vi "FPGA Beam Scanning V2.vi"(1 "Detectors":T1, 2 "Image Acquisition Parameters":T2={"Scan Type"=enum."Sample Scanning", "Scan Mode"=enum."XY", "Fast Axis Frequency (Hz)"=100.0, "Image Format"=128, "Line Accumulations"=1, "Frames Per Capture"=1, "Frames Accumulations"=1, "Image Dimension (um)"=[], "Number of Z Steps"=1, "Z Steps Size (um)"=1.0, "Pixel Size (nm)"=[]} {"Z Steps Size (um)" min=0.0; "Number of Z Steps" min=1; "Frames Accumulations" min=1; "Frames Per Capture" min=1; "Line Accumulations" min=1; "Image Format" items=["64 x 64"=64, "128 x 128"=128, "256 x 256"=256, "512 x 512"=512, "1024 x 1024"=1024, "2048 x 2048"=2048]}) -> ()   [LabVIEW 2016]
uses:
  <vilib>/rvi/interface/nirviReadWriteControl/nirviReadWriteControl.xnode
  <vilib>/rvi/interface/nirviMethod/nirviMethod.xnode
  <vilib>/rvi/errors/niLvFpgaMergeErrorWithErrorCode.vi
  <vilib>/rvi/interface/nirviOpenFPGA/nirviOpenFPGA.xnode
  <vilib>/vision/NI_Vision_Development_Module.lvlib
  <vilib>/rvi/interface/nirviCloseFPGA/nirviCloseFPGA.xnode
  <vilib>/vision/Image Controls.llb/IMAQ Image.ctl
  FPGA Bitfiles/MainSTEDFPGAProj_FPGATarget2_BeamScanningCamb_PyGckhW3v70.lvbitx
  FPGA Target VIs/FPGA-7852R/Beam Scanning Cambridge V1.vi
  NiFpgaLv.dll
  <vilib>/Utility/error.llb/Error Cluster From Error Code.vi
  <vilib>/rvi/errors/niLvFpgaAdjustHostInterfaceError.vi
  <vilib>/FPGAPlugInAG/PCIe-7852R/niLvFpga_ReadFifo_PCIe-7852R.vi
  <vilib>/FPGAPlugInAG/PCIe-7852R/niLvFpga_Close_PCIe-7852R.vi
  <vilib>/FPGAPlugInAG/PCIe-7852R/niLvFpga_Open_PCIe-7852R.vi
  <vilib>/FPGAPlugInAG/PCIe-7852R/niLvFpga_ConfigureFifo_PCIe-7852R.vi
  <vilib>/FPGAPlugInAG/PCIe-7852R/niLvFpga_StartFifo_PCIe-7852R.vi
  <vilib>/FPGAPlugInAG/PCIe-7852R/niLvFpga_Run_PCIe-7852R.vi
  Type Defs/Image Acquisition Parameters.ctl
  Detectors.ctl
panel:
  in  "Adjust Trigger":u16=300
  # "Copyright (C) 2020 Edward S Allgeyer\n\nRedistribution and use in source and binary forms, with or without\nmodification, are permitted provided that the following conditions\nare met:\n\n1. Redistributions of source code must retain the above copyright\n   notice, this list of conditions and the following disclaimer.\n\n2. Redistributions in binary form must reproduce the above copyright\n   notice, this list of conditions and the following disclaimer in\n   the documentation and/or other materials provided with the\n   distribution.\n\n3. Neither the name of the copyright holder nor the names of its\n   contributors may be used to endorse or promote products derived\n   from this software without specific prior written permission.\n\nTHIS SOFTWARE IS PROVIDED BY THE COPYRIGHT HOLDERS AND CONTRIBUTORS\n\"AS IS\" AND ANY EXPRESS OR IMPLIED WARRANTIES, INCLUDING, BUT NOT\nLIMITED TO, THE IMPLIED WARRANTIES OF MERCHANTABILITY AND FITNESS\nFOR A PARTICULAR PURPOSE ARE DISCLAIMED. IN NO EVENT SHALL THE\nCOPYRIGHT HOLDER OR CONTRIBUTORS BE LIABLE FOR ANY DIRECT, INDIRECT,\nINCIDENTAL, SPECIAL, EXEMPLARY, OR CONSEQUENTIAL DAMAGES (INCLUDING,\nBUT NOT LIMITED TO, PROCUREMENT OF SUBSTITUTE GOODS OR SERVICES;\nLOSS OF USE, DATA, OR PROFITS; OR BUSINESS INTERRUPTION) HOWEVER\nCAUSED AND ON ANY THEORY OF LIABILITY, WHETHER IN CONTRACT, STRICT\nLIABILITY, OR TORT (INCLUDING NEGLIGENCE OR OTHERWISE) ARISING IN\nANY WAY OUT OF THE USE OF THIS SOFTWARE, EVEN IF ADVISED OF THE\nPOSSIBILITY OF SUCH DAMAGE."
  # "XY"
  # "Z"
  # "Length"
  # "Height"
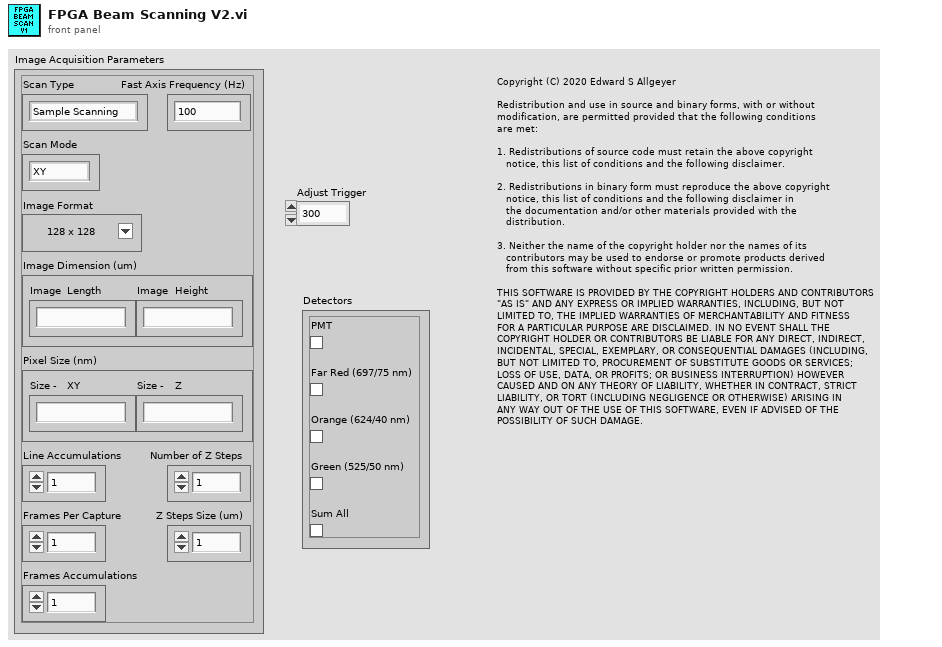
[diagram p1: front panel]
types:
  T1 = typedef "Detectors.ctl" = cluster{"PMT":bool, "Far Red (697/75 nm)":bool, "Orange (624/40 nm)":bool, "Green (525/50 nm)":bool, "Sum All":bool}
  T2 = typedef "Image Acquisition Parameters.ctl" = cluster{"Scan Type":enum16{"Sample Scanning", "Beam Scanning"}, "Scan Mode":enum16{"XY", "XZ", "YZ", "XYZ"}, "Fast Axis Frequency (Hz)":dbl, "Image Format":u16, "Line Accumulations":u16, "Frames Per Capture":u16, "Frames Accumulations":u16, "Image Dimension (um)":dbl[], "Number of Z Steps":u8, "Z Steps Size (um)":dbl, "Pixel Size (nm)":dbl[]}
  T3 = typedef "IMAQ Image.ctl" = refnum<image>
  T4 = enum16{"big-endian, network order", "native, host order", "little-endian"}
  T5 = cluster{"FPGA Sampling Period (ns)":dbl, "Counting Period (us)":dbl, "Samples Per Counting Period":i32, "Start Time (us)":dbl, "Stop Time (us)":dbl, "Normalized Scan End Position":dbl, "Normalized Scan Start Position":dbl}
  T6 = typedef "Scan Parameters.ctl" = cluster{"Fast_Ax_Amp_V":dbl, "Fast_Ax_Off_V":dbl, "Slow_Ax_Amp_V":dbl, "Slow_Ax_Off_V ":dbl, "Slow_Ax_Max_V_VperS":dbl, "Slow_Ax1_Del25ns":i32, "Slow_Ax2_Del25ns":i32, "Stage_X_Off_V":dbl, "Stage_Y_Off_V":dbl, "Stage_Z_Off_V":dbl, "Galvo1_Off_V":dbl, "Galvo2_Off_V":dbl, "Last_Scan_Mode":enum16{"XY", "XZ", "YZ", "XYZ"}, "Current_Scan_Mode":enum16{"XY", "XZ", "YZ", "XYZ"}, "Fly_Back_Lines":u16, "Linear_Ramp_End":u32, "Z_Step_I16":i16, "Z_Start_I16":i16, "Laser_States _U32":u32, "590_Voltage_I16":i16, "775_AOM_Volt_I16":i16, "Blanking OFF":bool, "Unused_Axis_I16":i16}
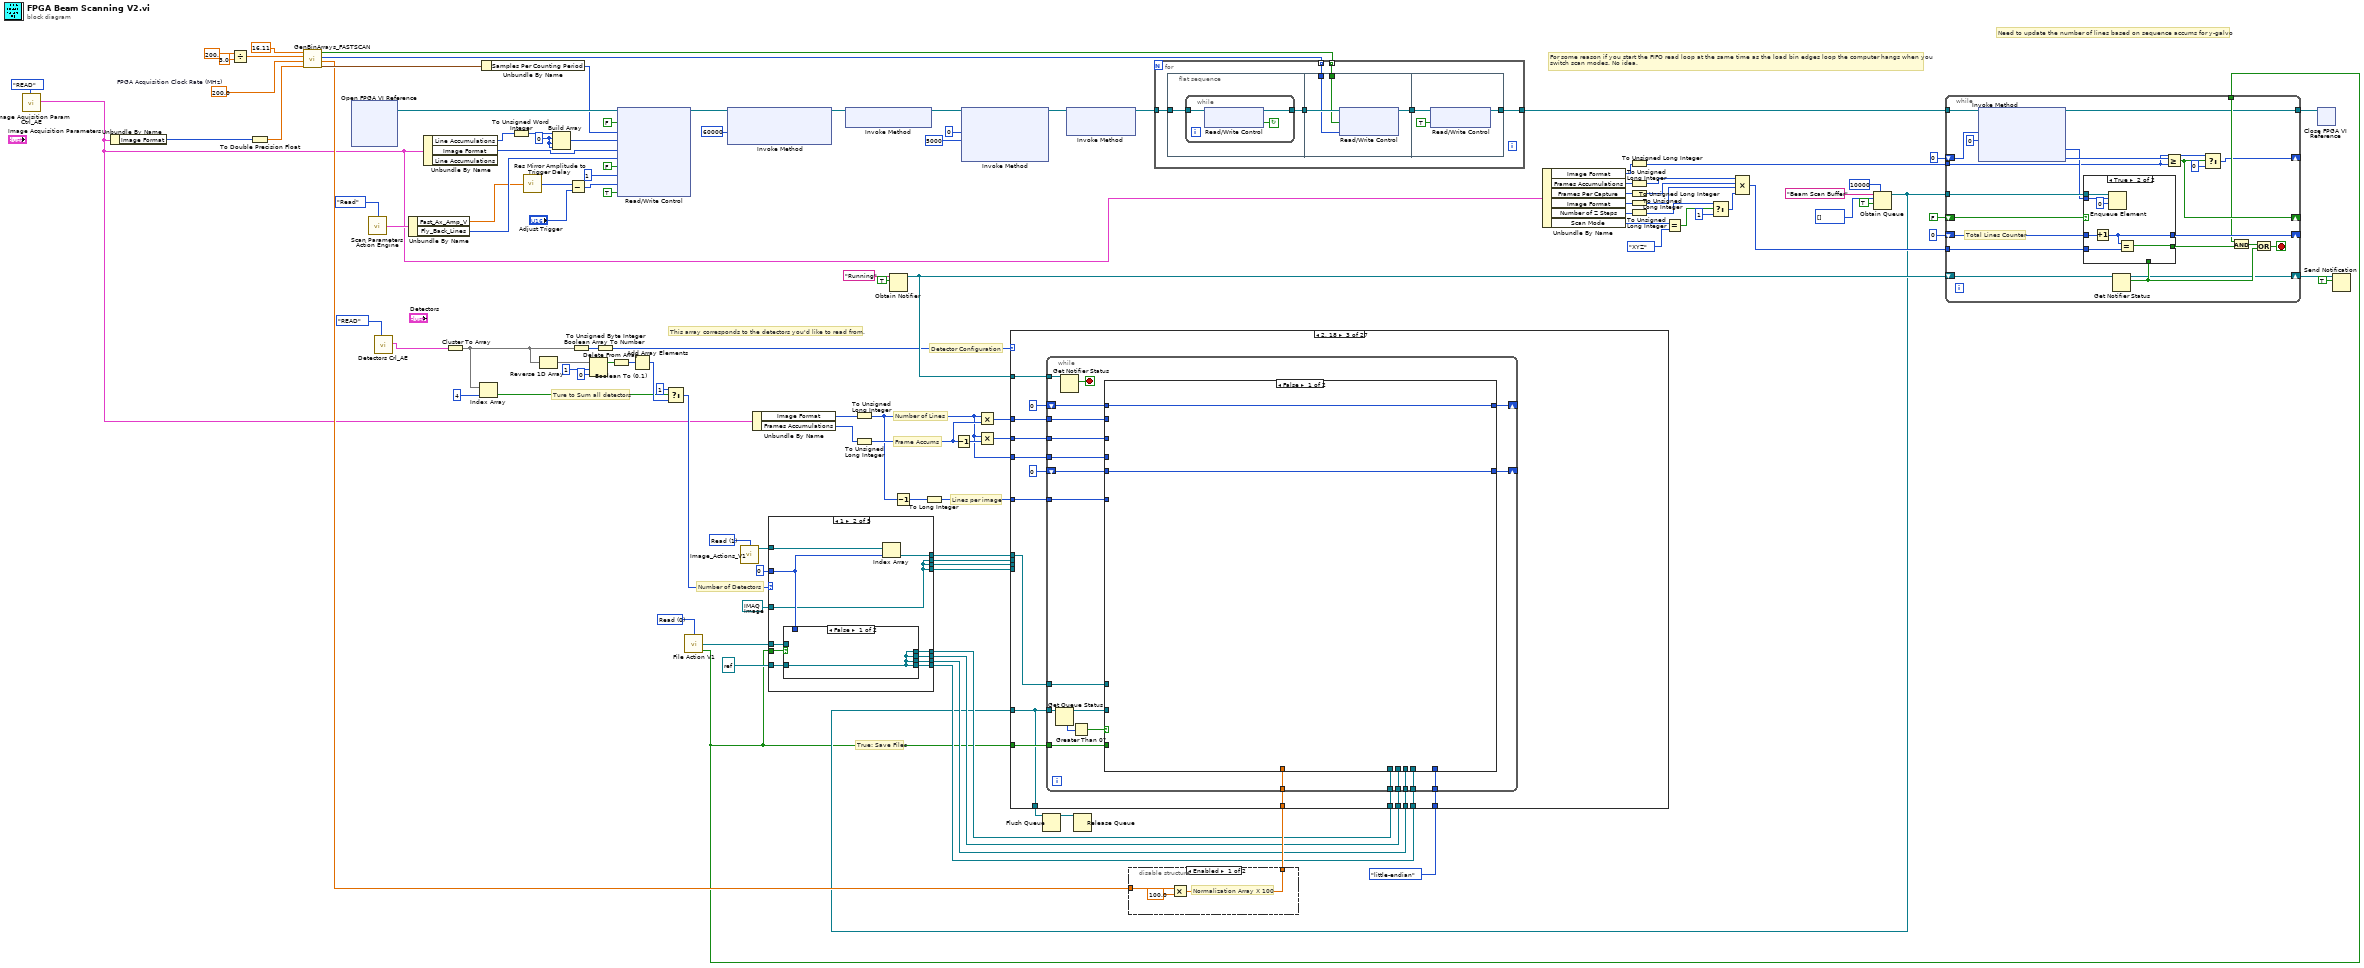
[diagram p0: block diagram]
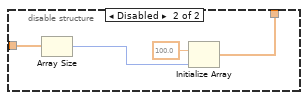
[diagram p2: hidden frame]
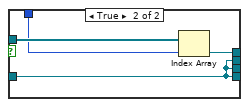
[diagram p4: hidden frame]
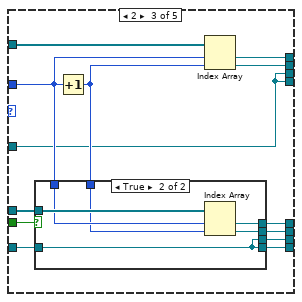
[diagram p5: hidden frame]
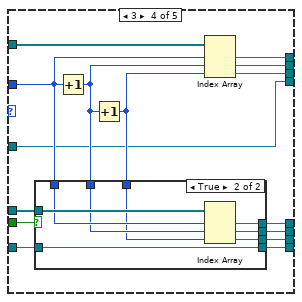
[diagram p7: hidden frame]
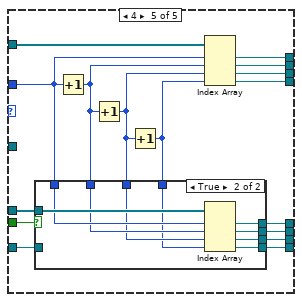
[diagram p9: hidden frame]
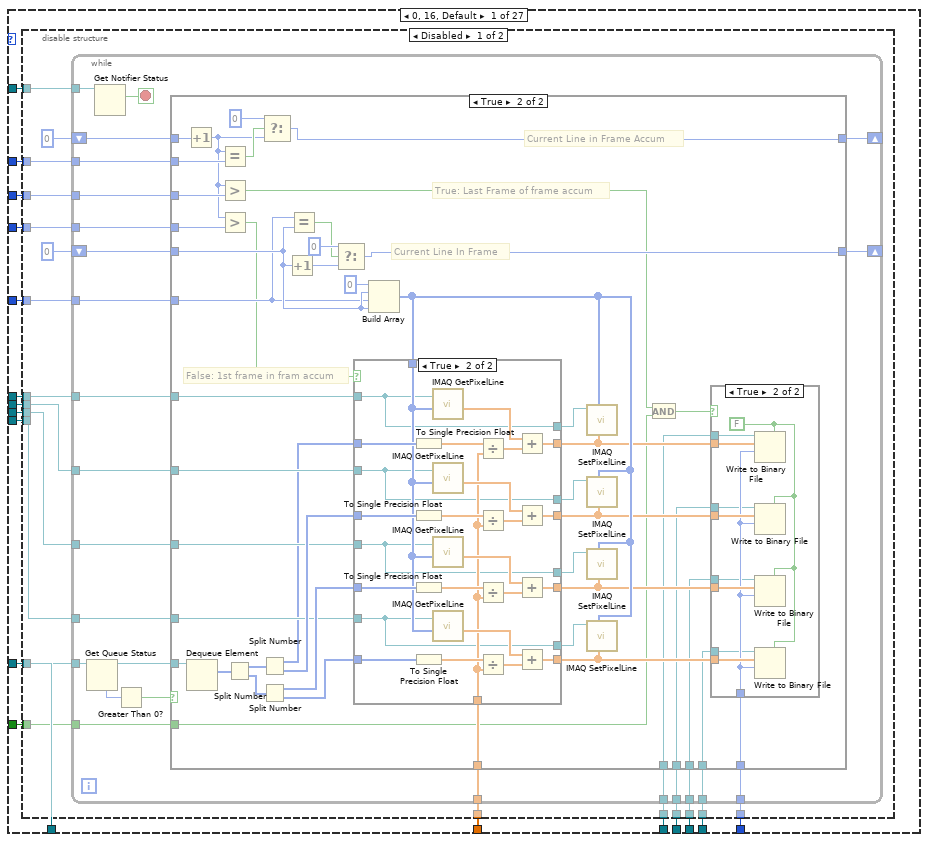
[diagram p11: hidden frame]
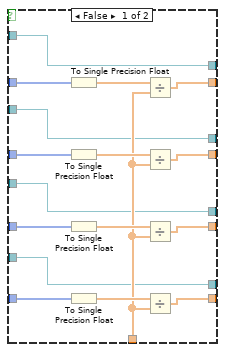
[diagram p14: hidden frame]
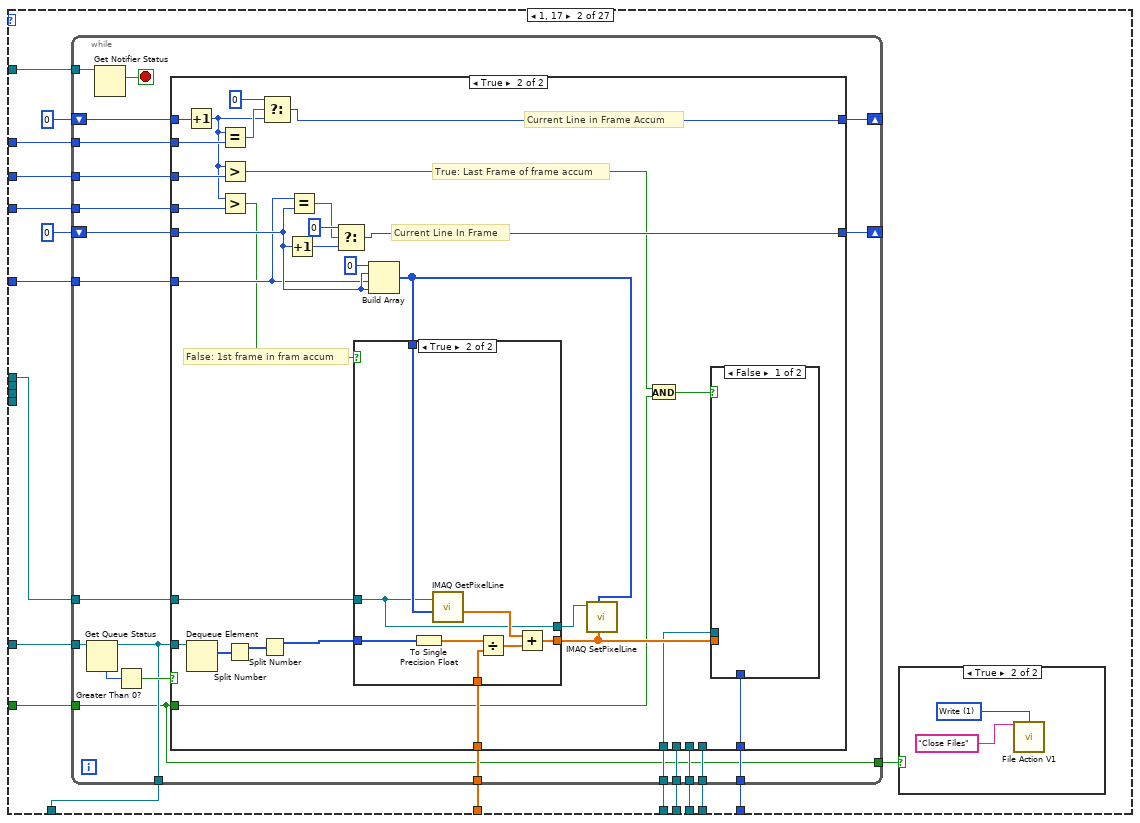
[diagram p16: hidden frame]
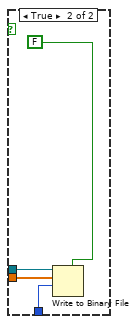
[diagram p19: hidden frame]
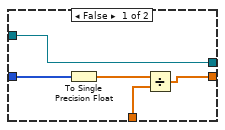
[diagram p20: hidden frame]
diagram:
  w18 = u16 0 items=["Read", "Write"] ("Mode")
  w19 = u16 0 ("element")
  w62 = u16 1 items=["Write", "Read"] ("Mode")
  w110 = 200.0  # FPGA Acquisition Clock Rate (MHz)
  # "This array corresponds to the detectors you'd like to read from."
  # "Ture to Sum all detectors"
  # "Number of Detectors"
  # "Detector Configuration"
  # "Frame Accums"
  # "Number of Lines"
  # "True: Save Files"
  # "Lines per image"
  # "For some reason if you start the FIFO read loop at the same time as the load bin edges loop the computer hangs when you\nswitch scan modes. No idea."
  # "Need to update the number of lines based on sequence accums for y-galvo"
  n1 = call "Image Aquisition Param Ctrl_AE.vi"("Action"=enum16{"READ", "WRITE"}."READ") -> ("Image Acquisition Parameters Out"=w3:T2)  [unwired: 10 in]
  n2 = Unbundle By Name(w3) -> ("Image Format"=w16:u16)
  n3 = Divide(x=200.0, y=3.0) -> (x/y=w107:dbl)
  n4 = To Double Precision Float(number=w16) -> (double precision float=w91:dbl)
  n5 = call "GenBinArrays_FASTSCAN.vi"("Pixels Per Line"=w91, "FPGA Acquisition Clock Rate (MHz)"=w110, "Collection Percent (%)"=w107, "Scan Rate (kHz)"=16.11) -> ("Reported Parameters"=w106:T5, "Normalization Array"=w40:sgl[], "Pre Binned Counts (x100)"=w13:u32[], "FPGA Bin Edges"=w14:bool[])
  n6 = xnode "Open FPGA VI Reference"() -> ("FPGA VI Reference Out"=w114:refnum<k20>)  [unwired: 2 in, 1 out]
  n7 = call "Scan Parameters Action Engine.vi"("Action"=enum16{"Read", "Write"}."Read") -> ("Scan Parameters OUT"=w24:T6)  [unwired: 14 in]
  n8 = call "Detectors Crl_AE.vi"("Action"=enum16{"READ", "WRITE"}."READ") -> ("Detectors Parameters Out"=w1:T1)  [unwired: 10 in]
  n9 = Unbundle By Name(w24) -> ("Fast_Ax_Amp_V"=w15:dbl, "Fly_Back_Lines"=w23:u16)
  n10 = Unbundle By Name(w3) -> ("Line Accumulations"=w29:u16, "Image Format"=w26:u16)  [unwired: 1 out]
  n11 = Cluster To Array(cluster=w1) -> (array=w7:bool[])
  n12 = Index Array(array=w7, index=4) -> (element=w5:bool)
  n13 = Unbundle By Name(w106) -> ("Samples Per Counting Period"=w73:i32)
  n14 = To Unsigned Word Integer(number=w29) -> (unsigned 16bit integer=w28:u16)
  n15 = call "Res Mirror Amplitude to Trigger Delay.vi"("Amplitude (V)"=w15) -> ("Trigger Delay (Ticks)"=w12:u16)
  n16 = Reverse 1D Array(array=w7) -> (reversed array=w45:bool[])
  n17 = Build Array(w28, w19, w19, w19) -> (w27:u16[])
  n18 = Subtract(x=w12, y="Adjust Trigger") -> (x-y=w11:u16)
  n19 = Boolean Array To Number(Boolean array=w7) -> (number=w9:u32)
  n20 = Delete From Array(array=w45, length=1, index=0) -> (array with subset deleted=w49:bool[])  [unwired: 1 out]
  n21 = To Unsigned Byte Integer(number=w9) -> (unsigned 8bit integer=w8:u8)
  n22 = Boolean To (0,1)(Boolean=w49) -> (0, 1=w48:i16[])
  n23 = xnode "Read/Write Control"("FPGA VI Reference In"=w114, "Ready For Write"=FALSE, "FPGA Samples"=w73, "Accums Per Line"=w27, "Lines Per Image"=w26, "Dead Lines"=w23, "Line Trigger"=FALSE, "Sequences"=u8 1, "Trigger Delay (Ticks)"=w11, "Stop Acquisition"=TRUE) -> ("FPGA VI Reference Out"=w113:refnum<k20>)  [unwired: 1 in, 1 out]
  n24 = Add Array Elements(numeric array=w48) -> (sum=w47:i16)
  n25 = Select(t=i16 1, s=w5, f=w47) -> (s? t:f=w42:i16)
  n26 = call "File Action V1.vi"("Mode"=w18) -> ("File REFs"=w59:refnum<file>[], "Files Open"=w17:bool)  [unwired: 12 in, 1 out]
  n27 = xnode "Invoke Method"("FPGA VI Reference In"=w113, "Requested Depth"=u32 60000) -> ("FPGA VI Reference Out"=w89:refnum<k20>)  [unwired: 1 in, 2 out]
  n28 = call "Image_Actions_V1.vi"("Mode"=w62) -> ("Image REFs OUT"=w61:T3[])  [unwired: 13 in, 1 out]
  n29 = Unbundle By Name(w3) -> ("Image Format"=w82:u16, "Frames Accumulations"=w81:u16)
  n30 = case shown="1" w42 {
    tunnel: [w116 w117 w133 w153 w192] -> w54
    tunnel: [w116 w117 w133 w167 w191] -> w55
    tunnel: [w116 w117 w145 w166 w190] -> w56
    tunnel: [w116 w127 w144 w165 w189] -> w57
    tunnel: 0 ("Offset") -> [_ w123 w140 w161 w185]
    tunnel: w61 -> [_ w126 w143 w164 w188]
    tunnel: T3 refnum ("New Image") -> [w116 w117 w133 w153 _]
    tunnel: w59 -> [_ w124 w141 w162 w186]
    tunnel: w17 -> [_ w125 w142 w163 w187]
    tunnel: [w115 w122 w138 w158 w181] -> w53
    tunnel: [w115 w121 w137 w157 w180] -> w52
    tunnel: [w115 w120 w136 w156 w179] -> w51
    tunnel: [w115 w119 w135 w155 w178] -> w50
    tunnel: refnum<file> refnum ("element") -> [w115 w118 w134 w154 w177]
    frame 0, Default {
    }
    frame 1 {
      n31 = case shown="False" w125 {
        tunnel: w124 -> [_ w132]
        tunnel: w123 -> [_ w131]
        tunnel: [w128 w130] -> w122
        tunnel: [w128 w129] -> w121
        tunnel: [w128 w129] -> w120
        tunnel: [w128 w129] -> w119
        tunnel: w118 -> [w128 w129]
        frame False {
        }
        frame True {
          n32 = Index Array(array=w132, index=w131) -> (element=w130:refnum<file>)
        }
      }
      n33 = Index Array(array=w126, index=w123) -> (element=w127:T3)
    }
    frame 2 {
      n34 = Increment(x=w140) -> (x+1=w139:i32)
      n35 = case shown="True" w142 {
        tunnel: w141 -> [_ w152]
        tunnel: w140 -> [_ w151]
        tunnel: w139 -> [_ w150]
        tunnel: [w146 w149] -> w138
        tunnel: [w146 w148] -> w137
        tunnel: [w146 w147] -> w136
        tunnel: [w146 w147] -> w135
        tunnel: w134 -> [w146 w147]
        frame False {
        }
        frame True {
          n36 = Index Array(array=w152, index #1=w151, index #2=w150) -> (element #1=w149:refnum<file>, element #2=w148:refnum<file>)
        }
      }
      n37 = Index Array(array=w143, index #1=w140, index #2=w139) -> (element #1=w144:T3, element #2=w145:T3)
    }
    frame 3 {
      n38 = Increment(x=w161) -> (x+1=w160:i32)
      n39 = Increment(x=w160) -> (x+1=w159:i32)
      n40 = case shown="True" w163 {
        tunnel: w162 -> [_ w176]
        tunnel: w161 -> [_ w175]
        tunnel: w160 -> [_ w174]
        tunnel: w159 -> [_ w173]
        tunnel: [w168 w172] -> w158
        tunnel: [w168 w171] -> w157
        tunnel: [w168 w170] -> w156
        tunnel: [w168 w169] -> w155
        tunnel: w154 -> [w168 w169]
        frame False {
        }
        frame True {
          n41 = Index Array(array=w176, index #1=w175, index #2=w174, index #3=w173) -> (element #1=w172:refnum<file>, element #2=w171:refnum<file>, element #3=w170:refnum<file>)
        }
      }
      n42 = Index Array(array=w164, index #1=w161, index #2=w160, index #3=w159) -> (element #1=w165:T3, element #2=w166:T3, element #3=w167:T3)
    }
    frame 4 {
      n43 = Increment(x=w185) -> (x+1=w184:i32)
      n44 = Increment(x=w184) -> (x+1=w183:i32)
      n45 = Increment(x=w183) -> (x+1=w182:i32)
      n46 = case shown="True" w187 {
        tunnel: w186 -> [_ w202]
        tunnel: w185 -> [_ w201]
        tunnel: w184 -> [_ w200]
        tunnel: w183 -> [_ w199]
        tunnel: w182 -> [_ w198]
        tunnel: [w193 w197] -> w181
        tunnel: [w193 w196] -> w180
        tunnel: [w193 w195] -> w179
        tunnel: [w193 w194] -> w178
        tunnel: w177 -> [w193 _]
        frame False {
        }
        frame True {
          n47 = Index Array(array=w202, index #1=w201, index #2=w200, index #3=w199, index #4=w198) -> (element #1=w197:refnum<file>, element #2=w196:refnum<file>, element #3=w195:refnum<file>, element #4=w194:refnum<file>)
        }
      }
      n48 = Index Array(array=w188, index #1=w185, index #2=w184, index #3=w183, index #4=w182) -> (element #1=w189:T3, element #2=w190:T3, element #3=w191:T3, element #4=w192:T3)
    }
  }
  n49 = xnode "Invoke Method"("FPGA VI Reference In"=w89) -> ("FPGA VI Reference Out"=w90:refnum<k20>)  [unwired: 1 in, 1 out]
  n50 = To Unsigned Long Integer(number=w82) -> (unsigned 32bit integer=w65:u32)
  n51 = To Unsigned Long Integer(number=w81) -> (unsigned 32bit integer=w66:u32)
  n52 = Obtain Notifier(name (unnamed)="Running", notification data type=TRUE) -> (notifier out=w39:refnum<notifier>)  [unwired: 2 in, 2 out]
  n53 = Decrement(x=w65) -> (x-1=w63:u32)
  n54 = To Long Integer(number=w63) -> (32bit integer=w71:i32)
  n55 = Decrement(x=w66) -> (x-1=w69:u32)
  n56 = xnode "Invoke Method"("FPGA VI Reference In"=w90, "Number of Elements"=u32 0, "Timeout (ms)"=5000) -> ("FPGA VI Reference Out"=w112:refnum<k20>)  [unwired: 1 in, 3 out]
  n57 = Multiply(x=w65, y=w66) -> (x*y=w67:u32)
  n58 = Multiply(x=w65, y=w69) -> (x*y=w68:u32)
  n59 = xnode "Invoke Method"("FPGA VI Reference In"=w112) -> ("FPGA VI Reference Out"=w105:refnum<k20>)  [unwired: 2 in, 1 out]
  n60 = disable-structure shown="Enabled" {
    disable-tunnel: [w205 w206] -> w80
    disable-tunnel: w40 -> [w203 w209]
    frame Enabled {
      # "Normalization Array X 100"
      n61 = Multiply(x=w203, y=sgl 100.0) -> (x*y=w205:sgl[])
    }
    frame Disabled {
      n62 = Array Size(array=w209) -> (size(s)=w208:i32)
      n63 = Initialize Array(sgl 100.0 ("element"), w208) -> (w206:sgl[])
    }
  }
  n64 = for {
    tunnel: [w213] -> w78
    tunnel: w105 -> [w212]
    tunnel: w14 -> [w211] mode=indexing
    tunnel: w13 -> [w210] mode=indexing
    n65 = flat-sequence {
      tunnel: [w217] -> w215
      tunnel: w212 -> [w216]
      tunnel: w215 -> [w224]
      tunnel: [w223] -> w214
      tunnel: w211 -> [w222]
      tunnel: w210 -> [w221]
      tunnel: w214 -> [w227]
      tunnel: [w226] -> w213
      frame #0 {
        n66 = while {
          tunnel: [w220] -> w217
          tunnel: w216 -> [w219]
          stop <- w218 continue-if-true
          n67 = xnode "Read/Write Control"("FPGA VI Reference In"=w219) -> ("FPGA VI Reference Out"=w220:refnum<k20>, "Ready For Write"=w218:bool)  [unwired: 1 in, 1 out]
        }
      }
      frame #1 {
        n68 = xnode "Read/Write Control"("FPGA VI Reference In"=w224, "BinEdge"=w222, "PreBinnedValue"=w221) -> ("FPGA VI Reference Out"=w223:refnum<k20>)  [unwired: 1 in, 1 out]
      }
      frame #2 {
        n69 = xnode "Read/Write Control"("FPGA VI Reference In"=w227, "Ready For Write"=TRUE) -> ("FPGA VI Reference Out"=w226:refnum<k20>)  [unwired: 1 in, 1 out]
      }
    }
  }
  n70 = Unbundle By Name(w3) -> ("Image Format"=w97:u16, "Frames Accumulations"=w37:u16, "Frames Per Capture"=w98:u16, "Image Format"=w38:u16, "Number of Z Steps"=w34:u8, "Scan Mode"=w35:enum16{"XY", "XZ", "YZ", "XYZ"})
  n71 = To Unsigned Long Integer(number=w97) -> (unsigned 32bit integer=w104:u32)
  n72 = To Unsigned Long Integer(number=w37) -> (unsigned 32bit integer=w33:u32)
  n73 = To Unsigned Long Integer(number=w98) -> (unsigned 32bit integer=w32:u32)
  n74 = To Unsigned Long Integer(number=w38) -> (unsigned 32bit integer=w31:u32)
  n75 = To Unsigned Long Integer(number=w34) -> (unsigned 32bit integer=w30:u32)
  n76 = Equal?(x=w35, y=enum16{"XY", "XZ", "YZ", "XYZ"}."XYZ") -> (x = y?=w85:bool)
  n77 = Select(t=w30, s=w85, f=u32 1) -> (s? t:f=w84:u32)
  n78 = Compound Arithmetic op=MULTIPLY(w33, w32, w31, w84) -> (w99:u32)
  n79 = Obtain Queue(max queue size (-1, unlimited)=10000, name (unnamed)="Beam Scan Buffer", element data type=u64[] [], create if not found? (T)=TRUE) -> (queue out=w21:refnum<queue>)  [unwired: 1 in, 2 out]
  n80 = case shown="2, 18" w8 {
    tunnel: w71 -> [w244 w406 w495 w584 w689 w777 w884 w992 w1116 w1204 w1311 w1419 w1544 w1651 w1777 w1904 w2046 w2135 w2225 w2315 w2407 w2497 w2587 w2679 w2768 w2860 w2952]
    tunnel: w17 -> [w241 w403 w492 w581 w686 w774 w881 w989 w1113 w1201 w1308 w1416 w1541 w1648 w1774 w1901 w2043 w2132 w2222 w2312 w2404 w2494 w2584 w2676 w2765 w2857 w2949]
    tunnel: T4."little-endian" ("byte order (0:big-endian, network order)") -> [w243 w405 w494 w583 w688 w776 w883 w991 w1115 w1203 w1310 w1418 w1543 w1650 w1776 w1903 w2045 w2134 w2224 w2314 w2406 w2496 w2586 w2678 w2767 w2859 w2951]
    tunnel: w80 -> [w242 w404 w493 w582 w687 w775 w882 w990 w1114 w1202 w1309 w1417 w1542 w1649 w1775 w1902 w2044 w2133 w2223 w2313 w2405 w2495 w2585 w2677 w2766 w2858 w2950]
    tunnel: w39 -> [w240 w402 w491 w580 w685 w773 w880 w988 w1112 w1200 w1307 w1415 w1540 w1647 w1773 w1900 w2042 w2131 w2221 w2311 w2403 w2493 w2583 w2675 w2764 w2856 w2948]
    tunnel: w68 -> [w239 w400 w489 w578 w683 w771 w878 w986 w1110 w1198 w1305 w1413 w1538 w1645 w1771 w1898 w2040 w2129 w2219 w2309 w2401 w2491 w2581 w2673 w2762 w2854 w2946]
    tunnel: w67 -> [w238 w399 w488 w577 w682 w770 w877 w985 w1109 w1197 w1304 w1412 w1537 w1644 w1770 w1897 w2039 w2128 w2218 w2308 w2400 w2490 w2580 w2672 w2761 w2853 w2945]
    tunnel: w65 -> [w237 w398 w487 w576 w681 w769 w876 w984 w1108 w1196 w1303 w1411 w1536 w1643 w1769 w1896 w2038 w2127 w2217 w2307 w2399 w2489 w2579 w2671 w2760 w2852 w2944]
    tunnel: w21 -> [w236 w397 w486 w569 w680 w768 w875 w983 w1107 w1195 w1302 w1410 w1535 w1642 w1768 w1895 w2037 w2126 w2216 w2306 w2398 w2488 w2578 w2670 w2759 w2851 w2943]
    tunnel: w57 -> [w231 w392 w481 w571 w675 w763 w870 w978 w1102 w1190 w1297 w1405 w1530 w1637 w1763 w1890 w2032 w2121 w2211 w2301 w2393 w2483 w2573 w2665 w2754 w2846 w2938]
    tunnel: w56 -> [w230 _ _ w570 _ w762 w869 w977 _ w1189 w1296 w1404 w1529 w1636 w1762 w1889 _ _ _ _ _ _ _ _ _ _ _]
    tunnel: w55 -> [w229 _ _ _ _ _ _ w976 _ _ _ w1403 _ w1635 w1761 w1888 _ _ _ _ _ _ _ _ _ _ _]
    tunnel: w54 -> [w228 _ _ _ _ _ _ _ _ _ _ _ _ _ _ w1887 _ _ _ _ _ _ _ _ _ _ _]
    tunnel: [w236 w391 w486 w568 w680 w768 w875 w983 w1107 w1195 w1302 w1410 w1535 w1642 w1768 w1895 w2037 w2126 w2216 w2306 w2398 w2488 w2578 w2670 w2759 w2851 w2943] -> w20
    tunnel: w53 -> [w235 w396 w485 w575 w679 w767 w874 w982 w1106 w1194 w1301 w1409 w1534 w1641 w1767 w1894 w2036 w2125 w2215 w2305 w2397 w2487 w2577 w2669 w2758 w2850 w2942]
    tunnel: w52 -> [w234 w395 w484 w574 w678 w766 w873 w981 w1105 w1193 w1300 w1408 w1533 w1640 w1766 w1893 w2035 w2124 w2214 w2304 w2396 w2486 w2576 w2668 w2757 w2849 w2941]
    tunnel: w51 -> [w233 w394 w483 w573 w677 w765 w872 w980 w1104 w1192 w1299 w1407 w1532 w1639 w1765 w1892 w2034 w2123 w2213 w2303 w2395 w2485 w2575 w2667 w2756 w2848 w2940]
    tunnel: w50 -> [w232 w393 w482 w572 w676 w764 w871 w979 w1103 w1191 w1298 w1406 w1531 w1638 w1764 w1891 w2033 w2122 w2212 w2302 w2394 w2484 w2574 w2666 w2755 w2847 w2939]
    frame 0, 16, Default {
      n81 = disable-structure shown="Disabled" {
        disable-tunnel: w244 -> [w262 _]
        disable-tunnel: w243 -> [w261 _]
        disable-tunnel: w242 -> [w260 _]
        disable-tunnel: w241 -> [w259 _]
        disable-tunnel: w240 -> [w258 _]
        disable-tunnel: w239 -> [w256 _]
        disable-tunnel: w238 -> [w255 _]
        disable-tunnel: w237 -> [w254 _]
        disable-tunnel: w236 -> [w253 _]
        disable-tunnel: w235 -> [w252 _]
        disable-tunnel: w234 -> [w251 _]
        disable-tunnel: w233 -> [w250 _]
        disable-tunnel: w232 -> [w249 _]
        disable-tunnel: w231 -> [w248 _]
        disable-tunnel: w230 -> [w247 _]
        disable-tunnel: w229 -> [w246 _]
        disable-tunnel: w228 -> [w245 _]
        frame Disabled {
          n82 = while {
            shift-right: [w286] -> _
            shift-left: 0 -> [w287]
            tunnel: w262 -> [w288]
            tunnel: w261 -> [w285]
            tunnel: w260 -> [w284]
            tunnel: w259 -> [w283]
            tunnel: w258 -> [w279]
            shift-right: [w276] -> _
            shift-left: u32 0 -> [w277]
            tunnel: w256 -> [w275]
            tunnel: w255 -> [w274]
            tunnel: w254 -> [w273]
            tunnel: w253 -> [w272]
            tunnel: w248 -> [w271]
            tunnel: w247 -> [w270]
            tunnel: w246 -> [w269]
            tunnel: w245 -> [w268]
            tunnel: w252 -> [w267]
            tunnel: w251 -> [w266]
            tunnel: w250 -> [w265]
            tunnel: w249 -> [w264]
            stop <- w278 stop-if-true
            n83 = Get Queue Status(queue=w272) -> (queue out=w280:refnum<queue>, # elements in queue=w282:i32)  [unwired: 2 in, 6 out]
            n84 = Get Notifier Status(notifier=w279) -> (current notification=w278:bool)  [unwired: 1 in, 4 out]
            n85 = Greater Than 0?(x=w282) -> (x > 0?=w281:bool)
            n86 = case shown="True" w281 {
              tunnel: w288 -> [_ w325]
              tunnel: w287 -> [w290 w326]
              tunnel: [w290 w324] -> w286
              tunnel: w285 -> [_ w318]
              tunnel: w284 -> [_ w317]
              tunnel: w283 -> [_ w307]
              tunnel: w280 -> [_ w316]
              tunnel: w277 -> [w289 w313]
              tunnel: [w289 w312] -> w276
              tunnel: w275 -> [_ w311]
              tunnel: w274 -> [_ w310]
              tunnel: w273 -> [_ w305]
              tunnel: w271 -> [_ w303]
              tunnel: w270 -> [_ w302]
              tunnel: w269 -> [_ w301]
              tunnel: w268 -> [_ w300]
              tunnel: w267 -> [_ w294]
              tunnel: w266 -> [_ w293]
              tunnel: w265 -> [_ w292]
              tunnel: w264 -> [_ w291]
              frame False {
              }
              frame True {
                # "False: 1st frame in fram accum"
                # "True: Last Frame of frame accum"
                # "Current Line in Frame Accum"
                # "Current Line In Frame"
                n87 = Increment(x=w313) -> (x+1=w306:u32)
                n88 = Dequeue Element(queue=w316) -> (element=w335:u64[])  [unwired: 2 in, 3 out]
                n89 = Equal?(x=w306, y=w310) -> (x = y?=w315:bool)
                n90 = Greater?(x=w306, y=w311) -> (0:w308:bool)
                n91 = Greater?(x=w306, y=w305) -> (0:w304:bool)
                n92 = Split Number(x=w335) -> (hi(x)=w336:u32[], lo(x)=w334:u32[])
                n93 = Split Number(x=w336) -> (hi(x)=w295:u16[], lo(x)=w333:u16[])
                n94 = Split Number(x=w334) -> (hi(x)=w332:u16[], lo(x)=w331:u16[])
                n95 = Select(t=u32 0, s=w315, f=w306) -> (s? t:f=w312:u32)
                n96 = Increment(x=w326) -> (x+1=w328:i32)
                n97 = Equal?(x=w325, y=w326) -> (x = y?=w327:bool)
                n98 = Select(t=0, s=w327, f=w328) -> (s? t:f=w324:i32)
                n99 = Build Array(0, w326, w325, w326) -> (w323:i32[])
                n100 = case shown="True" w304 {
                  tunnel: w295 -> [w362 w389]
                  tunnel: w333 -> [w357 w388]
                  tunnel: w332 -> [w356 w387]
                  tunnel: w331 -> [w355 w386]
                  tunnel: [w353 w378] -> w320
                  tunnel: [w354 w377] -> w321
                  tunnel: [w361 w376] -> w322
                  tunnel: [w352 w375] -> w319
                  tunnel: w323 -> [_ w370]
                  tunnel: w317 -> [w351 w368]
                  tunnel: w303 -> [w350 w365]
                  tunnel: w302 -> [w349 w366]
                  tunnel: w301 -> [w348 w367]
                  tunnel: w300 -> [w347 w364]
                  tunnel: [w348 w367] -> w297
                  tunnel: [w349 w366] -> w298
                  tunnel: [w350 w365] -> w299
                  tunnel: [w347 w364] -> w296
                  frame False {
                    n101 = To Single Precision Float(number=w362) -> (single precision float=w363:sgl[])
                    n102 = To Single Precision Float(number=w357) -> (single precision float=w360:sgl[])
                    n103 = To Single Precision Float(number=w356) -> (single precision float=w359:sgl[])
                    n104 = To Single Precision Float(number=w355) -> (single precision float=w358:sgl[])
                    n105 = Divide(x=w363, y=w351) -> (x/y=w361:sgl[])
                    n106 = Divide(x=w360, y=w351) -> (x/y=w354:sgl[])
                    n107 = Divide(x=w359, y=w351) -> (x/y=w353:sgl[])
                    n108 = Divide(x=w358, y=w351) -> (x/y=w352:sgl[])
                  }
                  frame True {
                    n109 = To Single Precision Float(number=w389) -> (single precision float=w369:sgl[])
                    n110 = To Single Precision Float(number=w388) -> (single precision float=w385:sgl[])
                    n111 = To Single Precision Float(number=w387) -> (single precision float=w384:sgl[])
                    n112 = To Single Precision Float(number=w386) -> (single precision float=w383:sgl[])
                    n113 = call "IMAQ GetPixelLine"("Line Coordinates"=w370, "Image"=w365) -> ("Pixels Line (Float)"=w374:sgl[])  [unwired: 2 in, 4 out]
                    n114 = call "IMAQ GetPixelLine"("Line Coordinates"=w370, "Image"=w366) -> ("Pixels Line (Float)"=w373:sgl[])  [unwired: 2 in, 4 out]
                    n115 = call "IMAQ GetPixelLine"("Line Coordinates"=w370, "Image"=w367) -> ("Pixels Line (Float)"=w372:sgl[])  [unwired: 2 in, 4 out]
                    n116 = call "IMAQ GetPixelLine"("Line Coordinates"=w370, "Image"=w364) -> ("Pixels Line (Float)"=w371:sgl[])  [unwired: 2 in, 4 out]
                    n117 = Divide(x=w369, y=w368) -> (x/y=w382:sgl[])
                    n118 = Divide(x=w385, y=w368) -> (x/y=w381:sgl[])
                    n119 = Divide(x=w384, y=w368) -> (x/y=w380:sgl[])
                    n120 = Divide(x=w383, y=w368) -> (x/y=w379:sgl[])
                    n121 = Add(x=w374, y=w382) -> (x+y=w376:sgl[])
                    n122 = Add(x=w373, y=w381) -> (x+y=w377:sgl[])
                    n123 = Add(x=w372, y=w380) -> (x+y=w378:sgl[])
                    n124 = Add(x=w371, y=w379) -> (x+y=w375:sgl[])
                  }
                }
                n125 = call "IMAQ SetPixelLine"("Pixels Line (Float)"=w322, "Line Coordinates"=w323, "Image"=w299) -> ()  [unwired: 7 in, 2 out]
                n126 = call "IMAQ SetPixelLine"("Pixels Line (Float)"=w321, "Line Coordinates"=w323, "Image"=w298) -> ()  [unwired: 7 in, 2 out]
                n127 = call "IMAQ SetPixelLine"("Pixels Line (Float)"=w320, "Line Coordinates"=w323, "Image"=w297) -> ()  [unwired: 7 in, 2 out]
                n128 = call "IMAQ SetPixelLine"("Pixels Line (Float)"=w319, "Line Coordinates"=w323, "Image"=w296) -> ()  [unwired: 7 in, 2 out]
                n129 = And(x=w308, y=w307) -> (x .and. y?=w309:bool)
                n130 = case shown="True" w309 {
                  tunnel: w322 -> [_ w346]
                  tunnel: w321 -> [_ w345]
                  tunnel: w320 -> [_ w344]
                  tunnel: w319 -> [_ w343]
                  tunnel: w318 -> [_ w341]
                  tunnel: w294 -> [_ w340]
                  tunnel: w293 -> [_ w339]
                  tunnel: w292 -> [_ w338]
                  tunnel: w291 -> [_ w337]
                  frame False {
                  }
                  frame True {
                    w342 = FALSE ("prepend array or string size? (T)")
                    n131 = Write to Binary File(file (use dialog)=w340, data=w346, 5:w342, 9:w341) -> ()  [unwired: 2 in, 3 out]
                    n132 = Write to Binary File(file (use dialog)=w339, data=w345, 5:w342, 9:w341) -> ()  [unwired: 2 in, 3 out]
                    n133 = Write to Binary File(file (use dialog)=w338, data=w344, 5:w342, 9:w341) -> ()  [unwired: 2 in, 3 out]
                    n134 = Write to Binary File(file (use dialog)=w337, data=w343, 5:w342, 9:w341) -> ()  [unwired: 2 in, 3 out]
                  }
                }
              }
            }
          }
        }
        frame Enabled {
        }
      }
    }
    frame 1, 17 {
      n135 = while {
        shift-right: [w429] -> _
        shift-left: 0 -> [w430]
        tunnel: w406 -> [w431]
        tunnel: w405 -> [w428]
        tunnel: w404 -> [w427]
        tunnel: w403 -> [w410]
        tunnel: w402 -> [w424]
        shift-right: [w421] -> _
        shift-left: u32 0 -> [w422]
        tunnel: w400 -> [w420]
        tunnel: w399 -> [w419]
        tunnel: w398 -> [w418]
        tunnel: w397 -> [w417]
        tunnel: w392 -> [w416]
        tunnel: w396 -> [w415]
        tunnel: w395 -> [w414]
        tunnel: w394 -> [w413]
        tunnel: w393 -> [w412]
        tunnel: [w411] -> w391
        tunnel: [w410] -> w390
        stop <- w423 stop-if-true
        n136 = Get Queue Status(queue=w417) -> (queue out=w411:refnum<queue>, # elements in queue=w426:i32)  [unwired: 2 in, 6 out]
        n137 = Get Notifier Status(notifier=w424) -> (current notification=w423:bool)  [unwired: 1 in, 4 out]
        n138 = Greater Than 0?(x=w426) -> (x > 0?=w425:bool)
        n139 = case shown="True" w425 {
          tunnel: w431 -> [_ w456]
          tunnel: w430 -> [w433 w457]
          tunnel: [w433 w455] -> w429
          tunnel: w428 -> [_ w452]
          tunnel: w427 -> [_ w451]
          tunnel: w410 -> [_ w434]
          tunnel: w411 -> [_ w450]
          tunnel: w422 -> [w432 w447]
          tunnel: [w432 w446] -> w421
          tunnel: w420 -> [_ w445]
          tunnel: w419 -> [_ w444]
          tunnel: w418 -> [_ w440]
          tunnel: w416 -> [_ w438]
          tunnel: w415 -> [_ w436]
          tunnel: w414 -> [_ _]
          tunnel: w413 -> [_ _]
          tunnel: w412 -> [_ _]
          frame False {
          }
          frame True {
            # "False: 1st frame in fram accum"
            # "True: Last Frame of frame accum"
            # "Current Line in Frame Accum"
            # "Current Line In Frame"
            n140 = Increment(x=w447) -> (x+1=w441:u32)
            n141 = Dequeue Element(queue=w450) -> (element=w462:u64[])  [unwired: 2 in, 3 out]
            n142 = Equal?(x=w441, y=w444) -> (x = y?=w449:bool)
            n143 = Greater?(x=w441, y=w445) -> (0:w442:bool)
            n144 = Greater?(x=w441, y=w440) -> (0:w439:bool)
            n145 = Split Number(x=w462) -> (hi(x)=w463:u32[])  [unwired: 1 out]
            n146 = Split Number(x=w463) -> (hi(x)=w435:u16[])  [unwired: 1 out]
            n147 = Select(t=u32 0, s=w449, f=w441) -> (s? t:f=w446:u32)
            n148 = Increment(x=w457) -> (x+1=w459:i32)
            n149 = Equal?(x=w456, y=w457) -> (x = y?=w458:bool)
            n150 = Select(t=0, s=w458, f=w459) -> (s? t:f=w455:i32)
            n151 = Build Array(0, w457, w456, w457) -> (w454:i32[])
            n152 = case shown="True" w439 {
              tunnel: w435 -> [w471 w480]
              tunnel: [w470 w477] -> w453
              tunnel: w454 -> [_ w475]
              tunnel: w451 -> [w469 w474]
              tunnel: w438 -> [w468 w473]
              tunnel: [w468 w473] -> w437
              frame False {
                n153 = To Single Precision Float(number=w471) -> (single precision float=w472:sgl[])
                n154 = Divide(x=w472, y=w469) -> (x/y=w470:sgl[])
              }
              frame True {
                n155 = To Single Precision Float(number=w480) -> (single precision float=w479:sgl[])
                n156 = call "IMAQ GetPixelLine"("Line Coordinates"=w475, "Image"=w473) -> ("Pixels Line (Float)"=w476:sgl[])  [unwired: 2 in, 4 out]
                n157 = Divide(x=w479, y=w474) -> (x/y=w478:sgl[])
                n158 = Add(x=w476, y=w478) -> (x+y=w477:sgl[])
              }
            }
            n159 = call "IMAQ SetPixelLine"("Pixels Line (Float)"=w453, "Line Coordinates"=w454, "Image"=w437) -> ()  [unwired: 7 in, 2 out]
            n160 = And(x=w442, y=w434) -> (x .and. y?=w443:bool)
            n161 = case shown="False" w443 {
              tunnel: w453 -> [_ w467]
              tunnel: w452 -> [_ w465]
              tunnel: w436 -> [_ w464]
              frame False {
              }
              frame True {
                n162 = Write to Binary File(file (use dialog)=w464, data=w467, 5:FALSE ("prepend array or string size? (T)"), 9:w465) -> ()  [unwired: 2 in, 3 out]
              }
            }
          }
        }
      }
      n163 = case shown="True" w390 {
        frame False {
        }
        frame True {
          w409 = u16 1 items=["Read", "Write"] ("Mode")
          n164 = call "File Action V1.vi"("Action"="Close Files", "Mode"=w409) -> ()  [unwired: 11 in, 3 out]
        }
      }
    }
    frame 2, 18 {
      n165 = while {
        shift-right: [w516] -> _
        shift-left: 0 -> [w517]
        tunnel: w495 -> [w518]
        tunnel: w494 -> [w515]
        tunnel: w493 -> [w514]
        tunnel: w492 -> [w513]
        tunnel: w491 -> [w509]
        shift-right: [w506] -> _
        shift-left: u32 0 -> [w507]
        tunnel: w489 -> [w505]
        tunnel: w488 -> [w504]
        tunnel: w487 -> [w503]
        tunnel: w486 -> [w502]
        tunnel: w481 -> [w501]
        tunnel: w485 -> [w500]
        tunnel: w484 -> [w499]
        tunnel: w483 -> [w498]
        tunnel: w482 -> [w497]
        stop <- w508 stop-if-true
        n166 = Get Queue Status(queue=w502) -> (queue out=w510:refnum<queue>, # elements in queue=w512:i32)  [unwired: 2 in, 6 out]
        n167 = Get Notifier Status(notifier=w509) -> (current notification=w508:bool)  [unwired: 1 in, 4 out]
        n168 = Greater Than 0?(x=w512) -> (x > 0?=w511:bool)
        n169 = case shown="False" w511 {
          tunnel: w518 -> [_ w543]
          tunnel: w517 -> [w520 w544]
          tunnel: [w520 w542] -> w516
          tunnel: w515 -> [_ w539]
          tunnel: w514 -> [_ w538]
          tunnel: w513 -> [_ w528]
          tunnel: w510 -> [_ w537]
          tunnel: w507 -> [w519 w534]
          tunnel: [w519 w533] -> w506
          tunnel: w505 -> [_ w532]
          tunnel: w504 -> [_ w531]
          tunnel: w503 -> [_ w526]
          tunnel: w501 -> [_ w524]
          tunnel: w500 -> [_ w522]
          tunnel: w499 -> [_ _]
          tunnel: w498 -> [_ _]
          tunnel: w497 -> [_ _]
          frame False {
          }
          frame True {
            # "False: 1st frame in fram accum"
            # "True: Last Frame of frame accum"
            # "Current Line in Frame Accum"
            # "Current Line In Frame"
            n170 = Increment(x=w534) -> (x+1=w527:u32)
            n171 = Dequeue Element(queue=w537) -> (element=w549:u64[])  [unwired: 2 in, 3 out]
            n172 = Equal?(x=w527, y=w531) -> (x = y?=w536:bool)
            n173 = Greater?(x=w527, y=w532) -> (0:w529:bool)
            n174 = Greater?(x=w527, y=w526) -> (0:w525:bool)
            n175 = Split Number(x=w549) -> (hi(x)=w550:u32[])  [unwired: 1 out]
            n176 = Split Number(x=w550) -> (lo(x)=w521:u16[])  [unwired: 1 out]
            n177 = Select(t=u32 0, s=w536, f=w527) -> (s? t:f=w533:u32)
            n178 = Increment(x=w544) -> (x+1=w546:i32)
            n179 = Equal?(x=w543, y=w544) -> (x = y?=w545:bool)
            n180 = Select(t=0, s=w545, f=w546) -> (s? t:f=w542:i32)
            n181 = Build Array(0, w544, w543, w544) -> (w541:i32[])
            n182 = case shown="True" w525 {
              tunnel: w521 -> [w558 w567]
              tunnel: [w557 w564] -> w540
              tunnel: w541 -> [_ w562]
              tunnel: w538 -> [w556 w561]
              tunnel: w524 -> [w555 w560]
              tunnel: [w555 w560] -> w523
              frame False {
                n183 = To Single Precision Float(number=w558) -> (single precision float=w559:sgl[])
                n184 = Divide(x=w559, y=w556) -> (x/y=w557:sgl[])
              }
              frame True {
                n185 = To Single Precision Float(number=w567) -> (single precision float=w566:sgl[])
                n186 = call "IMAQ GetPixelLine"("Line Coordinates"=w562, "Image"=w560) -> ("Pixels Line (Float)"=w563:sgl[])  [unwired: 2 in, 4 out]
                n187 = Divide(x=w566, y=w561) -> (x/y=w565:sgl[])
                n188 = Add(x=w563, y=w565) -> (x+y=w564:sgl[])
              }
            }
            n189 = call "IMAQ SetPixelLine"("Pixels Line (Float)"=w540, "Line Coordinates"=w541, "Image"=w523) -> ()  [unwired: 7 in, 2 out]
            n190 = And(x=w529, y=w528) -> (x .and. y?=w530:bool)
            n191 = case shown="True" w530 {
              tunnel: w540 -> [_ w554]
              tunnel: w539 -> [_ w552]
              tunnel: w522 -> [_ w551]
              frame False {
              }
              frame True {
                n192 = Write to Binary File(file (use dialog)=w551, data=w554, 5:FALSE ("prepend array or string size? (T)"), 9:w552) -> ()  [unwired: 2 in, 3 out]
              }
            }
          }
        }
      }
    }
    frame 3 {
      n193 = while {
        shift-right: [w606] -> _
        shift-left: 0 -> [w607]
        tunnel: w584 -> [w608]
        tunnel: w583 -> [w605]
        tunnel: w582 -> [w604]
        tunnel: w581 -> [w603]
        tunnel: w580 -> [w600]
        shift-right: [w597] -> _
        shift-left: u32 0 -> [w598]
        tunnel: w578 -> [w596]
        tunnel: w577 -> [w595]
        tunnel: w576 -> [w594]
        tunnel: w569 -> [w593]
        tunnel: w571 -> [w592]
        tunnel: w570 -> [w591]
        tunnel: w575 -> [w590]
        tunnel: w574 -> [w589]
        tunnel: w573 -> [w588]
        tunnel: w572 -> [w587]
        tunnel: [w586] -> w568
        stop <- w599 stop-if-true
        n194 = Get Queue Status(queue=w593) -> (queue out=w586:refnum<queue>, # elements in queue=w602:i32)  [unwired: 2 in, 6 out]
        n195 = Get Notifier Status(notifier=w600) -> (current notification=w599:bool)  [unwired: 1 in, 4 out]
        n196 = Greater Than 0?(x=w602) -> (x > 0?=w601:bool)
        n197 = case shown="True" w601 {
          tunnel: w608 -> [_ w638]
          tunnel: w607 -> [w610 w639]
          tunnel: [w610 w637] -> w606
          tunnel: w605 -> [_ w633]
          tunnel: w604 -> [_ w632]
          tunnel: w603 -> [_ w622]
          tunnel: w586 -> [_ w631]
          tunnel: w598 -> [w609 w628]
          tunnel: [w609 w627] -> w597
          tunnel: w596 -> [_ w626]
          tunnel: w595 -> [_ w625]
          tunnel: w594 -> [_ w620]
          tunnel: w592 -> [_ w618]
          tunnel: w591 -> [_ w617]
          tunnel: w590 -> [_ w614]
          tunnel: w589 -> [_ w613]
          tunnel: w588 -> [_ _]
          tunnel: w587 -> [_ _]
          frame False {
          }
          frame True {
            # "False: 1st frame in fram accum"
            # "True: Last Frame of frame accum"
            # "Current Line in Frame Accum"
            # "Current Line In Frame"
            n198 = Increment(x=w628) -> (x+1=w621:u32)
            n199 = Dequeue Element(queue=w631) -> (element=w644:u64[])  [unwired: 2 in, 3 out]
            n200 = Equal?(x=w621, y=w625) -> (x = y?=w630:bool)
            n201 = Greater?(x=w621, y=w626) -> (0:w623:bool)
            n202 = Greater?(x=w621, y=w620) -> (0:w619:bool)
            n203 = Split Number(x=w644) -> (hi(x)=w645:u32[])  [unwired: 1 out]
            n204 = Split Number(x=w645) -> (hi(x)=w612:u16[], lo(x)=w611:u16[])
            n205 = Select(t=u32 0, s=w630, f=w621) -> (s? t:f=w627:u32)
            n206 = Increment(x=w639) -> (x+1=w641:i32)
            n207 = Equal?(x=w638, y=w639) -> (x = y?=w640:bool)
            n208 = Select(t=0, s=w640, f=w641) -> (s? t:f=w637:i32)
            n209 = Build Array(0, w639, w638, w639) -> (w636:i32[])
            n210 = case shown="True" w619 {
              tunnel: w612 -> [w658 w674]
              tunnel: w611 -> [w657 w673]
              tunnel: [w655 w668] -> w634
              tunnel: [w656 w667] -> w635
              tunnel: w636 -> [_ w664]
              tunnel: w632 -> [w654 w663]
              tunnel: w618 -> [w653 w661]
              tunnel: w617 -> [w652 w662]
              tunnel: [w652 w662] -> w615
              tunnel: [w653 w661] -> w616
              frame False {
                n211 = To Single Precision Float(number=w658) -> (single precision float=w660:sgl[])
                n212 = To Single Precision Float(number=w657) -> (single precision float=w659:sgl[])
                n213 = Divide(x=w660, y=w654) -> (x/y=w656:sgl[])
                n214 = Divide(x=w659, y=w654) -> (x/y=w655:sgl[])
              }
              frame True {
                n215 = To Single Precision Float(number=w674) -> (single precision float=w672:sgl[])
                n216 = To Single Precision Float(number=w673) -> (single precision float=w671:sgl[])
                n217 = call "IMAQ GetPixelLine"("Line Coordinates"=w664, "Image"=w661) -> ("Pixels Line (Float)"=w666:sgl[])  [unwired: 2 in, 4 out]
                n218 = call "IMAQ GetPixelLine"("Line Coordinates"=w664, "Image"=w662) -> ("Pixels Line (Float)"=w665:sgl[])  [unwired: 2 in, 4 out]
                n219 = Divide(x=w672, y=w663) -> (x/y=w670:sgl[])
                n220 = Divide(x=w671, y=w663) -> (x/y=w669:sgl[])
                n221 = Add(x=w666, y=w670) -> (x+y=w667:sgl[])
                n222 = Add(x=w665, y=w669) -> (x+y=w668:sgl[])
              }
            }
            n223 = call "IMAQ SetPixelLine"("Pixels Line (Float)"=w635, "Line Coordinates"=w636, "Image"=w616) -> ()  [unwired: 7 in, 2 out]
            n224 = call "IMAQ SetPixelLine"("Pixels Line (Float)"=w634, "Line Coordinates"=w636, "Image"=w615) -> ()  [unwired: 7 in, 2 out]
            n225 = And(x=w623, y=w622) -> (x .and. y?=w624:bool)
            n226 = case shown="False" w624 {
              tunnel: w635 -> [_ w651]
              tunnel: w634 -> [_ w650]
              tunnel: w633 -> [_ w648]
              tunnel: w614 -> [_ w647]
              tunnel: w613 -> [_ w646]
              frame False {
              }
              frame True {
                w649 = FALSE ("prepend array or string size? (T)")
                n227 = Write to Binary File(file (use dialog)=w647, data=w651, 5:w649, 9:w648) -> ()  [unwired: 2 in, 3 out]
                n228 = Write to Binary File(file (use dialog)=w646, data=w650, 5:w649, 9:w648) -> ()  [unwired: 2 in, 3 out]
              }
            }
          }
        }
      }
    }
    frame 4, 20 {
      n229 = while {
        shift-right: [w710] -> _
        shift-left: 0 -> [w711]
        tunnel: w689 -> [w712]
        tunnel: w688 -> [w709]
        tunnel: w687 -> [w708]
        tunnel: w686 -> [w707]
        tunnel: w685 -> [w703]
        shift-right: [w700] -> _
        shift-left: u32 0 -> [w701]
        tunnel: w683 -> [w699]
        tunnel: w682 -> [w698]
        tunnel: w681 -> [w697]
        tunnel: w680 -> [w696]
        tunnel: w675 -> [w695]
        tunnel: w679 -> [w694]
        tunnel: w678 -> [w693]
        tunnel: w677 -> [w692]
        tunnel: w676 -> [w691]
        stop <- w702 stop-if-true
        n230 = Get Queue Status(queue=w696) -> (queue out=w704:refnum<queue>, # elements in queue=w706:i32)  [unwired: 2 in, 6 out]
        n231 = Get Notifier Status(notifier=w703) -> (current notification=w702:bool)  [unwired: 1 in, 4 out]
        n232 = Greater Than 0?(x=w706) -> (x > 0?=w705:bool)
        n233 = case shown="True" w705 {
          tunnel: w712 -> [_ w737]
          tunnel: w711 -> [w714 w738]
          tunnel: [w714 w736] -> w710
          tunnel: w709 -> [_ w733]
          tunnel: w708 -> [_ w732]
          tunnel: w707 -> [_ w722]
          tunnel: w704 -> [_ w731]
          tunnel: w701 -> [w713 w728]
          tunnel: [w713 w727] -> w700
          tunnel: w699 -> [_ w726]
          tunnel: w698 -> [_ w725]
          tunnel: w697 -> [_ w720]
          tunnel: w695 -> [_ w718]
          tunnel: w694 -> [_ w716]
          tunnel: w693 -> [_ _]
          tunnel: w692 -> [_ _]
          tunnel: w691 -> [_ _]
          frame False {
          }
          frame True {
            # "False: 1st frame in fram accum"
            # "True: Last Frame of frame accum"
            # "Current Line in Frame Accum"
            # "Current Line In Frame"
            n234 = Increment(x=w728) -> (x+1=w721:u32)
            n235 = Dequeue Element(queue=w731) -> (element=w744:u64[])  [unwired: 2 in, 3 out]
            n236 = Equal?(x=w721, y=w725) -> (x = y?=w730:bool)
            n237 = Greater?(x=w721, y=w726) -> (0:w723:bool)
            n238 = Greater?(x=w721, y=w720) -> (0:w719:bool)
            n239 = Split Number(x=w744) -> (lo(x)=w743:u32[])  [unwired: 1 out]
            n240 = Split Number(x=w743) -> (hi(x)=w715:u16[])  [unwired: 1 out]
            n241 = Select(t=u32 0, s=w730, f=w721) -> (s? t:f=w727:u32)
            n242 = Increment(x=w738) -> (x+1=w740:i32)
            n243 = Equal?(x=w737, y=w738) -> (x = y?=w739:bool)
            n244 = Select(t=0, s=w739, f=w740) -> (s? t:f=w736:i32)
            n245 = Build Array(0, w738, w737, w738) -> (w735:i32[])
            n246 = case shown="True" w719 {
              tunnel: w715 -> [w752 w761]
              tunnel: [w751 w758] -> w734
              tunnel: w735 -> [_ w756]
              tunnel: w732 -> [w750 w755]
              tunnel: w718 -> [w749 w754]
              tunnel: [w749 w754] -> w717
              frame False {
                n247 = To Single Precision Float(number=w752) -> (single precision float=w753:sgl[])
                n248 = Divide(x=w753, y=w750) -> (x/y=w751:sgl[])
              }
              frame True {
                n249 = To Single Precision Float(number=w761) -> (single precision float=w760:sgl[])
                n250 = call "IMAQ GetPixelLine"("Line Coordinates"=w756, "Image"=w754) -> ("Pixels Line (Float)"=w757:sgl[])  [unwired: 2 in, 4 out]
                n251 = Divide(x=w760, y=w755) -> (x/y=w759:sgl[])
                n252 = Add(x=w757, y=w759) -> (x+y=w758:sgl[])
              }
            }
            n253 = call "IMAQ SetPixelLine"("Pixels Line (Float)"=w734, "Line Coordinates"=w735, "Image"=w717) -> ()  [unwired: 7 in, 2 out]
            n254 = And(x=w723, y=w722) -> (x .and. y?=w724:bool)
            n255 = case shown="True" w724 {
              tunnel: w734 -> [_ w748]
              tunnel: w733 -> [_ w746]
              tunnel: w716 -> [_ w745]
              frame False {
              }
              frame True {
                n256 = Write to Binary File(file (use dialog)=w745, data=w748, 5:FALSE ("prepend array or string size? (T)"), 9:w746) -> ()  [unwired: 2 in, 3 out]
              }
            }
          }
        }
      }
    }
    frame 5 {
      n257 = while {
        shift-right: [w799] -> _
        shift-left: 0 -> [w800]
        tunnel: w777 -> [w801]
        tunnel: w776 -> [w798]
        tunnel: w775 -> [w797]
        tunnel: w774 -> [w796]
        tunnel: w773 -> [w792]
        shift-right: [w789] -> _
        shift-left: u32 0 -> [w790]
        tunnel: w771 -> [w788]
        tunnel: w770 -> [w787]
        tunnel: w769 -> [w786]
        tunnel: w768 -> [w785]
        tunnel: w763 -> [w784]
        tunnel: w762 -> [w783]
        tunnel: w767 -> [w782]
        tunnel: w766 -> [w781]
        tunnel: w765 -> [w780]
        tunnel: w764 -> [w779]
        stop <- w791 stop-if-true
        n258 = Get Queue Status(queue=w785) -> (queue out=w793:refnum<queue>, # elements in queue=w795:i32)  [unwired: 2 in, 6 out]
        n259 = Get Notifier Status(notifier=w792) -> (current notification=w791:bool)  [unwired: 1 in, 4 out]
        n260 = Greater Than 0?(x=w795) -> (x > 0?=w794:bool)
        n261 = case shown="True" w794 {
          tunnel: w801 -> [_ w830]
          tunnel: w800 -> [w803 w831]
          tunnel: [w803 w829] -> w799
          tunnel: w798 -> [_ w825]
          tunnel: w797 -> [_ w824]
          tunnel: w796 -> [_ w814]
          tunnel: w793 -> [_ w823]
          tunnel: w790 -> [w802 w820]
          tunnel: [w802 w819] -> w789
          tunnel: w788 -> [_ w818]
          tunnel: w787 -> [_ w817]
          tunnel: w786 -> [_ w812]
          tunnel: w784 -> [_ w810]
          tunnel: w783 -> [_ w809]
          tunnel: w782 -> [_ w805]
          tunnel: w781 -> [_ w804]
          tunnel: w780 -> [_ _]
          tunnel: w779 -> [_ _]
          frame False {
          }
          frame True {
            # "False: 1st frame in fram accum"
            # "True: Last Frame of frame accum"
            # "Current Line in Frame Accum"
            # "Current Line In Frame"
            n262 = Increment(x=w820) -> (x+1=w813:u32)
            n263 = Dequeue Element(queue=w823) -> (element=w838:u64[])  [unwired: 2 in, 3 out]
            n264 = Equal?(x=w813, y=w817) -> (x = y?=w822:bool)
            n265 = Greater?(x=w813, y=w818) -> (0:w815:bool)
            n266 = Greater?(x=w813, y=w812) -> (0:w811:bool)
            n267 = Split Number(x=w838) -> (hi(x)=w839:u32[], lo(x)=w837:u32[])
            n268 = Split Number(x=w839) -> (hi(x)=w806:u16[])  [unwired: 1 out]
            n269 = Split Number(x=w837) -> (hi(x)=w836:u16[])  [unwired: 1 out]
            n270 = Select(t=u32 0, s=w822, f=w813) -> (s? t:f=w819:u32)
            n271 = Increment(x=w831) -> (x+1=w833:i32)
            n272 = Equal?(x=w830, y=w831) -> (x = y?=w832:bool)
            n273 = Select(t=0, s=w832, f=w833) -> (s? t:f=w829:i32)
            n274 = Build Array(0, w831, w830, w831) -> (w828:i32[])
            n275 = case shown="False" w811 {
              tunnel: w806 -> [w853 w868]
              tunnel: w836 -> [w850 w867]
              tunnel: [w849 w863] -> w826
              tunnel: [w852 w862] -> w827
              tunnel: w828 -> [_ w859]
              tunnel: w824 -> [w848 w857]
              tunnel: w810 -> [w847 w855]
              tunnel: w809 -> [w846 w856]
              tunnel: [w846 w856] -> w807
              tunnel: [w847 w855] -> w808
              frame False {
                n276 = To Single Precision Float(number=w853) -> (single precision float=w854:sgl[])
                n277 = To Single Precision Float(number=w850) -> (single precision float=w851:sgl[])
                n278 = Divide(x=w854, y=w848) -> (x/y=w852:sgl[])
                n279 = Divide(x=w851, y=w848) -> (x/y=w849:sgl[])
              }
              frame True {
                n280 = To Single Precision Float(number=w868) -> (single precision float=w858:sgl[])
                n281 = To Single Precision Float(number=w867) -> (single precision float=w866:sgl[])
                n282 = call "IMAQ GetPixelLine"("Line Coordinates"=w859, "Image"=w855) -> ("Pixels Line (Float)"=w861:sgl[])  [unwired: 2 in, 4 out]
                n283 = call "IMAQ GetPixelLine"("Line Coordinates"=w859, "Image"=w856) -> ("Pixels Line (Float)"=w860:sgl[])  [unwired: 2 in, 4 out]
                n284 = Divide(x=w858, y=w857) -> (x/y=w865:sgl[])
                n285 = Divide(x=w866, y=w857) -> (x/y=w864:sgl[])
                n286 = Add(x=w861, y=w865) -> (x+y=w862:sgl[])
                n287 = Add(x=w860, y=w864) -> (x+y=w863:sgl[])
              }
            }
            n288 = call "IMAQ SetPixelLine"("Pixels Line (Float)"=w827, "Line Coordinates"=w828, "Image"=w808) -> ()  [unwired: 7 in, 2 out]
            n289 = call "IMAQ SetPixelLine"("Pixels Line (Float)"=w826, "Line Coordinates"=w828, "Image"=w807) -> ()  [unwired: 7 in, 2 out]
            n290 = And(x=w815, y=w814) -> (x .and. y?=w816:bool)
            n291 = case shown="True" w816 {
              tunnel: w827 -> [_ w845]
              tunnel: w826 -> [_ w844]
              tunnel: w825 -> [_ w842]
              tunnel: w805 -> [_ w841]
              tunnel: w804 -> [_ w840]
              frame False {
              }
              frame True {
                w843 = FALSE ("prepend array or string size? (T)")
                n292 = Write to Binary File(file (use dialog)=w841, data=w845, 5:w843, 9:w842) -> ()  [unwired: 2 in, 3 out]
                n293 = Write to Binary File(file (use dialog)=w840, data=w844, 5:w843, 9:w842) -> ()  [unwired: 2 in, 3 out]
              }
            }
          }
        }
      }
    }
    frame 6 {
      n294 = while {
        shift-right: [w906] -> _
        shift-left: 0 -> [w907]
        tunnel: w884 -> [w908]
        tunnel: w883 -> [w905]
        tunnel: w882 -> [w904]
        tunnel: w881 -> [w903]
        tunnel: w880 -> [w899]
        shift-right: [w896] -> _
        shift-left: u32 0 -> [w897]
        tunnel: w878 -> [w895]
        tunnel: w877 -> [w894]
        tunnel: w876 -> [w893]
        tunnel: w875 -> [w892]
        tunnel: w870 -> [w891]
        tunnel: w869 -> [w890]
        tunnel: w874 -> [w889]
        tunnel: w873 -> [w888]
        tunnel: w872 -> [w887]
        tunnel: w871 -> [w886]
        stop <- w898 stop-if-true
        n295 = Get Queue Status(queue=w892) -> (queue out=w900:refnum<queue>, # elements in queue=w902:i32)  [unwired: 2 in, 6 out]
        n296 = Get Notifier Status(notifier=w899) -> (current notification=w898:bool)  [unwired: 1 in, 4 out]
        n297 = Greater Than 0?(x=w902) -> (x > 0?=w901:bool)
        n298 = case shown="True" w901 {
          tunnel: w908 -> [_ w936]
          tunnel: w907 -> [w910 w937]
          tunnel: [w910 w935] -> w906
          tunnel: w905 -> [_ w931]
          tunnel: w904 -> [_ w930]
          tunnel: w903 -> [_ w920]
          tunnel: w900 -> [_ w929]
          tunnel: w897 -> [w909 w926]
          tunnel: [w909 w925] -> w896
          tunnel: w895 -> [_ w924]
          tunnel: w894 -> [_ w923]
          tunnel: w893 -> [_ w918]
          tunnel: w891 -> [_ w916]
          tunnel: w890 -> [_ w915]
          tunnel: w889 -> [_ w912]
          tunnel: w888 -> [_ w911]
          tunnel: w887 -> [_ _]
          tunnel: w886 -> [_ _]
          frame False {
          }
          frame True {
            # "False: 1st frame in fram accum"
            # "True: Last Frame of frame accum"
            # "Current Line in Frame Accum"
            # "Current Line In Frame"
            n299 = Increment(x=w926) -> (x+1=w919:u32)
            n300 = Dequeue Element(queue=w929) -> (element=w945:u64[])  [unwired: 2 in, 3 out]
            n301 = Equal?(x=w919, y=w923) -> (x = y?=w928:bool)
            n302 = Greater?(x=w919, y=w924) -> (0:w921:bool)
            n303 = Greater?(x=w919, y=w918) -> (0:w917:bool)
            n304 = Split Number(x=w945) -> (hi(x)=w946:u32[], lo(x)=w944:u32[])
            n305 = Split Number(x=w946) -> (lo(x)=w943:u16[])  [unwired: 1 out]
            n306 = Split Number(x=w944) -> (hi(x)=w942:u16[])  [unwired: 1 out]
            n307 = Select(t=u32 0, s=w928, f=w919) -> (s? t:f=w925:u32)
            n308 = Increment(x=w937) -> (x+1=w939:i32)
            n309 = Equal?(x=w936, y=w937) -> (x = y?=w938:bool)
            n310 = Select(t=0, s=w938, f=w939) -> (s? t:f=w935:i32)
            n311 = Build Array(0, w937, w936, w937) -> (w934:i32[])
            n312 = case shown="False" w917 {
              tunnel: w943 -> [w959 w975]
              tunnel: w942 -> [w958 w974]
              tunnel: [w956 w969] -> w932
              tunnel: [w957 w968] -> w933
              tunnel: w934 -> [_ w965]
              tunnel: w930 -> [w955 w964]
              tunnel: w916 -> [w954 w962]
              tunnel: w915 -> [w953 w963]
              tunnel: [w953 w963] -> w913
              tunnel: [w954 w962] -> w914
              frame False {
                n313 = To Single Precision Float(number=w959) -> (single precision float=w961:sgl[])
                n314 = To Single Precision Float(number=w958) -> (single precision float=w960:sgl[])
                n315 = Divide(x=w961, y=w955) -> (x/y=w957:sgl[])
                n316 = Divide(x=w960, y=w955) -> (x/y=w956:sgl[])
              }
              frame True {
                n317 = To Single Precision Float(number=w975) -> (single precision float=w973:sgl[])
                n318 = To Single Precision Float(number=w974) -> (single precision float=w972:sgl[])
                n319 = call "IMAQ GetPixelLine"("Line Coordinates"=w965, "Image"=w962) -> ("Pixels Line (Float)"=w967:sgl[])  [unwired: 2 in, 4 out]
                n320 = call "IMAQ GetPixelLine"("Line Coordinates"=w965, "Image"=w963) -> ("Pixels Line (Float)"=w966:sgl[])  [unwired: 2 in, 4 out]
                n321 = Divide(x=w973, y=w964) -> (x/y=w971:sgl[])
                n322 = Divide(x=w972, y=w964) -> (x/y=w970:sgl[])
                n323 = Add(x=w967, y=w971) -> (x+y=w968:sgl[])
                n324 = Add(x=w966, y=w970) -> (x+y=w969:sgl[])
              }
            }
            n325 = call "IMAQ SetPixelLine"("Pixels Line (Float)"=w933, "Line Coordinates"=w934, "Image"=w914) -> ()  [unwired: 7 in, 2 out]
            n326 = call "IMAQ SetPixelLine"("Pixels Line (Float)"=w932, "Line Coordinates"=w934, "Image"=w913) -> ()  [unwired: 7 in, 2 out]
            n327 = And(x=w921, y=w920) -> (x .and. y?=w922:bool)
            n328 = case shown="True" w922 {
              tunnel: w933 -> [_ w952]
              tunnel: w932 -> [_ w951]
              tunnel: w931 -> [_ w949]
              tunnel: w912 -> [_ w948]
              tunnel: w911 -> [_ w947]
              frame False {
              }
              frame True {
                w950 = FALSE ("prepend array or string size? (T)")
                n329 = Write to Binary File(file (use dialog)=w948, data=w952, 5:w950, 9:w949) -> ()  [unwired: 2 in, 3 out]
                n330 = Write to Binary File(file (use dialog)=w947, data=w951, 5:w950, 9:w949) -> ()  [unwired: 2 in, 3 out]
              }
            }
          }
        }
      }
    }
    frame 7 {
      n331 = while {
        shift-right: [w1015] -> _
        shift-left: 0 -> [w1016]
        tunnel: w992 -> [w1017]
        tunnel: w991 -> [w1014]
        tunnel: w990 -> [w1013]
        tunnel: w989 -> [w1012]
        tunnel: w988 -> [w1008]
        shift-right: [w1005] -> _
        shift-left: u32 0 -> [w1006]
        tunnel: w986 -> [w1004]
        tunnel: w985 -> [w1003]
        tunnel: w984 -> [w1002]
        tunnel: w983 -> [w1001]
        tunnel: w978 -> [w1000]
        tunnel: w977 -> [w999]
        tunnel: w976 -> [w998]
        tunnel: w982 -> [w997]
        tunnel: w981 -> [w996]
        tunnel: w980 -> [w995]
        tunnel: w979 -> [w994]
        stop <- w1007 stop-if-true
        n332 = Get Queue Status(queue=w1001) -> (queue out=w1009:refnum<queue>, # elements in queue=w1011:i32)  [unwired: 2 in, 6 out]
        n333 = Get Notifier Status(notifier=w1008) -> (current notification=w1007:bool)  [unwired: 1 in, 4 out]
        n334 = Greater Than 0?(x=w1011) -> (x > 0?=w1010:bool)
        n335 = case shown="True" w1010 {
          tunnel: w1017 -> [_ w1050]
          tunnel: w1016 -> [w1019 w1051]
          tunnel: [w1019 w1049] -> w1015
          tunnel: w1014 -> [_ w1044]
          tunnel: w1013 -> [_ w1043]
          tunnel: w1012 -> [_ w1033]
          tunnel: w1009 -> [_ w1042]
          tunnel: w1006 -> [w1018 w1039]
          tunnel: [w1018 w1038] -> w1005
          tunnel: w1004 -> [_ w1037]
          tunnel: w1003 -> [_ w1036]
          tunnel: w1002 -> [_ w1031]
          tunnel: w1000 -> [_ w1029]
          tunnel: w999 -> [_ w1028]
          tunnel: w998 -> [_ w1027]
          tunnel: w997 -> [_ w1022]
          tunnel: w996 -> [_ w1021]
          tunnel: w995 -> [_ w1020]
          tunnel: w994 -> [_ _]
          frame False {
          }
          frame True {
            # "False: 1st frame in fram accum"
            # "True: Last Frame of frame accum"
            # "Current Line in Frame Accum"
            # "Current Line In Frame"
            n336 = Increment(x=w1039) -> (x+1=w1032:u32)
            n337 = Dequeue Element(queue=w1042) -> (element=w1059:u64[])  [unwired: 2 in, 3 out]
            n338 = Equal?(x=w1032, y=w1036) -> (x = y?=w1041:bool)
            n339 = Greater?(x=w1032, y=w1037) -> (0:w1034:bool)
            n340 = Greater?(x=w1032, y=w1031) -> (0:w1030:bool)
            n341 = Split Number(x=w1059) -> (hi(x)=w1060:u32[], lo(x)=w1058:u32[])
            n342 = Split Number(x=w1060) -> (hi(x)=w1023:u16[], lo(x)=w1057:u16[])
            n343 = Split Number(x=w1058) -> (hi(x)=w1056:u16[])  [unwired: 1 out]
            n344 = Select(t=u32 0, s=w1041, f=w1032) -> (s? t:f=w1038:u32)
            n345 = Increment(x=w1051) -> (x+1=w1053:i32)
            n346 = Equal?(x=w1050, y=w1051) -> (x = y?=w1052:bool)
            n347 = Select(t=0, s=w1052, f=w1053) -> (s? t:f=w1049:i32)
            n348 = Build Array(0, w1051, w1050, w1051) -> (w1048:i32[])
            n349 = case shown="False" w1030 {
              tunnel: w1023 -> [w1080 w1101]
              tunnel: w1057 -> [w1076 w1100]
              tunnel: w1056 -> [w1075 w1099]
              tunnel: [w1073 w1093] -> w1045
              tunnel: [w1074 w1092] -> w1046
              tunnel: [w1079 w1091] -> w1047
              tunnel: w1048 -> [_ w1087]
              tunnel: w1043 -> [w1072 w1085]
              tunnel: w1029 -> [w1071 w1082]
              tunnel: w1028 -> [w1070 w1083]
              tunnel: w1027 -> [w1069 w1084]
              tunnel: [w1069 w1084] -> w1024
              tunnel: [w1070 w1083] -> w1025
              tunnel: [w1071 w1082] -> w1026
              frame False {
                n350 = To Single Precision Float(number=w1080) -> (single precision float=w1081:sgl[])
                n351 = To Single Precision Float(number=w1076) -> (single precision float=w1078:sgl[])
                n352 = To Single Precision Float(number=w1075) -> (single precision float=w1077:sgl[])
                n353 = Divide(x=w1081, y=w1072) -> (x/y=w1079:sgl[])
                n354 = Divide(x=w1078, y=w1072) -> (x/y=w1074:sgl[])
                n355 = Divide(x=w1077, y=w1072) -> (x/y=w1073:sgl[])
              }
              frame True {
                n356 = To Single Precision Float(number=w1101) -> (single precision float=w1086:sgl[])
                n357 = To Single Precision Float(number=w1100) -> (single precision float=w1098:sgl[])
                n358 = To Single Precision Float(number=w1099) -> (single precision float=w1097:sgl[])
                n359 = call "IMAQ GetPixelLine"("Line Coordinates"=w1087, "Image"=w1082) -> ("Pixels Line (Float)"=w1090:sgl[])  [unwired: 2 in, 4 out]
                n360 = call "IMAQ GetPixelLine"("Line Coordinates"=w1087, "Image"=w1083) -> ("Pixels Line (Float)"=w1089:sgl[])  [unwired: 2 in, 4 out]
                n361 = call "IMAQ GetPixelLine"("Line Coordinates"=w1087, "Image"=w1084) -> ("Pixels Line (Float)"=w1088:sgl[])  [unwired: 2 in, 4 out]
                n362 = Divide(x=w1086, y=w1085) -> (x/y=w1096:sgl[])
                n363 = Divide(x=w1098, y=w1085) -> (x/y=w1095:sgl[])
                n364 = Divide(x=w1097, y=w1085) -> (x/y=w1094:sgl[])
                n365 = Add(x=w1090, y=w1096) -> (x+y=w1091:sgl[])
                n366 = Add(x=w1089, y=w1095) -> (x+y=w1092:sgl[])
                n367 = Add(x=w1088, y=w1094) -> (x+y=w1093:sgl[])
              }
            }
            n368 = call "IMAQ SetPixelLine"("Pixels Line (Float)"=w1047, "Line Coordinates"=w1048, "Image"=w1026) -> ()  [unwired: 7 in, 2 out]
            n369 = call "IMAQ SetPixelLine"("Pixels Line (Float)"=w1046, "Line Coordinates"=w1048, "Image"=w1025) -> ()  [unwired: 7 in, 2 out]
            n370 = call "IMAQ SetPixelLine"("Pixels Line (Float)"=w1045, "Line Coordinates"=w1048, "Image"=w1024) -> ()  [unwired: 7 in, 2 out]
            n371 = And(x=w1034, y=w1033) -> (x .and. y?=w1035:bool)
            n372 = case shown="True" w1035 {
              tunnel: w1047 -> [_ w1068]
              tunnel: w1046 -> [_ w1067]
              tunnel: w1045 -> [_ w1066]
              tunnel: w1044 -> [_ w1064]
              tunnel: w1022 -> [_ w1063]
              tunnel: w1021 -> [_ w1062]
              tunnel: w1020 -> [_ w1061]
              frame False {
              }
              frame True {
                w1065 = FALSE ("prepend array or string size? (T)")
                n373 = Write to Binary File(file (use dialog)=w1063, data=w1068, 5:w1065, 9:w1064) -> ()  [unwired: 2 in, 3 out]
                n374 = Write to Binary File(file (use dialog)=w1062, data=w1067, 5:w1065, 9:w1064) -> ()  [unwired: 2 in, 3 out]
                n375 = Write to Binary File(file (use dialog)=w1061, data=w1066, 5:w1065, 9:w1064) -> ()  [unwired: 2 in, 3 out]
              }
            }
          }
        }
      }
    }
    frame 8, 24 {
      n376 = while {
        shift-right: [w1137] -> _
        shift-left: 0 -> [w1138]
        tunnel: w1116 -> [w1139]
        tunnel: w1115 -> [w1136]
        tunnel: w1114 -> [w1135]
        tunnel: w1113 -> [w1134]
        tunnel: w1112 -> [w1130]
        shift-right: [w1127] -> _
        shift-left: u32 0 -> [w1128]
        tunnel: w1110 -> [w1126]
        tunnel: w1109 -> [w1125]
        tunnel: w1108 -> [w1124]
        tunnel: w1107 -> [w1123]
        tunnel: w1102 -> [w1122]
        tunnel: w1106 -> [w1121]
        tunnel: w1105 -> [w1120]
        tunnel: w1104 -> [w1119]
        tunnel: w1103 -> [w1118]
        stop <- w1129 stop-if-true
        n377 = Get Queue Status(queue=w1123) -> (queue out=w1131:refnum<queue>, # elements in queue=w1133:i32)  [unwired: 2 in, 6 out]
        n378 = Get Notifier Status(notifier=w1130) -> (current notification=w1129:bool)  [unwired: 1 in, 4 out]
        n379 = Greater Than 0?(x=w1133) -> (x > 0?=w1132:bool)
        n380 = case shown="True" w1132 {
          tunnel: w1139 -> [_ w1163]
          tunnel: w1138 -> [w1141 w1164]
          tunnel: [w1141 w1162] -> w1137
          tunnel: w1136 -> [_ w1159]
          tunnel: w1135 -> [_ w1158]
          tunnel: w1134 -> [_ w1148]
          tunnel: w1131 -> [_ w1157]
          tunnel: w1128 -> [w1140 w1154]
          tunnel: [w1140 w1153] -> w1127
          tunnel: w1126 -> [_ w1152]
          tunnel: w1125 -> [_ w1151]
          tunnel: w1124 -> [_ w1146]
          tunnel: w1122 -> [_ w1144]
          tunnel: w1121 -> [_ w1142]
          tunnel: w1120 -> [_ _]
          tunnel: w1119 -> [_ _]
          tunnel: w1118 -> [_ _]
          frame False {
          }
          frame True {
            # "False: 1st frame in fram accum"
            # "True: Last Frame of frame accum"
            # "Current Line in Frame Accum"
            # "Current Line In Frame"
            n381 = Increment(x=w1154) -> (x+1=w1147:u32)
            n382 = Dequeue Element(queue=w1157) -> (element=w1171:u64[])  [unwired: 2 in, 3 out]
            n383 = Equal?(x=w1147, y=w1151) -> (x = y?=w1156:bool)
            n384 = Greater?(x=w1147, y=w1152) -> (0:w1149:bool)
            n385 = Greater?(x=w1147, y=w1146) -> (0:w1145:bool)
            n386 = Split Number(x=w1171) -> (lo(x)=w1170:u32[])  [unwired: 1 out]
            n387 = Split Number(x=w1170) -> (lo(x)=w1169:u16[])  [unwired: 1 out]
            n388 = Select(t=u32 0, s=w1156, f=w1147) -> (s? t:f=w1153:u32)
            n389 = Increment(x=w1164) -> (x+1=w1166:i32)
            n390 = Equal?(x=w1163, y=w1164) -> (x = y?=w1165:bool)
            n391 = Select(t=0, s=w1165, f=w1166) -> (s? t:f=w1162:i32)
            n392 = Build Array(0, w1164, w1163, w1164) -> (w1161:i32[])
            n393 = case shown="True" w1145 {
              tunnel: w1169 -> [w1179 w1188]
              tunnel: [w1178 w1185] -> w1160
              tunnel: w1161 -> [_ w1183]
              tunnel: w1158 -> [w1177 w1182]
              tunnel: w1144 -> [w1176 w1181]
              tunnel: [w1176 w1181] -> w1143
              frame False {
                n394 = To Single Precision Float(number=w1179) -> (single precision float=w1180:sgl[])
                n395 = Divide(x=w1180, y=w1177) -> (x/y=w1178:sgl[])
              }
              frame True {
                n396 = To Single Precision Float(number=w1188) -> (single precision float=w1187:sgl[])
                n397 = call "IMAQ GetPixelLine"("Line Coordinates"=w1183, "Image"=w1181) -> ("Pixels Line (Float)"=w1184:sgl[])  [unwired: 2 in, 4 out]
                n398 = Divide(x=w1187, y=w1182) -> (x/y=w1186:sgl[])
                n399 = Add(x=w1184, y=w1186) -> (x+y=w1185:sgl[])
              }
            }
            n400 = call "IMAQ SetPixelLine"("Pixels Line (Float)"=w1160, "Line Coordinates"=w1161, "Image"=w1143) -> ()  [unwired: 7 in, 2 out]
            n401 = And(x=w1149, y=w1148) -> (x .and. y?=w1150:bool)
            n402 = case shown="True" w1150 {
              tunnel: w1160 -> [_ w1175]
              tunnel: w1159 -> [_ w1173]
              tunnel: w1142 -> [_ w1172]
              frame False {
              }
              frame True {
                n403 = Write to Binary File(file (use dialog)=w1172, data=w1175, 5:FALSE ("prepend array or string size? (T)"), 9:w1173) -> ()  [unwired: 2 in, 3 out]
              }
            }
          }
        }
      }
    }
    frame 9 {
      n404 = while {
        shift-right: [w1226] -> _
        shift-left: 0 -> [w1227]
        tunnel: w1204 -> [w1228]
        tunnel: w1203 -> [w1225]
        tunnel: w1202 -> [w1224]
        tunnel: w1201 -> [w1223]
        tunnel: w1200 -> [w1219]
        shift-right: [w1216] -> _
        shift-left: u32 0 -> [w1217]
        tunnel: w1198 -> [w1215]
        tunnel: w1197 -> [w1214]
        tunnel: w1196 -> [w1213]
        tunnel: w1195 -> [w1212]
        tunnel: w1190 -> [w1211]
        tunnel: w1189 -> [w1210]
        tunnel: w1194 -> [w1209]
        tunnel: w1193 -> [w1208]
        tunnel: w1192 -> [w1207]
        tunnel: w1191 -> [w1206]
        stop <- w1218 stop-if-true
        n405 = Get Queue Status(queue=w1212) -> (queue out=w1220:refnum<queue>, # elements in queue=w1222:i32)  [unwired: 2 in, 6 out]
        n406 = Get Notifier Status(notifier=w1219) -> (current notification=w1218:bool)  [unwired: 1 in, 4 out]
        n407 = Greater Than 0?(x=w1222) -> (x > 0?=w1221:bool)
        n408 = case shown="True" w1221 {
          tunnel: w1228 -> [_ w1257]
          tunnel: w1227 -> [w1230 w1258]
          tunnel: [w1230 w1256] -> w1226
          tunnel: w1225 -> [_ w1252]
          tunnel: w1224 -> [_ w1251]
          tunnel: w1223 -> [_ w1241]
          tunnel: w1220 -> [_ w1250]
          tunnel: w1217 -> [w1229 w1247]
          tunnel: [w1229 w1246] -> w1216
          tunnel: w1215 -> [_ w1245]
          tunnel: w1214 -> [_ w1244]
          tunnel: w1213 -> [_ w1239]
          tunnel: w1211 -> [_ w1237]
          tunnel: w1210 -> [_ w1236]
          tunnel: w1209 -> [_ w1232]
          tunnel: w1208 -> [_ w1231]
          tunnel: w1207 -> [_ _]
          tunnel: w1206 -> [_ _]
          frame False {
          }
          frame True {
            # "False: 1st frame in fram accum"
            # "True: Last Frame of frame accum"
            # "Current Line in Frame Accum"
            # "Current Line In Frame"
            n409 = Increment(x=w1247) -> (x+1=w1240:u32)
            n410 = Dequeue Element(queue=w1250) -> (element=w1265:u64[])  [unwired: 2 in, 3 out]
            n411 = Equal?(x=w1240, y=w1244) -> (x = y?=w1249:bool)
            n412 = Greater?(x=w1240, y=w1245) -> (0:w1242:bool)
            n413 = Greater?(x=w1240, y=w1239) -> (0:w1238:bool)
            n414 = Split Number(x=w1265) -> (hi(x)=w1266:u32[], lo(x)=w1264:u32[])
            n415 = Split Number(x=w1266) -> (hi(x)=w1233:u16[])  [unwired: 1 out]
            n416 = Split Number(x=w1264) -> (lo(x)=w1263:u16[])  [unwired: 1 out]
            n417 = Select(t=u32 0, s=w1249, f=w1240) -> (s? t:f=w1246:u32)
            n418 = Increment(x=w1258) -> (x+1=w1260:i32)
            n419 = Equal?(x=w1257, y=w1258) -> (x = y?=w1259:bool)
            n420 = Select(t=0, s=w1259, f=w1260) -> (s? t:f=w1256:i32)
            n421 = Build Array(0, w1258, w1257, w1258) -> (w1255:i32[])
            n422 = case shown="True" w1238 {
              tunnel: w1233 -> [w1280 w1295]
              tunnel: w1263 -> [w1277 w1294]
              tunnel: [w1279 w1290] -> w1254
              tunnel: [w1276 w1289] -> w1253
              tunnel: w1255 -> [_ w1286]
              tunnel: w1251 -> [w1275 w1284]
              tunnel: w1237 -> [w1274 w1283]
              tunnel: w1236 -> [w1273 w1282]
              tunnel: [w1274 w1283] -> w1235
              tunnel: [w1273 w1282] -> w1234
              frame False {
                n423 = To Single Precision Float(number=w1280) -> (single precision float=w1281:sgl[])
                n424 = To Single Precision Float(number=w1277) -> (single precision float=w1278:sgl[])
                n425 = Divide(x=w1281, y=w1275) -> (x/y=w1279:sgl[])
                n426 = Divide(x=w1278, y=w1275) -> (x/y=w1276:sgl[])
              }
              frame True {
                n427 = To Single Precision Float(number=w1295) -> (single precision float=w1285:sgl[])
                n428 = To Single Precision Float(number=w1294) -> (single precision float=w1293:sgl[])
                n429 = call "IMAQ GetPixelLine"("Line Coordinates"=w1286, "Image"=w1283) -> ("Pixels Line (Float)"=w1288:sgl[])  [unwired: 2 in, 4 out]
                n430 = call "IMAQ GetPixelLine"("Line Coordinates"=w1286, "Image"=w1282) -> ("Pixels Line (Float)"=w1287:sgl[])  [unwired: 2 in, 4 out]
                n431 = Divide(x=w1285, y=w1284) -> (x/y=w1292:sgl[])
                n432 = Divide(x=w1293, y=w1284) -> (x/y=w1291:sgl[])
                n433 = Add(x=w1288, y=w1292) -> (x+y=w1290:sgl[])
                n434 = Add(x=w1287, y=w1291) -> (x+y=w1289:sgl[])
              }
            }
            n435 = call "IMAQ SetPixelLine"("Pixels Line (Float)"=w1254, "Line Coordinates"=w1255, "Image"=w1235) -> ()  [unwired: 7 in, 2 out]
            n436 = call "IMAQ SetPixelLine"("Pixels Line (Float)"=w1253, "Line Coordinates"=w1255, "Image"=w1234) -> ()  [unwired: 7 in, 2 out]
            n437 = And(x=w1242, y=w1241) -> (x .and. y?=w1243:bool)
            n438 = case shown="True" w1243 {
              tunnel: w1254 -> [_ w1272]
              tunnel: w1253 -> [_ w1271]
              tunnel: w1252 -> [_ w1269]
              tunnel: w1232 -> [_ w1268]
              tunnel: w1231 -> [_ w1267]
              frame False {
              }
              frame True {
                w1270 = FALSE ("prepend array or string size? (T)")
                n439 = Write to Binary File(file (use dialog)=w1268, data=w1272, 5:w1270, 9:w1269) -> ()  [unwired: 2 in, 3 out]
                n440 = Write to Binary File(file (use dialog)=w1267, data=w1271, 5:w1270, 9:w1269) -> ()  [unwired: 2 in, 3 out]
              }
            }
          }
        }
      }
    }
    frame 10 {
      n441 = while {
        shift-right: [w1333] -> _
        shift-left: 0 -> [w1334]
        tunnel: w1311 -> [w1335]
        tunnel: w1310 -> [w1332]
        tunnel: w1309 -> [w1331]
        tunnel: w1308 -> [w1330]
        tunnel: w1307 -> [w1326]
        shift-right: [w1323] -> _
        shift-left: u32 0 -> [w1324]
        tunnel: w1305 -> [w1322]
        tunnel: w1304 -> [w1321]
        tunnel: w1303 -> [w1320]
        tunnel: w1302 -> [w1319]
        tunnel: w1297 -> [w1318]
        tunnel: w1296 -> [w1317]
        tunnel: w1301 -> [w1316]
        tunnel: w1300 -> [w1315]
        tunnel: w1299 -> [w1314]
        tunnel: w1298 -> [w1313]
        stop <- w1325 stop-if-true
        n442 = Get Queue Status(queue=w1319) -> (queue out=w1327:refnum<queue>, # elements in queue=w1329:i32)  [unwired: 2 in, 6 out]
        n443 = Get Notifier Status(notifier=w1326) -> (current notification=w1325:bool)  [unwired: 1 in, 4 out]
        n444 = Greater Than 0?(x=w1329) -> (x > 0?=w1328:bool)
        n445 = case shown="True" w1328 {
          tunnel: w1335 -> [_ w1363]
          tunnel: w1334 -> [w1337 w1364]
          tunnel: [w1337 w1362] -> w1333
          tunnel: w1332 -> [_ w1358]
          tunnel: w1331 -> [_ w1357]
          tunnel: w1330 -> [_ w1347]
          tunnel: w1327 -> [_ w1356]
          tunnel: w1324 -> [w1336 w1353]
          tunnel: [w1336 w1352] -> w1323
          tunnel: w1322 -> [_ w1351]
          tunnel: w1321 -> [_ w1350]
          tunnel: w1320 -> [_ w1345]
          tunnel: w1318 -> [_ w1343]
          tunnel: w1317 -> [_ w1342]
          tunnel: w1316 -> [_ w1339]
          tunnel: w1315 -> [_ w1338]
          tunnel: w1314 -> [_ _]
          tunnel: w1313 -> [_ _]
          frame False {
          }
          frame True {
            # "False: 1st frame in fram accum"
            # "True: Last Frame of frame accum"
            # "Current Line in Frame Accum"
            # "Current Line In Frame"
            n446 = Increment(x=w1353) -> (x+1=w1346:u32)
            n447 = Dequeue Element(queue=w1356) -> (element=w1372:u64[])  [unwired: 2 in, 3 out]
            n448 = Equal?(x=w1346, y=w1350) -> (x = y?=w1355:bool)
            n449 = Greater?(x=w1346, y=w1351) -> (0:w1348:bool)
            n450 = Greater?(x=w1346, y=w1345) -> (0:w1344:bool)
            n451 = Split Number(x=w1372) -> (hi(x)=w1373:u32[], lo(x)=w1371:u32[])
            n452 = Split Number(x=w1373) -> (lo(x)=w1370:u16[])  [unwired: 1 out]
            n453 = Split Number(x=w1371) -> (lo(x)=w1369:u16[])  [unwired: 1 out]
            n454 = Select(t=u32 0, s=w1355, f=w1346) -> (s? t:f=w1352:u32)
            n455 = Increment(x=w1364) -> (x+1=w1366:i32)
            n456 = Equal?(x=w1363, y=w1364) -> (x = y?=w1365:bool)
            n457 = Select(t=0, s=w1365, f=w1366) -> (s? t:f=w1362:i32)
            n458 = Build Array(0, w1364, w1363, w1364) -> (w1361:i32[])
            n459 = case shown="True" w1344 {
              tunnel: w1370 -> [w1386 w1402]
              tunnel: w1369 -> [w1385 w1401]
              tunnel: [w1384 w1396] -> w1360
              tunnel: [w1383 w1395] -> w1359
              tunnel: w1361 -> [_ w1392]
              tunnel: w1357 -> [w1382 w1391]
              tunnel: w1343 -> [w1381 w1390]
              tunnel: w1342 -> [w1380 w1389]
              tunnel: [w1381 w1390] -> w1341
              tunnel: [w1380 w1389] -> w1340
              frame False {
                n460 = To Single Precision Float(number=w1386) -> (single precision float=w1388:sgl[])
                n461 = To Single Precision Float(number=w1385) -> (single precision float=w1387:sgl[])
                n462 = Divide(x=w1388, y=w1382) -> (x/y=w1384:sgl[])
                n463 = Divide(x=w1387, y=w1382) -> (x/y=w1383:sgl[])
              }
              frame True {
                n464 = To Single Precision Float(number=w1402) -> (single precision float=w1400:sgl[])
                n465 = To Single Precision Float(number=w1401) -> (single precision float=w1399:sgl[])
                n466 = call "IMAQ GetPixelLine"("Line Coordinates"=w1392, "Image"=w1390) -> ("Pixels Line (Float)"=w1394:sgl[])  [unwired: 2 in, 4 out]
                n467 = call "IMAQ GetPixelLine"("Line Coordinates"=w1392, "Image"=w1389) -> ("Pixels Line (Float)"=w1393:sgl[])  [unwired: 2 in, 4 out]
                n468 = Divide(x=w1400, y=w1391) -> (x/y=w1398:sgl[])
                n469 = Divide(x=w1399, y=w1391) -> (x/y=w1397:sgl[])
                n470 = Add(x=w1394, y=w1398) -> (x+y=w1396:sgl[])
                n471 = Add(x=w1393, y=w1397) -> (x+y=w1395:sgl[])
              }
            }
            n472 = call "IMAQ SetPixelLine"("Pixels Line (Float)"=w1360, "Line Coordinates"=w1361, "Image"=w1341) -> ()  [unwired: 7 in, 2 out]
            n473 = call "IMAQ SetPixelLine"("Pixels Line (Float)"=w1359, "Line Coordinates"=w1361, "Image"=w1340) -> ()  [unwired: 7 in, 2 out]
            n474 = And(x=w1348, y=w1347) -> (x .and. y?=w1349:bool)
            n475 = case shown="True" w1349 {
              tunnel: w1360 -> [_ w1379]
              tunnel: w1359 -> [_ w1378]
              tunnel: w1358 -> [_ w1376]
              tunnel: w1339 -> [_ w1375]
              tunnel: w1338 -> [_ w1374]
              frame False {
              }
              frame True {
                w1377 = FALSE ("prepend array or string size? (T)")
                n476 = Write to Binary File(file (use dialog)=w1375, data=w1379, 5:w1377, 9:w1376) -> ()  [unwired: 2 in, 3 out]
                n477 = Write to Binary File(file (use dialog)=w1374, data=w1378, 5:w1377, 9:w1376) -> ()  [unwired: 2 in, 3 out]
              }
            }
          }
        }
      }
    }
    frame 11 {
      n478 = while {
        shift-right: [w1442] -> _
        shift-left: 0 -> [w1443]
        tunnel: w1419 -> [w1444]
        tunnel: w1418 -> [w1441]
        tunnel: w1417 -> [w1440]
        tunnel: w1416 -> [w1439]
        tunnel: w1415 -> [w1435]
        shift-right: [w1432] -> _
        shift-left: u32 0 -> [w1433]
        tunnel: w1413 -> [w1431]
        tunnel: w1412 -> [w1430]
        tunnel: w1411 -> [w1429]
        tunnel: w1410 -> [w1428]
        tunnel: w1405 -> [w1427]
        tunnel: w1404 -> [w1426]
        tunnel: w1403 -> [w1425]
        tunnel: w1409 -> [w1424]
        tunnel: w1408 -> [w1423]
        tunnel: w1407 -> [w1422]
        tunnel: w1406 -> [w1421]
        stop <- w1434 stop-if-true
        n479 = Get Queue Status(queue=w1428) -> (queue out=w1436:refnum<queue>, # elements in queue=w1438:i32)  [unwired: 2 in, 6 out]
        n480 = Get Notifier Status(notifier=w1435) -> (current notification=w1434:bool)  [unwired: 1 in, 4 out]
        n481 = Greater Than 0?(x=w1438) -> (x > 0?=w1437:bool)
        n482 = case shown="True" w1437 {
          tunnel: w1444 -> [_ w1477]
          tunnel: w1443 -> [w1446 w1478]
          tunnel: [w1446 w1476] -> w1442
          tunnel: w1441 -> [_ w1471]
          tunnel: w1440 -> [_ w1470]
          tunnel: w1439 -> [_ w1460]
          tunnel: w1436 -> [_ w1469]
          tunnel: w1433 -> [w1445 w1466]
          tunnel: [w1445 w1465] -> w1432
          tunnel: w1431 -> [_ w1464]
          tunnel: w1430 -> [_ w1463]
          tunnel: w1429 -> [_ w1458]
          tunnel: w1427 -> [_ w1456]
          tunnel: w1426 -> [_ w1455]
          tunnel: w1425 -> [_ w1454]
          tunnel: w1424 -> [_ w1449]
          tunnel: w1423 -> [_ w1448]
          tunnel: w1422 -> [_ w1447]
          tunnel: w1421 -> [_ _]
          frame False {
          }
          frame True {
            # "False: 1st frame in fram accum"
            # "True: Last Frame of frame accum"
            # "Current Line in Frame Accum"
            # "Current Line In Frame"
            n483 = Increment(x=w1466) -> (x+1=w1459:u32)
            n484 = Dequeue Element(queue=w1469) -> (element=w1486:u64[])  [unwired: 2 in, 3 out]
            n485 = Equal?(x=w1459, y=w1463) -> (x = y?=w1468:bool)
            n486 = Greater?(x=w1459, y=w1464) -> (0:w1461:bool)
            n487 = Greater?(x=w1459, y=w1458) -> (0:w1457:bool)
            n488 = Split Number(x=w1486) -> (hi(x)=w1487:u32[], lo(x)=w1485:u32[])
            n489 = Split Number(x=w1487) -> (hi(x)=w1450:u16[], lo(x)=w1484:u16[])
            n490 = Split Number(x=w1485) -> (lo(x)=w1483:u16[])  [unwired: 1 out]
            n491 = Select(t=u32 0, s=w1468, f=w1459) -> (s? t:f=w1465:u32)
            n492 = Increment(x=w1478) -> (x+1=w1480:i32)
            n493 = Equal?(x=w1477, y=w1478) -> (x = y?=w1479:bool)
            n494 = Select(t=0, s=w1479, f=w1480) -> (s? t:f=w1476:i32)
            n495 = Build Array(0, w1478, w1477, w1478) -> (w1475:i32[])
            n496 = case shown="False" w1457 {
              tunnel: w1450 -> [w1507 w1528]
              tunnel: w1484 -> [w1503 w1527]
              tunnel: w1483 -> [w1502 w1526]
              tunnel: [w1501 w1520] -> w1473
              tunnel: [w1506 w1519] -> w1474
              tunnel: [w1500 w1518] -> w1472
              tunnel: w1475 -> [_ w1514]
              tunnel: w1470 -> [w1499 w1512]
              tunnel: w1456 -> [w1498 w1510]
              tunnel: w1455 -> [w1497 w1511]
              tunnel: w1454 -> [w1496 w1509]
              tunnel: [w1497 w1511] -> w1452
              tunnel: [w1498 w1510] -> w1453
              tunnel: [w1496 w1509] -> w1451
              frame False {
                n497 = To Single Precision Float(number=w1507) -> (single precision float=w1508:sgl[])
                n498 = To Single Precision Float(number=w1503) -> (single precision float=w1505:sgl[])
                n499 = To Single Precision Float(number=w1502) -> (single precision float=w1504:sgl[])
                n500 = Divide(x=w1508, y=w1499) -> (x/y=w1506:sgl[])
                n501 = Divide(x=w1505, y=w1499) -> (x/y=w1501:sgl[])
                n502 = Divide(x=w1504, y=w1499) -> (x/y=w1500:sgl[])
              }
              frame True {
                n503 = To Single Precision Float(number=w1528) -> (single precision float=w1513:sgl[])
                n504 = To Single Precision Float(number=w1527) -> (single precision float=w1525:sgl[])
                n505 = To Single Precision Float(number=w1526) -> (single precision float=w1524:sgl[])
                n506 = call "IMAQ GetPixelLine"("Line Coordinates"=w1514, "Image"=w1510) -> ("Pixels Line (Float)"=w1517:sgl[])  [unwired: 2 in, 4 out]
                n507 = call "IMAQ GetPixelLine"("Line Coordinates"=w1514, "Image"=w1511) -> ("Pixels Line (Float)"=w1516:sgl[])  [unwired: 2 in, 4 out]
                n508 = call "IMAQ GetPixelLine"("Line Coordinates"=w1514, "Image"=w1509) -> ("Pixels Line (Float)"=w1515:sgl[])  [unwired: 2 in, 4 out]
                n509 = Divide(x=w1513, y=w1512) -> (x/y=w1523:sgl[])
                n510 = Divide(x=w1525, y=w1512) -> (x/y=w1522:sgl[])
                n511 = Divide(x=w1524, y=w1512) -> (x/y=w1521:sgl[])
                n512 = Add(x=w1517, y=w1523) -> (x+y=w1519:sgl[])
                n513 = Add(x=w1516, y=w1522) -> (x+y=w1520:sgl[])
                n514 = Add(x=w1515, y=w1521) -> (x+y=w1518:sgl[])
              }
            }
            n515 = call "IMAQ SetPixelLine"("Pixels Line (Float)"=w1474, "Line Coordinates"=w1475, "Image"=w1453) -> ()  [unwired: 7 in, 2 out]
            n516 = call "IMAQ SetPixelLine"("Pixels Line (Float)"=w1473, "Line Coordinates"=w1475, "Image"=w1452) -> ()  [unwired: 7 in, 2 out]
            n517 = call "IMAQ SetPixelLine"("Pixels Line (Float)"=w1472, "Line Coordinates"=w1475, "Image"=w1451) -> ()  [unwired: 7 in, 2 out]
            n518 = And(x=w1461, y=w1460) -> (x .and. y?=w1462:bool)
            n519 = case shown="True" w1462 {
              tunnel: w1474 -> [_ w1495]
              tunnel: w1473 -> [_ w1494]
              tunnel: w1472 -> [_ w1493]
              tunnel: w1471 -> [_ w1491]
              tunnel: w1449 -> [_ w1490]
              tunnel: w1448 -> [_ w1489]
              tunnel: w1447 -> [_ w1488]
              frame False {
              }
              frame True {
                w1492 = FALSE ("prepend array or string size? (T)")
                n520 = Write to Binary File(file (use dialog)=w1490, data=w1495, 5:w1492, 9:w1491) -> ()  [unwired: 2 in, 3 out]
                n521 = Write to Binary File(file (use dialog)=w1489, data=w1494, 5:w1492, 9:w1491) -> ()  [unwired: 2 in, 3 out]
                n522 = Write to Binary File(file (use dialog)=w1488, data=w1493, 5:w1492, 9:w1491) -> ()  [unwired: 2 in, 3 out]
              }
            }
          }
        }
      }
    }
    frame 12 {
      n523 = while {
        shift-right: [w1566] -> _
        shift-left: 0 -> [w1567]
        tunnel: w1544 -> [w1568]
        tunnel: w1543 -> [w1565]
        tunnel: w1542 -> [w1564]
        tunnel: w1541 -> [w1563]
        tunnel: w1540 -> [w1559]
        shift-right: [w1556] -> _
        shift-left: u32 0 -> [w1557]
        tunnel: w1538 -> [w1555]
        tunnel: w1537 -> [w1554]
        tunnel: w1536 -> [w1553]
        tunnel: w1535 -> [w1552]
        tunnel: w1530 -> [w1551]
        tunnel: w1529 -> [w1550]
        tunnel: w1534 -> [w1549]
        tunnel: w1533 -> [w1548]
        tunnel: w1532 -> [w1547]
        tunnel: w1531 -> [w1546]
        stop <- w1558 stop-if-true
        n524 = Get Queue Status(queue=w1552) -> (queue out=w1560:refnum<queue>, # elements in queue=w1562:i32)  [unwired: 2 in, 6 out]
        n525 = Get Notifier Status(notifier=w1559) -> (current notification=w1558:bool)  [unwired: 1 in, 4 out]
        n526 = Greater Than 0?(x=w1562) -> (x > 0?=w1561:bool)
        n527 = case shown="True" w1561 {
          tunnel: w1568 -> [_ w1597]
          tunnel: w1567 -> [w1570 w1598]
          tunnel: [w1570 w1596] -> w1566
          tunnel: w1565 -> [_ w1592]
          tunnel: w1564 -> [_ w1591]
          tunnel: w1563 -> [_ w1581]
          tunnel: w1560 -> [_ w1590]
          tunnel: w1557 -> [w1569 w1587]
          tunnel: [w1569 w1586] -> w1556
          tunnel: w1555 -> [_ w1585]
          tunnel: w1554 -> [_ w1584]
          tunnel: w1553 -> [_ w1579]
          tunnel: w1551 -> [_ w1577]
          tunnel: w1550 -> [_ w1576]
          tunnel: w1549 -> [_ w1573]
          tunnel: w1548 -> [_ w1572]
          tunnel: w1547 -> [_ _]
          tunnel: w1546 -> [_ _]
          frame False {
          }
          frame True {
            # "False: 1st frame in fram accum"
            # "True: Last Frame of frame accum"
            # "Current Line in Frame Accum"
            # "Current Line In Frame"
            n528 = Increment(x=w1587) -> (x+1=w1580:u32)
            n529 = Dequeue Element(queue=w1590) -> (element=w1605:u64[])  [unwired: 2 in, 3 out]
            n530 = Equal?(x=w1580, y=w1584) -> (x = y?=w1589:bool)
            n531 = Greater?(x=w1580, y=w1585) -> (0:w1582:bool)
            n532 = Greater?(x=w1580, y=w1579) -> (0:w1578:bool)
            n533 = Split Number(x=w1605) -> (lo(x)=w1604:u32[])  [unwired: 1 out]
            n534 = Split Number(x=w1604) -> (hi(x)=w1571:u16[], lo(x)=w1603:u16[])
            n535 = Select(t=u32 0, s=w1589, f=w1580) -> (s? t:f=w1586:u32)
            n536 = Increment(x=w1598) -> (x+1=w1600:i32)
            n537 = Equal?(x=w1597, y=w1598) -> (x = y?=w1599:bool)
            n538 = Select(t=0, s=w1599, f=w1600) -> (s? t:f=w1596:i32)
            n539 = Build Array(0, w1598, w1597, w1598) -> (w1595:i32[])
            n540 = case shown="True" w1578 {
              tunnel: w1571 -> [w1619 w1634]
              tunnel: w1603 -> [w1616 w1633]
              tunnel: [w1618 w1629] -> w1594
              tunnel: [w1615 w1628] -> w1593
              tunnel: w1595 -> [_ w1625]
              tunnel: w1591 -> [w1614 w1623]
              tunnel: w1577 -> [w1613 w1622]
              tunnel: w1576 -> [w1612 w1621]
              tunnel: [w1613 w1622] -> w1575
              tunnel: [w1612 w1621] -> w1574
              frame False {
                n541 = To Single Precision Float(number=w1619) -> (single precision float=w1620:sgl[])
                n542 = To Single Precision Float(number=w1616) -> (single precision float=w1617:sgl[])
                n543 = Divide(x=w1620, y=w1614) -> (x/y=w1618:sgl[])
                n544 = Divide(x=w1617, y=w1614) -> (x/y=w1615:sgl[])
              }
              frame True {
                n545 = To Single Precision Float(number=w1634) -> (single precision float=w1624:sgl[])
                n546 = To Single Precision Float(number=w1633) -> (single precision float=w1632:sgl[])
                n547 = call "IMAQ GetPixelLine"("Line Coordinates"=w1625, "Image"=w1622) -> ("Pixels Line (Float)"=w1627:sgl[])  [unwired: 2 in, 4 out]
                n548 = call "IMAQ GetPixelLine"("Line Coordinates"=w1625, "Image"=w1621) -> ("Pixels Line (Float)"=w1626:sgl[])  [unwired: 2 in, 4 out]
                n549 = Divide(x=w1624, y=w1623) -> (x/y=w1631:sgl[])
                n550 = Divide(x=w1632, y=w1623) -> (x/y=w1630:sgl[])
                n551 = Add(x=w1627, y=w1631) -> (x+y=w1629:sgl[])
                n552 = Add(x=w1626, y=w1630) -> (x+y=w1628:sgl[])
              }
            }
            n553 = call "IMAQ SetPixelLine"("Pixels Line (Float)"=w1594, "Line Coordinates"=w1595, "Image"=w1575) -> ()  [unwired: 7 in, 2 out]
            n554 = call "IMAQ SetPixelLine"("Pixels Line (Float)"=w1593, "Line Coordinates"=w1595, "Image"=w1574) -> ()  [unwired: 7 in, 2 out]
            n555 = And(x=w1582, y=w1581) -> (x .and. y?=w1583:bool)
            n556 = case shown="True" w1583 {
              tunnel: w1594 -> [_ w1611]
              tunnel: w1593 -> [_ w1610]
              tunnel: w1592 -> [_ w1608]
              tunnel: w1573 -> [_ w1607]
              tunnel: w1572 -> [_ w1606]
              frame False {
              }
              frame True {
                w1609 = FALSE ("prepend array or string size? (T)")
                n557 = Write to Binary File(file (use dialog)=w1607, data=w1611, 5:w1609, 9:w1608) -> ()  [unwired: 2 in, 3 out]
                n558 = Write to Binary File(file (use dialog)=w1606, data=w1610, 5:w1609, 9:w1608) -> ()  [unwired: 2 in, 3 out]
              }
            }
          }
        }
      }
    }
    frame 13 {
      n559 = while {
        shift-right: [w1674] -> _
        shift-left: 0 -> [w1675]
        tunnel: w1651 -> [w1676]
        tunnel: w1650 -> [w1673]
        tunnel: w1649 -> [w1672]
        tunnel: w1648 -> [w1671]
        tunnel: w1647 -> [w1667]
        shift-right: [w1664] -> _
        shift-left: u32 0 -> [w1665]
        tunnel: w1645 -> [w1663]
        tunnel: w1644 -> [w1662]
        tunnel: w1643 -> [w1661]
        tunnel: w1642 -> [w1660]
        tunnel: w1637 -> [w1659]
        tunnel: w1636 -> [w1658]
        tunnel: w1635 -> [w1657]
        tunnel: w1641 -> [w1656]
        tunnel: w1640 -> [w1655]
        tunnel: w1639 -> [w1654]
        tunnel: w1638 -> [w1653]
        stop <- w1666 stop-if-true
        n560 = Get Queue Status(queue=w1660) -> (queue out=w1668:refnum<queue>, # elements in queue=w1670:i32)  [unwired: 2 in, 6 out]
        n561 = Get Notifier Status(notifier=w1667) -> (current notification=w1666:bool)  [unwired: 1 in, 4 out]
        n562 = Greater Than 0?(x=w1670) -> (x > 0?=w1669:bool)
        n563 = case shown="True" w1669 {
          tunnel: w1676 -> [_ w1709]
          tunnel: w1675 -> [w1678 w1710]
          tunnel: [w1678 w1708] -> w1674
          tunnel: w1673 -> [_ w1703]
          tunnel: w1672 -> [_ w1702]
          tunnel: w1671 -> [_ w1692]
          tunnel: w1668 -> [_ w1701]
          tunnel: w1665 -> [w1677 w1698]
          tunnel: [w1677 w1697] -> w1664
          tunnel: w1663 -> [_ w1696]
          tunnel: w1662 -> [_ w1695]
          tunnel: w1661 -> [_ w1690]
          tunnel: w1659 -> [_ w1688]
          tunnel: w1658 -> [_ w1687]
          tunnel: w1657 -> [_ w1686]
          tunnel: w1656 -> [_ w1681]
          tunnel: w1655 -> [_ w1680]
          tunnel: w1654 -> [_ w1679]
          tunnel: w1653 -> [_ _]
          frame False {
          }
          frame True {
            # "False: 1st frame in fram accum"
            # "True: Last Frame of frame accum"
            # "Current Line in Frame Accum"
            # "Current Line In Frame"
            n564 = Increment(x=w1698) -> (x+1=w1691:u32)
            n565 = Dequeue Element(queue=w1701) -> (element=w1718:u64[])  [unwired: 2 in, 3 out]
            n566 = Equal?(x=w1691, y=w1695) -> (x = y?=w1700:bool)
            n567 = Greater?(x=w1691, y=w1696) -> (0:w1693:bool)
            n568 = Greater?(x=w1691, y=w1690) -> (0:w1689:bool)
            n569 = Split Number(x=w1718) -> (hi(x)=w1719:u32[], lo(x)=w1717:u32[])
            n570 = Split Number(x=w1719) -> (hi(x)=w1682:u16[])  [unwired: 1 out]
            n571 = Split Number(x=w1717) -> (hi(x)=w1716:u16[], lo(x)=w1715:u16[])
            n572 = Select(t=u32 0, s=w1700, f=w1691) -> (s? t:f=w1697:u32)
            n573 = Increment(x=w1710) -> (x+1=w1712:i32)
            n574 = Equal?(x=w1709, y=w1710) -> (x = y?=w1711:bool)
            n575 = Select(t=0, s=w1711, f=w1712) -> (s? t:f=w1708:i32)
            n576 = Build Array(0, w1710, w1709, w1710) -> (w1707:i32[])
            n577 = case shown="True" w1689 {
              tunnel: w1682 -> [w1739 w1760]
              tunnel: w1716 -> [w1735 w1759]
              tunnel: w1715 -> [w1734 w1758]
              tunnel: [w1733 w1752] -> w1705
              tunnel: [w1738 w1751] -> w1706
              tunnel: [w1732 w1750] -> w1704
              tunnel: w1707 -> [_ w1746]
              tunnel: w1702 -> [w1731 w1744]
              tunnel: w1688 -> [w1730 w1742]
              tunnel: w1687 -> [w1729 w1743]
              tunnel: w1686 -> [w1728 w1741]
              tunnel: [w1729 w1743] -> w1684
              tunnel: [w1730 w1742] -> w1685
              tunnel: [w1728 w1741] -> w1683
              frame False {
                n578 = To Single Precision Float(number=w1739) -> (single precision float=w1740:sgl[])
                n579 = To Single Precision Float(number=w1735) -> (single precision float=w1737:sgl[])
                n580 = To Single Precision Float(number=w1734) -> (single precision float=w1736:sgl[])
                n581 = Divide(x=w1740, y=w1731) -> (x/y=w1738:sgl[])
                n582 = Divide(x=w1737, y=w1731) -> (x/y=w1733:sgl[])
                n583 = Divide(x=w1736, y=w1731) -> (x/y=w1732:sgl[])
              }
              frame True {
                n584 = To Single Precision Float(number=w1760) -> (single precision float=w1745:sgl[])
                n585 = To Single Precision Float(number=w1759) -> (single precision float=w1757:sgl[])
                n586 = To Single Precision Float(number=w1758) -> (single precision float=w1756:sgl[])
                n587 = call "IMAQ GetPixelLine"("Line Coordinates"=w1746, "Image"=w1742) -> ("Pixels Line (Float)"=w1749:sgl[])  [unwired: 2 in, 4 out]
                n588 = call "IMAQ GetPixelLine"("Line Coordinates"=w1746, "Image"=w1743) -> ("Pixels Line (Float)"=w1748:sgl[])  [unwired: 2 in, 4 out]
                n589 = call "IMAQ GetPixelLine"("Line Coordinates"=w1746, "Image"=w1741) -> ("Pixels Line (Float)"=w1747:sgl[])  [unwired: 2 in, 4 out]
                n590 = Divide(x=w1745, y=w1744) -> (x/y=w1755:sgl[])
                n591 = Divide(x=w1757, y=w1744) -> (x/y=w1754:sgl[])
                n592 = Divide(x=w1756, y=w1744) -> (x/y=w1753:sgl[])
                n593 = Add(x=w1749, y=w1755) -> (x+y=w1751:sgl[])
                n594 = Add(x=w1748, y=w1754) -> (x+y=w1752:sgl[])
                n595 = Add(x=w1747, y=w1753) -> (x+y=w1750:sgl[])
              }
            }
            n596 = call "IMAQ SetPixelLine"("Pixels Line (Float)"=w1706, "Line Coordinates"=w1707, "Image"=w1685) -> ()  [unwired: 7 in, 2 out]
            n597 = call "IMAQ SetPixelLine"("Pixels Line (Float)"=w1705, "Line Coordinates"=w1707, "Image"=w1684) -> ()  [unwired: 7 in, 2 out]
            n598 = call "IMAQ SetPixelLine"("Pixels Line (Float)"=w1704, "Line Coordinates"=w1707, "Image"=w1683) -> ()  [unwired: 7 in, 2 out]
            n599 = And(x=w1693, y=w1692) -> (x .and. y?=w1694:bool)
            n600 = case shown="True" w1694 {
              tunnel: w1706 -> [_ w1727]
              tunnel: w1705 -> [_ w1726]
              tunnel: w1704 -> [_ w1725]
              tunnel: w1703 -> [_ w1723]
              tunnel: w1681 -> [_ w1722]
              tunnel: w1680 -> [_ w1721]
              tunnel: w1679 -> [_ w1720]
              frame False {
              }
              frame True {
                w1724 = FALSE ("prepend array or string size? (T)")
                n601 = Write to Binary File(file (use dialog)=w1722, data=w1727, 5:w1724, 9:w1723) -> ()  [unwired: 2 in, 3 out]
                n602 = Write to Binary File(file (use dialog)=w1721, data=w1726, 5:w1724, 9:w1723) -> ()  [unwired: 2 in, 3 out]
                n603 = Write to Binary File(file (use dialog)=w1720, data=w1725, 5:w1724, 9:w1723) -> ()  [unwired: 2 in, 3 out]
              }
            }
          }
        }
      }
    }
    frame 14 {
      n604 = while {
        shift-right: [w1800] -> _
        shift-left: 0 -> [w1801]
        tunnel: w1777 -> [w1802]
        tunnel: w1776 -> [w1799]
        tunnel: w1775 -> [w1798]
        tunnel: w1774 -> [w1797]
        tunnel: w1773 -> [w1793]
        shift-right: [w1790] -> _
        shift-left: u32 0 -> [w1791]
        tunnel: w1771 -> [w1789]
        tunnel: w1770 -> [w1788]
        tunnel: w1769 -> [w1787]
        tunnel: w1768 -> [w1786]
        tunnel: w1763 -> [w1781]
        tunnel: w1762 -> [w1780]
        tunnel: w1761 -> [w1779]
        tunnel: w1767 -> [w1785]
        tunnel: w1766 -> [w1784]
        tunnel: w1765 -> [w1783]
        tunnel: w1764 -> [w1782]
        stop <- w1792 stop-if-true
        n605 = Get Queue Status(queue=w1786) -> (queue out=w1794:refnum<queue>, # elements in queue=w1796:i32)  [unwired: 2 in, 6 out]
        n606 = Get Notifier Status(notifier=w1793) -> (current notification=w1792:bool)  [unwired: 1 in, 4 out]
        n607 = Greater Than 0?(x=w1796) -> (x > 0?=w1795:bool)
        n608 = case shown="True" w1795 {
          tunnel: w1802 -> [_ w1834]
          tunnel: w1801 -> [w1804 w1835]
          tunnel: [w1804 w1833] -> w1800
          tunnel: w1799 -> [_ w1828]
          tunnel: w1798 -> [_ w1827]
          tunnel: w1797 -> [_ w1817]
          tunnel: w1794 -> [_ w1826]
          tunnel: w1791 -> [w1803 w1823]
          tunnel: [w1803 w1822] -> w1790
          tunnel: w1789 -> [_ w1821]
          tunnel: w1788 -> [_ w1820]
          tunnel: w1787 -> [_ w1815]
          tunnel: w1781 -> [_ w1813]
          tunnel: w1780 -> [_ w1812]
          tunnel: w1779 -> [_ w1811]
          tunnel: w1785 -> [_ w1807]
          tunnel: w1784 -> [_ w1806]
          tunnel: w1783 -> [_ w1805]
          tunnel: w1782 -> [_ _]
          frame False {
          }
          frame True {
            # "False: 1st frame in fram accum"
            # "True: Last Frame of frame accum"
            # "Current Line in Frame Accum"
            # "Current Line In Frame"
            n609 = Increment(x=w1823) -> (x+1=w1816:u32)
            n610 = Dequeue Element(queue=w1826) -> (element=w1844:u64[])  [unwired: 2 in, 3 out]
            n611 = Equal?(x=w1816, y=w1820) -> (x = y?=w1825:bool)
            n612 = Greater?(x=w1816, y=w1821) -> (0:w1818:bool)
            n613 = Greater?(x=w1816, y=w1815) -> (0:w1814:bool)
            n614 = Split Number(x=w1844) -> (hi(x)=w1845:u32[], lo(x)=w1843:u32[])
            n615 = Split Number(x=w1845) -> (lo(x)=w1842:u16[])  [unwired: 1 out]
            n616 = Split Number(x=w1843) -> (hi(x)=w1841:u16[], lo(x)=w1840:u16[])
            n617 = Select(t=u32 0, s=w1825, f=w1816) -> (s? t:f=w1822:u32)
            n618 = Increment(x=w1835) -> (x+1=w1837:i32)
            n619 = Equal?(x=w1834, y=w1835) -> (x = y?=w1836:bool)
            n620 = Select(t=0, s=w1836, f=w1837) -> (s? t:f=w1833:i32)
            n621 = Build Array(0, w1835, w1834, w1835) -> (w1832:i32[])
            n622 = case shown="True" w1814 {
              tunnel: w1842 -> [w1863 w1886]
              tunnel: w1841 -> [w1862 w1885]
              tunnel: w1840 -> [w1861 w1884]
              tunnel: [w1859 w1877] -> w1830
              tunnel: [w1860 w1876] -> w1831
              tunnel: [w1858 w1875] -> w1829
              tunnel: w1832 -> [_ w1871]
              tunnel: w1827 -> [w1857 w1870]
              tunnel: w1813 -> [w1856 w1868]
              tunnel: w1812 -> [w1855 w1869]
              tunnel: w1811 -> [w1854 w1867]
              tunnel: [w1855 w1869] -> w1809
              tunnel: [w1856 w1868] -> w1810
              tunnel: [w1854 w1867] -> w1808
              frame False {
                n623 = To Single Precision Float(number=w1863) -> (single precision float=w1866:sgl[])
                n624 = To Single Precision Float(number=w1862) -> (single precision float=w1865:sgl[])
                n625 = To Single Precision Float(number=w1861) -> (single precision float=w1864:sgl[])
                n626 = Divide(x=w1866, y=w1857) -> (x/y=w1860:sgl[])
                n627 = Divide(x=w1865, y=w1857) -> (x/y=w1859:sgl[])
                n628 = Divide(x=w1864, y=w1857) -> (x/y=w1858:sgl[])
              }
              frame True {
                n629 = To Single Precision Float(number=w1886) -> (single precision float=w1883:sgl[])
                n630 = To Single Precision Float(number=w1885) -> (single precision float=w1882:sgl[])
                n631 = To Single Precision Float(number=w1884) -> (single precision float=w1881:sgl[])
                n632 = call "IMAQ GetPixelLine"("Line Coordinates"=w1871, "Image"=w1868) -> ("Pixels Line (Float)"=w1874:sgl[])  [unwired: 2 in, 4 out]
                n633 = call "IMAQ GetPixelLine"("Line Coordinates"=w1871, "Image"=w1869) -> ("Pixels Line (Float)"=w1873:sgl[])  [unwired: 2 in, 4 out]
                n634 = call "IMAQ GetPixelLine"("Line Coordinates"=w1871, "Image"=w1867) -> ("Pixels Line (Float)"=w1872:sgl[])  [unwired: 2 in, 4 out]
                n635 = Divide(x=w1883, y=w1870) -> (x/y=w1880:sgl[])
                n636 = Divide(x=w1882, y=w1870) -> (x/y=w1879:sgl[])
                n637 = Divide(x=w1881, y=w1870) -> (x/y=w1878:sgl[])
                n638 = Add(x=w1874, y=w1880) -> (x+y=w1876:sgl[])
                n639 = Add(x=w1873, y=w1879) -> (x+y=w1877:sgl[])
                n640 = Add(x=w1872, y=w1878) -> (x+y=w1875:sgl[])
              }
            }
            n641 = call "IMAQ SetPixelLine"("Pixels Line (Float)"=w1831, "Line Coordinates"=w1832, "Image"=w1810) -> ()  [unwired: 7 in, 2 out]
            n642 = call "IMAQ SetPixelLine"("Pixels Line (Float)"=w1830, "Line Coordinates"=w1832, "Image"=w1809) -> ()  [unwired: 7 in, 2 out]
            n643 = call "IMAQ SetPixelLine"("Pixels Line (Float)"=w1829, "Line Coordinates"=w1832, "Image"=w1808) -> ()  [unwired: 7 in, 2 out]
            n644 = And(x=w1818, y=w1817) -> (x .and. y?=w1819:bool)
            n645 = case shown="True" w1819 {
              tunnel: w1831 -> [_ w1853]
              tunnel: w1830 -> [_ w1852]
              tunnel: w1829 -> [_ w1851]
              tunnel: w1828 -> [_ w1849]
              tunnel: w1807 -> [_ w1848]
              tunnel: w1806 -> [_ w1847]
              tunnel: w1805 -> [_ w1846]
              frame False {
              }
              frame True {
                w1850 = FALSE ("prepend array or string size? (T)")
                n646 = Write to Binary File(file (use dialog)=w1848, data=w1853, 5:w1850, 9:w1849) -> ()  [unwired: 2 in, 3 out]
                n647 = Write to Binary File(file (use dialog)=w1847, data=w1852, 5:w1850, 9:w1849) -> ()  [unwired: 2 in, 3 out]
                n648 = Write to Binary File(file (use dialog)=w1846, data=w1851, 5:w1850, 9:w1849) -> ()  [unwired: 2 in, 3 out]
              }
            }
          }
        }
      }
    }
    frame 15 {
      n649 = while {
        shift-right: [w1928] -> _
        shift-left: 0 -> [w1929]
        tunnel: w1904 -> [w1930]
        tunnel: w1903 -> [w1927]
        tunnel: w1902 -> [w1926]
        tunnel: w1901 -> [w1925]
        tunnel: w1900 -> [w1921]
        shift-right: [w1918] -> _
        shift-left: u32 0 -> [w1919]
        tunnel: w1898 -> [w1917]
        tunnel: w1897 -> [w1916]
        tunnel: w1896 -> [w1915]
        tunnel: w1895 -> [w1914]
        tunnel: w1890 -> [w1913]
        tunnel: w1889 -> [w1912]
        tunnel: w1888 -> [w1911]
        tunnel: w1887 -> [w1910]
        tunnel: w1894 -> [w1909]
        tunnel: w1893 -> [w1908]
        tunnel: w1892 -> [w1907]
        tunnel: w1891 -> [w1906]
        stop <- w1920 stop-if-true
        n650 = Get Queue Status(queue=w1914) -> (queue out=w1922:refnum<queue>, # elements in queue=w1924:i32)  [unwired: 2 in, 6 out]
        n651 = Get Notifier Status(notifier=w1921) -> (current notification=w1920:bool)  [unwired: 1 in, 4 out]
        n652 = Greater Than 0?(x=w1924) -> (x > 0?=w1923:bool)
        n653 = case shown="True" w1923 {
          tunnel: w1930 -> [_ w1967]
          tunnel: w1929 -> [w1932 w1968]
          tunnel: [w1932 w1966] -> w1928
          tunnel: w1927 -> [_ w1960]
          tunnel: w1926 -> [_ w1959]
          tunnel: w1925 -> [_ w1949]
          tunnel: w1922 -> [_ w1958]
          tunnel: w1919 -> [w1931 w1955]
          tunnel: [w1931 w1954] -> w1918
          tunnel: w1917 -> [_ w1953]
          tunnel: w1916 -> [_ w1952]
          tunnel: w1915 -> [_ w1947]
          tunnel: w1913 -> [_ w1945]
          tunnel: w1912 -> [_ w1944]
          tunnel: w1911 -> [_ w1943]
          tunnel: w1910 -> [_ w1942]
          tunnel: w1909 -> [_ w1936]
          tunnel: w1908 -> [_ w1935]
          tunnel: w1907 -> [_ w1934]
          tunnel: w1906 -> [_ w1933]
          frame False {
          }
          frame True {
            # "False: 1st frame in fram accum"
            # "True: Last Frame of frame accum"
            # "Current Line in Frame Accum"
            # "Current Line In Frame"
            n654 = Increment(x=w1955) -> (x+1=w1948:u32)
            n655 = Dequeue Element(queue=w1958) -> (element=w1977:u64[])  [unwired: 2 in, 3 out]
            n656 = Equal?(x=w1948, y=w1952) -> (x = y?=w1957:bool)
            n657 = Greater?(x=w1948, y=w1953) -> (0:w1950:bool)
            n658 = Greater?(x=w1948, y=w1947) -> (0:w1946:bool)
            n659 = Split Number(x=w1977) -> (hi(x)=w1978:u32[], lo(x)=w1976:u32[])
            n660 = Split Number(x=w1978) -> (hi(x)=w1937:u16[], lo(x)=w1975:u16[])
            n661 = Split Number(x=w1976) -> (hi(x)=w1974:u16[], lo(x)=w1973:u16[])
            n662 = Select(t=u32 0, s=w1957, f=w1948) -> (s? t:f=w1954:u32)
            n663 = Increment(x=w1968) -> (x+1=w1970:i32)
            n664 = Equal?(x=w1967, y=w1968) -> (x = y?=w1969:bool)
            n665 = Select(t=0, s=w1969, f=w1970) -> (s? t:f=w1966:i32)
            n666 = Build Array(0, w1968, w1967, w1968) -> (w1965:i32[])
            n667 = case shown="True" w1946 {
              tunnel: w1937 -> [w2004 w2031]
              tunnel: w1975 -> [w1999 w2030]
              tunnel: w1974 -> [w1998 w2029]
              tunnel: w1973 -> [w1997 w2028]
              tunnel: [w1995 w2020] -> w1962
              tunnel: [w1996 w2019] -> w1963
              tunnel: [w2003 w2018] -> w1964
              tunnel: [w1994 w2017] -> w1961
              tunnel: w1965 -> [_ w2012]
              tunnel: w1959 -> [w1993 w2010]
              tunnel: w1945 -> [w1992 w2007]
              tunnel: w1944 -> [w1991 w2008]
              tunnel: w1943 -> [w1990 w2009]
              tunnel: w1942 -> [w1989 w2006]
              tunnel: [w1990 w2009] -> w1939
              tunnel: [w1991 w2008] -> w1940
              tunnel: [w1992 w2007] -> w1941
              tunnel: [w1989 w2006] -> w1938
              frame False {
                n668 = To Single Precision Float(number=w2004) -> (single precision float=w2005:sgl[])
                n669 = To Single Precision Float(number=w1999) -> (single precision float=w2002:sgl[])
                n670 = To Single Precision Float(number=w1998) -> (single precision float=w2001:sgl[])
                n671 = To Single Precision Float(number=w1997) -> (single precision float=w2000:sgl[])
                n672 = Divide(x=w2005, y=w1993) -> (x/y=w2003:sgl[])
                n673 = Divide(x=w2002, y=w1993) -> (x/y=w1996:sgl[])
                n674 = Divide(x=w2001, y=w1993) -> (x/y=w1995:sgl[])
                n675 = Divide(x=w2000, y=w1993) -> (x/y=w1994:sgl[])
              }
              frame True {
                n676 = To Single Precision Float(number=w2031) -> (single precision float=w2011:sgl[])
                n677 = To Single Precision Float(number=w2030) -> (single precision float=w2027:sgl[])
                n678 = To Single Precision Float(number=w2029) -> (single precision float=w2026:sgl[])
                n679 = To Single Precision Float(number=w2028) -> (single precision float=w2025:sgl[])
                n680 = call "IMAQ GetPixelLine"("Line Coordinates"=w2012, "Image"=w2007) -> ("Pixels Line (Float)"=w2016:sgl[])  [unwired: 2 in, 4 out]
                n681 = call "IMAQ GetPixelLine"("Line Coordinates"=w2012, "Image"=w2008) -> ("Pixels Line (Float)"=w2015:sgl[])  [unwired: 2 in, 4 out]
                n682 = call "IMAQ GetPixelLine"("Line Coordinates"=w2012, "Image"=w2009) -> ("Pixels Line (Float)"=w2014:sgl[])  [unwired: 2 in, 4 out]
                n683 = call "IMAQ GetPixelLine"("Line Coordinates"=w2012, "Image"=w2006) -> ("Pixels Line (Float)"=w2013:sgl[])  [unwired: 2 in, 4 out]
                n684 = Divide(x=w2011, y=w2010) -> (x/y=w2024:sgl[])
                n685 = Divide(x=w2027, y=w2010) -> (x/y=w2023:sgl[])
                n686 = Divide(x=w2026, y=w2010) -> (x/y=w2022:sgl[])
                n687 = Divide(x=w2025, y=w2010) -> (x/y=w2021:sgl[])
                n688 = Add(x=w2016, y=w2024) -> (x+y=w2018:sgl[])
                n689 = Add(x=w2015, y=w2023) -> (x+y=w2019:sgl[])
                n690 = Add(x=w2014, y=w2022) -> (x+y=w2020:sgl[])
                n691 = Add(x=w2013, y=w2021) -> (x+y=w2017:sgl[])
              }
            }
            n692 = call "IMAQ SetPixelLine"("Pixels Line (Float)"=w1964, "Line Coordinates"=w1965, "Image"=w1941) -> ()  [unwired: 7 in, 2 out]
            n693 = call "IMAQ SetPixelLine"("Pixels Line (Float)"=w1963, "Line Coordinates"=w1965, "Image"=w1940) -> ()  [unwired: 7 in, 2 out]
            n694 = call "IMAQ SetPixelLine"("Pixels Line (Float)"=w1962, "Line Coordinates"=w1965, "Image"=w1939) -> ()  [unwired: 7 in, 2 out]
            n695 = call "IMAQ SetPixelLine"("Pixels Line (Float)"=w1961, "Line Coordinates"=w1965, "Image"=w1938) -> ()  [unwired: 7 in, 2 out]
            n696 = And(x=w1950, y=w1949) -> (x .and. y?=w1951:bool)
            n697 = case shown="True" w1951 {
              tunnel: w1964 -> [_ w1988]
              tunnel: w1963 -> [_ w1987]
              tunnel: w1962 -> [_ w1986]
              tunnel: w1961 -> [_ w1985]
              tunnel: w1960 -> [_ w1983]
              tunnel: w1936 -> [_ w1982]
              tunnel: w1935 -> [_ w1981]
              tunnel: w1934 -> [_ w1980]
              tunnel: w1933 -> [_ w1979]
              frame False {
              }
              frame True {
                w1984 = FALSE ("prepend array or string size? (T)")
                n698 = Write to Binary File(file (use dialog)=w1982, data=w1988, 5:w1984, 9:w1983) -> ()  [unwired: 2 in, 3 out]
                n699 = Write to Binary File(file (use dialog)=w1981, data=w1987, 5:w1984, 9:w1983) -> ()  [unwired: 2 in, 3 out]
                n700 = Write to Binary File(file (use dialog)=w1980, data=w1986, 5:w1984, 9:w1983) -> ()  [unwired: 2 in, 3 out]
                n701 = Write to Binary File(file (use dialog)=w1979, data=w1985, 5:w1984, 9:w1983) -> ()  [unwired: 2 in, 3 out]
              }
            }
          }
        }
      }
    }
    frame 19 {
      n702 = while {
        shift-right: [w2067] -> _
        shift-left: 0 -> [w2068]
        tunnel: w2046 -> [w2069]
        tunnel: w2045 -> [w2066]
        tunnel: w2044 -> [w2065]
        tunnel: w2043 -> [w2064]
        tunnel: w2042 -> [w2060]
        shift-right: [w2057] -> _
        shift-left: u32 0 -> [w2058]
        tunnel: w2040 -> [w2056]
        tunnel: w2039 -> [w2055]
        tunnel: w2038 -> [w2054]
        tunnel: w2037 -> [w2053]
        tunnel: w2032 -> [w2052]
        tunnel: w2036 -> [w2051]
        tunnel: w2035 -> [w2050]
        tunnel: w2034 -> [w2049]
        tunnel: w2033 -> [w2048]
        stop <- w2059 stop-if-true
        n703 = Get Queue Status(queue=w2053) -> (queue out=w2061:refnum<queue>, # elements in queue=w2063:i32)  [unwired: 2 in, 6 out]
        n704 = Get Notifier Status(notifier=w2060) -> (current notification=w2059:bool)  [unwired: 1 in, 4 out]
        n705 = Greater Than 0?(x=w2063) -> (x > 0?=w2062:bool)
        n706 = case shown="True" w2062 {
          tunnel: w2069 -> [_ w2098]
          tunnel: w2068 -> [w2071 w2099]
          tunnel: [w2071 w2097] -> w2067
          tunnel: w2066 -> [_ w2094]
          tunnel: w2065 -> [_ w2093]
          tunnel: w2064 -> [_ w2083]
          tunnel: w2061 -> [_ w2092]
          tunnel: w2058 -> [w2070 w2089]
          tunnel: [w2070 w2088] -> w2057
          tunnel: w2056 -> [_ w2087]
          tunnel: w2055 -> [_ w2086]
          tunnel: w2054 -> [_ w2081]
          tunnel: w2052 -> [_ w2079]
          tunnel: w2051 -> [_ w2077]
          tunnel: w2050 -> [_ _]
          tunnel: w2049 -> [_ _]
          tunnel: w2048 -> [_ _]
          frame False {
          }
          frame True {
            # "True: Last Frame of frame accum"
            # "Current Line in Frame Accum"
            # "Current Line In Frame"
            n707 = Increment(x=w2089) -> (x+1=w2082:u32)
            n708 = Dequeue Element(queue=w2092) -> (element=w2104:u64[])  [unwired: 2 in, 3 out]
            n709 = Equal?(x=w2082, y=w2086) -> (x = y?=w2091:bool)
            n710 = Greater?(x=w2082, y=w2087) -> (0:w2084:bool)
            n711 = Greater?(x=w2082, y=w2081) -> (0:w2080:bool)
            n712 = Split Number(x=w2104) -> (hi(x)=w2105:u32[])  [unwired: 1 out]
            n713 = Split Number(x=w2105) -> (hi(x)=w2076:u16[], lo(x)=w2075:u16[])
            n714 = Select(t=u32 0, s=w2091, f=w2082) -> (s? t:f=w2088:u32)
            n715 = Increment(x=w2099) -> (x+1=w2101:i32)
            n716 = Equal?(x=w2098, y=w2099) -> (x = y?=w2100:bool)
            n717 = To Single Precision Float(number=w2076) -> (single precision float=w2074:sgl[])
            n718 = To Single Precision Float(number=w2075) -> (single precision float=w2073:sgl[])
            n719 = Select(t=0, s=w2100, f=w2101) -> (s? t:f=w2097:i32)
            n720 = Add(x=w2074, y=w2073) -> (x+y=w2072:sgl[])
            n721 = Build Array(0, w2099, w2098, w2099) -> (w2096:i32[])
            n722 = case shown="False" w2080 {
              tunnel: [w2113 w2119] -> w2095
              tunnel: w2096 -> [_ w2117]
              tunnel: w2093 -> [w2112 w2116]
              tunnel: w2079 -> [w2111 w2115]
              tunnel: [w2111 w2115] -> w2078
              tunnel: w2072 -> [w2110 w2114]
              frame False {
                n723 = Divide(x=w2110, y=w2112) -> (x/y=w2113:sgl[])
              }
              frame True {
                n724 = call "IMAQ GetPixelLine"("Line Coordinates"=w2117, "Image"=w2115) -> ("Pixels Line (Float)"=w2118:sgl[])  [unwired: 2 in, 4 out]
                n725 = Divide(x=w2114, y=w2116) -> (x/y=w2120:sgl[])
                n726 = Add(x=w2118, y=w2120) -> (x+y=w2119:sgl[])
              }
            }
            n727 = call "IMAQ SetPixelLine"("Pixels Line (Float)"=w2095, "Line Coordinates"=w2096, "Image"=w2078) -> ()  [unwired: 7 in, 2 out]
            n728 = And(x=w2084, y=w2083) -> (x .and. y?=w2085:bool)
            n729 = case shown="True" w2085 {
              tunnel: w2095 -> [_ w2109]
              tunnel: w2094 -> [_ w2107]
              tunnel: w2077 -> [_ w2106]
              frame False {
              }
              frame True {
                n730 = Write to Binary File(file (use dialog)=w2106, data=w2109, 5:FALSE ("prepend array or string size? (T)"), 9:w2107) -> ()  [unwired: 2 in, 3 out]
              }
            }
          }
        }
      }
    }
    frame 21 {
      n731 = while {
        shift-right: [w2156] -> _
        shift-left: 0 -> [w2157]
        tunnel: w2135 -> [w2158]
        tunnel: w2134 -> [w2155]
        tunnel: w2133 -> [w2154]
        tunnel: w2132 -> [w2153]
        tunnel: w2131 -> [w2149]
        shift-right: [w2146] -> _
        shift-left: u32 0 -> [w2147]
        tunnel: w2129 -> [w2145]
        tunnel: w2128 -> [w2144]
        tunnel: w2127 -> [w2143]
        tunnel: w2126 -> [w2142]
        tunnel: w2121 -> [w2141]
        tunnel: w2125 -> [w2140]
        tunnel: w2124 -> [w2139]
        tunnel: w2123 -> [w2138]
        tunnel: w2122 -> [w2137]
        stop <- w2148 stop-if-true
        n732 = Get Queue Status(queue=w2142) -> (queue out=w2150:refnum<queue>, # elements in queue=w2152:i32)  [unwired: 2 in, 6 out]
        n733 = Get Notifier Status(notifier=w2149) -> (current notification=w2148:bool)  [unwired: 1 in, 4 out]
        n734 = Greater Than 0?(x=w2152) -> (x > 0?=w2151:bool)
        n735 = case shown="True" w2151 {
          tunnel: w2158 -> [_ w2187]
          tunnel: w2157 -> [w2160 w2188]
          tunnel: [w2160 w2186] -> w2156
          tunnel: w2155 -> [_ w2183]
          tunnel: w2154 -> [_ w2182]
          tunnel: w2153 -> [_ w2172]
          tunnel: w2150 -> [_ w2181]
          tunnel: w2147 -> [w2159 w2178]
          tunnel: [w2159 w2177] -> w2146
          tunnel: w2145 -> [_ w2176]
          tunnel: w2144 -> [_ w2175]
          tunnel: w2143 -> [_ w2170]
          tunnel: w2141 -> [_ w2168]
          tunnel: w2140 -> [_ w2166]
          tunnel: w2139 -> [_ _]
          tunnel: w2138 -> [_ _]
          tunnel: w2137 -> [_ _]
          frame False {
          }
          frame True {
            # "True: Last Frame of frame accum"
            # "Current Line in Frame Accum"
            # "Current Line In Frame"
            n736 = Increment(x=w2178) -> (x+1=w2171:u32)
            n737 = Dequeue Element(queue=w2181) -> (element=w2194:u64[])  [unwired: 2 in, 3 out]
            n738 = Equal?(x=w2171, y=w2175) -> (x = y?=w2180:bool)
            n739 = Greater?(x=w2171, y=w2176) -> (0:w2173:bool)
            n740 = Greater?(x=w2171, y=w2170) -> (0:w2169:bool)
            n741 = Split Number(x=w2194) -> (hi(x)=w2195:u32[], lo(x)=w2193:u32[])
            n742 = Split Number(x=w2195) -> (hi(x)=w2165:u16[])  [unwired: 1 out]
            n743 = Split Number(x=w2193) -> (hi(x)=w2161:u16[])  [unwired: 1 out]
            n744 = Select(t=u32 0, s=w2180, f=w2171) -> (s? t:f=w2177:u32)
            n745 = Increment(x=w2188) -> (x+1=w2190:i32)
            n746 = Equal?(x=w2187, y=w2188) -> (x = y?=w2189:bool)
            n747 = To Single Precision Float(number=w2165) -> (single precision float=w2164:sgl[])
            n748 = To Single Precision Float(number=w2161) -> (single precision float=w2163:sgl[])
            n749 = Select(t=0, s=w2189, f=w2190) -> (s? t:f=w2186:i32)
            n750 = Add(x=w2164, y=w2163) -> (x+y=w2162:sgl[])
            n751 = Build Array(0, w2188, w2187, w2188) -> (w2185:i32[])
            n752 = case shown="False" w2169 {
              tunnel: [w2203 w2209] -> w2184
              tunnel: w2185 -> [_ w2207]
              tunnel: w2182 -> [w2202 w2206]
              tunnel: w2168 -> [w2201 w2205]
              tunnel: [w2201 w2205] -> w2167
              tunnel: w2162 -> [w2200 w2204]
              frame False {
                n753 = Divide(x=w2200, y=w2202) -> (x/y=w2203:sgl[])
              }
              frame True {
                n754 = call "IMAQ GetPixelLine"("Line Coordinates"=w2207, "Image"=w2205) -> ("Pixels Line (Float)"=w2208:sgl[])  [unwired: 2 in, 4 out]
                n755 = Divide(x=w2204, y=w2206) -> (x/y=w2210:sgl[])
                n756 = Add(x=w2208, y=w2210) -> (x+y=w2209:sgl[])
              }
            }
            n757 = call "IMAQ SetPixelLine"("Pixels Line (Float)"=w2184, "Line Coordinates"=w2185, "Image"=w2167) -> ()  [unwired: 7 in, 2 out]
            n758 = And(x=w2173, y=w2172) -> (x .and. y?=w2174:bool)
            n759 = case shown="True" w2174 {
              tunnel: w2184 -> [_ w2199]
              tunnel: w2183 -> [_ w2197]
              tunnel: w2166 -> [_ w2196]
              frame False {
              }
              frame True {
                n760 = Write to Binary File(file (use dialog)=w2196, data=w2199, 5:FALSE ("prepend array or string size? (T)"), 9:w2197) -> ()  [unwired: 2 in, 3 out]
              }
            }
          }
        }
      }
    }
    frame 22 {
      n761 = while {
        shift-right: [w2246] -> _
        shift-left: 0 -> [w2247]
        tunnel: w2225 -> [w2248]
        tunnel: w2224 -> [w2245]
        tunnel: w2223 -> [w2244]
        tunnel: w2222 -> [w2243]
        tunnel: w2221 -> [w2239]
        shift-right: [w2236] -> _
        shift-left: u32 0 -> [w2237]
        tunnel: w2219 -> [w2235]
        tunnel: w2218 -> [w2234]
        tunnel: w2217 -> [w2233]
        tunnel: w2216 -> [w2232]
        tunnel: w2211 -> [w2231]
        tunnel: w2215 -> [w2230]
        tunnel: w2214 -> [w2229]
        tunnel: w2213 -> [w2228]
        tunnel: w2212 -> [w2227]
        stop <- w2238 stop-if-true
        n762 = Get Queue Status(queue=w2232) -> (queue out=w2240:refnum<queue>, # elements in queue=w2242:i32)  [unwired: 2 in, 6 out]
        n763 = Get Notifier Status(notifier=w2239) -> (current notification=w2238:bool)  [unwired: 1 in, 4 out]
        n764 = Greater Than 0?(x=w2242) -> (x > 0?=w2241:bool)
        n765 = case shown="True" w2241 {
          tunnel: w2248 -> [_ w2277]
          tunnel: w2247 -> [w2250 w2278]
          tunnel: [w2250 w2276] -> w2246
          tunnel: w2245 -> [_ w2273]
          tunnel: w2244 -> [_ w2272]
          tunnel: w2243 -> [_ w2262]
          tunnel: w2240 -> [_ w2271]
          tunnel: w2237 -> [w2249 w2268]
          tunnel: [w2249 w2267] -> w2236
          tunnel: w2235 -> [_ w2266]
          tunnel: w2234 -> [_ w2265]
          tunnel: w2233 -> [_ w2260]
          tunnel: w2231 -> [_ w2258]
          tunnel: w2230 -> [_ w2256]
          tunnel: w2229 -> [_ _]
          tunnel: w2228 -> [_ _]
          tunnel: w2227 -> [_ _]
          frame False {
          }
          frame True {
            # "True: Last Frame of frame accum"
            # "Current Line in Frame Accum"
            # "Current Line In Frame"
            n766 = Increment(x=w2268) -> (x+1=w2261:u32)
            n767 = Dequeue Element(queue=w2271) -> (element=w2284:u64[])  [unwired: 2 in, 3 out]
            n768 = Equal?(x=w2261, y=w2265) -> (x = y?=w2270:bool)
            n769 = Greater?(x=w2261, y=w2266) -> (0:w2263:bool)
            n770 = Greater?(x=w2261, y=w2260) -> (0:w2259:bool)
            n771 = Split Number(x=w2284) -> (hi(x)=w2285:u32[], lo(x)=w2283:u32[])
            n772 = Split Number(x=w2285) -> (lo(x)=w2251:u16[])  [unwired: 1 out]
            n773 = Split Number(x=w2283) -> (hi(x)=w2252:u16[])  [unwired: 1 out]
            n774 = Select(t=u32 0, s=w2270, f=w2261) -> (s? t:f=w2267:u32)
            n775 = Increment(x=w2278) -> (x+1=w2280:i32)
            n776 = Equal?(x=w2277, y=w2278) -> (x = y?=w2279:bool)
            n777 = To Single Precision Float(number=w2251) -> (single precision float=w2255:sgl[])
            n778 = To Single Precision Float(number=w2252) -> (single precision float=w2254:sgl[])
            n779 = Select(t=0, s=w2279, f=w2280) -> (s? t:f=w2276:i32)
            n780 = Add(x=w2255, y=w2254) -> (x+y=w2253:sgl[])
            n781 = Build Array(0, w2278, w2277, w2278) -> (w2275:i32[])
            n782 = case shown="False" w2259 {
              tunnel: [w2293 w2299] -> w2274
              tunnel: w2275 -> [_ w2297]
              tunnel: w2272 -> [w2292 w2296]
              tunnel: w2258 -> [w2291 w2295]
              tunnel: [w2291 w2295] -> w2257
              tunnel: w2253 -> [w2290 w2294]
              frame False {
                n783 = Divide(x=w2290, y=w2292) -> (x/y=w2293:sgl[])
              }
              frame True {
                n784 = call "IMAQ GetPixelLine"("Line Coordinates"=w2297, "Image"=w2295) -> ("Pixels Line (Float)"=w2298:sgl[])  [unwired: 2 in, 4 out]
                n785 = Divide(x=w2294, y=w2296) -> (x/y=w2300:sgl[])
                n786 = Add(x=w2298, y=w2300) -> (x+y=w2299:sgl[])
              }
            }
            n787 = call "IMAQ SetPixelLine"("Pixels Line (Float)"=w2274, "Line Coordinates"=w2275, "Image"=w2257) -> ()  [unwired: 7 in, 2 out]
            n788 = And(x=w2263, y=w2262) -> (x .and. y?=w2264:bool)
            n789 = case shown="True" w2264 {
              tunnel: w2274 -> [_ w2289]
              tunnel: w2273 -> [_ w2287]
              tunnel: w2256 -> [_ w2286]
              frame False {
              }
              frame True {
                n790 = Write to Binary File(file (use dialog)=w2286, data=w2289, 5:FALSE ("prepend array or string size? (T)"), 9:w2287) -> ()  [unwired: 2 in, 3 out]
              }
            }
          }
        }
      }
    }
    frame 23 {
      n791 = while {
        shift-right: [w2336] -> _
        shift-left: 0 -> [w2337]
        tunnel: w2315 -> [w2338]
        tunnel: w2314 -> [w2335]
        tunnel: w2313 -> [w2334]
        tunnel: w2312 -> [w2333]
        tunnel: w2311 -> [w2329]
        shift-right: [w2326] -> _
        shift-left: u32 0 -> [w2327]
        tunnel: w2309 -> [w2325]
        tunnel: w2308 -> [w2324]
        tunnel: w2307 -> [w2323]
        tunnel: w2306 -> [w2322]
        tunnel: w2301 -> [w2321]
        tunnel: w2305 -> [w2320]
        tunnel: w2304 -> [w2319]
        tunnel: w2303 -> [w2318]
        tunnel: w2302 -> [w2317]
        stop <- w2328 stop-if-true
        n792 = Get Queue Status(queue=w2322) -> (queue out=w2330:refnum<queue>, # elements in queue=w2332:i32)  [unwired: 2 in, 6 out]
        n793 = Get Notifier Status(notifier=w2329) -> (current notification=w2328:bool)  [unwired: 1 in, 4 out]
        n794 = Greater Than 0?(x=w2332) -> (x > 0?=w2331:bool)
        n795 = case shown="True" w2331 {
          tunnel: w2338 -> [_ w2369]
          tunnel: w2337 -> [w2340 w2370]
          tunnel: [w2340 w2368] -> w2336
          tunnel: w2335 -> [_ w2365]
          tunnel: w2334 -> [_ w2364]
          tunnel: w2333 -> [_ w2354]
          tunnel: w2330 -> [_ w2363]
          tunnel: w2327 -> [w2339 w2360]
          tunnel: [w2339 w2359] -> w2326
          tunnel: w2325 -> [_ w2358]
          tunnel: w2324 -> [_ w2357]
          tunnel: w2323 -> [_ w2352]
          tunnel: w2321 -> [_ w2350]
          tunnel: w2320 -> [_ w2348]
          tunnel: w2319 -> [_ _]
          tunnel: w2318 -> [_ _]
          tunnel: w2317 -> [_ _]
          frame False {
          }
          frame True {
            # "True: Last Frame of frame accum"
            # "Current Line in Frame Accum"
            # "Current Line In Frame"
            n796 = Increment(x=w2360) -> (x+1=w2353:u32)
            n797 = Dequeue Element(queue=w2363) -> (element=w2376:u64[])  [unwired: 2 in, 3 out]
            n798 = Equal?(x=w2353, y=w2357) -> (x = y?=w2362:bool)
            n799 = Greater?(x=w2353, y=w2358) -> (0:w2355:bool)
            n800 = Greater?(x=w2353, y=w2352) -> (0:w2351:bool)
            n801 = Split Number(x=w2376) -> (hi(x)=w2377:u32[], lo(x)=w2375:u32[])
            n802 = Split Number(x=w2377) -> (hi(x)=w2346:u16[], lo(x)=w2345:u16[])
            n803 = Split Number(x=w2375) -> (hi(x)=w2347:u16[])  [unwired: 1 out]
            n804 = Select(t=u32 0, s=w2362, f=w2353) -> (s? t:f=w2359:u32)
            n805 = Increment(x=w2370) -> (x+1=w2372:i32)
            n806 = Equal?(x=w2369, y=w2370) -> (x = y?=w2371:bool)
            n807 = To Single Precision Float(number=w2346) -> (single precision float=w2344:sgl[])
            n808 = To Single Precision Float(number=w2345) -> (single precision float=w2342:sgl[])
            n809 = To Single Precision Float(number=w2347) -> (single precision float=w2343:sgl[])
            n810 = Select(t=0, s=w2371, f=w2372) -> (s? t:f=w2368:i32)
            n811 = Compound Arithmetic op=ADD(w2344, w2342, w2343) -> (w2341:sgl[])
            n812 = Build Array(0, w2370, w2369, w2370) -> (w2367:i32[])
            n813 = case shown="False" w2351 {
              tunnel: [w2385 w2391] -> w2366
              tunnel: w2367 -> [_ w2389]
              tunnel: w2364 -> [w2384 w2388]
              tunnel: w2350 -> [w2383 w2387]
              tunnel: [w2383 w2387] -> w2349
              tunnel: w2341 -> [w2382 w2386]
              frame False {
                n814 = Divide(x=w2382, y=w2384) -> (x/y=w2385:sgl[])
              }
              frame True {
                n815 = call "IMAQ GetPixelLine"("Line Coordinates"=w2389, "Image"=w2387) -> ("Pixels Line (Float)"=w2390:sgl[])  [unwired: 2 in, 4 out]
                n816 = Divide(x=w2386, y=w2388) -> (x/y=w2392:sgl[])
                n817 = Add(x=w2390, y=w2392) -> (x+y=w2391:sgl[])
              }
            }
            n818 = call "IMAQ SetPixelLine"("Pixels Line (Float)"=w2366, "Line Coordinates"=w2367, "Image"=w2349) -> ()  [unwired: 7 in, 2 out]
            n819 = And(x=w2355, y=w2354) -> (x .and. y?=w2356:bool)
            n820 = case shown="True" w2356 {
              tunnel: w2366 -> [_ w2381]
              tunnel: w2365 -> [_ w2379]
              tunnel: w2348 -> [_ w2378]
              frame False {
              }
              frame True {
                n821 = Write to Binary File(file (use dialog)=w2378, data=w2381, 5:FALSE ("prepend array or string size? (T)"), 9:w2379) -> ()  [unwired: 2 in, 3 out]
              }
            }
          }
        }
      }
    }
    frame 25 {
      n822 = while {
        shift-right: [w2428] -> _
        shift-left: 0 -> [w2429]
        tunnel: w2407 -> [w2430]
        tunnel: w2406 -> [w2427]
        tunnel: w2405 -> [w2426]
        tunnel: w2404 -> [w2425]
        tunnel: w2403 -> [w2421]
        shift-right: [w2418] -> _
        shift-left: u32 0 -> [w2419]
        tunnel: w2401 -> [w2417]
        tunnel: w2400 -> [w2416]
        tunnel: w2399 -> [w2415]
        tunnel: w2398 -> [w2414]
        tunnel: w2393 -> [w2413]
        tunnel: w2397 -> [w2412]
        tunnel: w2396 -> [w2411]
        tunnel: w2395 -> [w2410]
        tunnel: w2394 -> [w2409]
        stop <- w2420 stop-if-true
        n823 = Get Queue Status(queue=w2414) -> (queue out=w2422:refnum<queue>, # elements in queue=w2424:i32)  [unwired: 2 in, 6 out]
        n824 = Get Notifier Status(notifier=w2421) -> (current notification=w2420:bool)  [unwired: 1 in, 4 out]
        n825 = Greater Than 0?(x=w2424) -> (x > 0?=w2423:bool)
        n826 = case shown="True" w2423 {
          tunnel: w2430 -> [_ w2459]
          tunnel: w2429 -> [w2432 w2460]
          tunnel: [w2432 w2458] -> w2428
          tunnel: w2427 -> [_ w2455]
          tunnel: w2426 -> [_ w2454]
          tunnel: w2425 -> [_ w2444]
          tunnel: w2422 -> [_ w2453]
          tunnel: w2419 -> [w2431 w2450]
          tunnel: [w2431 w2449] -> w2418
          tunnel: w2417 -> [_ w2448]
          tunnel: w2416 -> [_ w2447]
          tunnel: w2415 -> [_ w2442]
          tunnel: w2413 -> [_ w2440]
          tunnel: w2412 -> [_ w2438]
          tunnel: w2411 -> [_ _]
          tunnel: w2410 -> [_ _]
          tunnel: w2409 -> [_ _]
          frame False {
          }
          frame True {
            # "True: Last Frame of frame accum"
            # "Current Line in Frame Accum"
            # "Current Line In Frame"
            n827 = Increment(x=w2450) -> (x+1=w2443:u32)
            n828 = Dequeue Element(queue=w2453) -> (element=w2466:u64[])  [unwired: 2 in, 3 out]
            n829 = Equal?(x=w2443, y=w2447) -> (x = y?=w2452:bool)
            n830 = Greater?(x=w2443, y=w2448) -> (0:w2445:bool)
            n831 = Greater?(x=w2443, y=w2442) -> (0:w2441:bool)
            n832 = Split Number(x=w2466) -> (hi(x)=w2467:u32[], lo(x)=w2465:u32[])
            n833 = Split Number(x=w2467) -> (hi(x)=w2433:u16[])  [unwired: 1 out]
            n834 = Split Number(x=w2465) -> (lo(x)=w2434:u16[])  [unwired: 1 out]
            n835 = Select(t=u32 0, s=w2452, f=w2443) -> (s? t:f=w2449:u32)
            n836 = Increment(x=w2460) -> (x+1=w2462:i32)
            n837 = Equal?(x=w2459, y=w2460) -> (x = y?=w2461:bool)
            n838 = To Single Precision Float(number=w2433) -> (single precision float=w2437:sgl[])
            n839 = To Single Precision Float(number=w2434) -> (single precision float=w2436:sgl[])
            n840 = Select(t=0, s=w2461, f=w2462) -> (s? t:f=w2458:i32)
            n841 = Add(x=w2437, y=w2436) -> (x+y=w2435:sgl[])
            n842 = Build Array(0, w2460, w2459, w2460) -> (w2457:i32[])
            n843 = case shown="False" w2441 {
              tunnel: [w2475 w2481] -> w2456
              tunnel: w2457 -> [_ w2479]
              tunnel: w2454 -> [w2474 w2478]
              tunnel: w2440 -> [w2473 w2477]
              tunnel: [w2473 w2477] -> w2439
              tunnel: w2435 -> [w2472 w2476]
              frame False {
                n844 = Divide(x=w2472, y=w2474) -> (x/y=w2475:sgl[])
              }
              frame True {
                n845 = call "IMAQ GetPixelLine"("Line Coordinates"=w2479, "Image"=w2477) -> ("Pixels Line (Float)"=w2480:sgl[])  [unwired: 2 in, 4 out]
                n846 = Divide(x=w2476, y=w2478) -> (x/y=w2482:sgl[])
                n847 = Add(x=w2480, y=w2482) -> (x+y=w2481:sgl[])
              }
            }
            n848 = call "IMAQ SetPixelLine"("Pixels Line (Float)"=w2456, "Line Coordinates"=w2457, "Image"=w2439) -> ()  [unwired: 7 in, 2 out]
            n849 = And(x=w2445, y=w2444) -> (x .and. y?=w2446:bool)
            n850 = case shown="True" w2446 {
              tunnel: w2456 -> [_ w2471]
              tunnel: w2455 -> [_ w2469]
              tunnel: w2438 -> [_ w2468]
              frame False {
              }
              frame True {
                n851 = Write to Binary File(file (use dialog)=w2468, data=w2471, 5:FALSE ("prepend array or string size? (T)"), 9:w2469) -> ()  [unwired: 2 in, 3 out]
              }
            }
          }
        }
      }
    }
    frame 26 {
      n852 = while {
        shift-right: [w2518] -> _
        shift-left: 0 -> [w2519]
        tunnel: w2497 -> [w2520]
        tunnel: w2496 -> [w2517]
        tunnel: w2495 -> [w2516]
        tunnel: w2494 -> [w2515]
        tunnel: w2493 -> [w2511]
        shift-right: [w2508] -> _
        shift-left: u32 0 -> [w2509]
        tunnel: w2491 -> [w2507]
        tunnel: w2490 -> [w2506]
        tunnel: w2489 -> [w2505]
        tunnel: w2488 -> [w2504]
        tunnel: w2483 -> [w2503]
        tunnel: w2487 -> [w2502]
        tunnel: w2486 -> [w2501]
        tunnel: w2485 -> [w2500]
        tunnel: w2484 -> [w2499]
        stop <- w2510 stop-if-true
        n853 = Get Queue Status(queue=w2504) -> (queue out=w2512:refnum<queue>, # elements in queue=w2514:i32)  [unwired: 2 in, 6 out]
        n854 = Get Notifier Status(notifier=w2511) -> (current notification=w2510:bool)  [unwired: 1 in, 4 out]
        n855 = Greater Than 0?(x=w2514) -> (x > 0?=w2513:bool)
        n856 = case shown="True" w2513 {
          tunnel: w2520 -> [_ w2549]
          tunnel: w2519 -> [w2522 w2550]
          tunnel: [w2522 w2548] -> w2518
          tunnel: w2517 -> [_ w2545]
          tunnel: w2516 -> [_ w2544]
          tunnel: w2515 -> [_ w2534]
          tunnel: w2512 -> [_ w2543]
          tunnel: w2509 -> [w2521 w2540]
          tunnel: [w2521 w2539] -> w2508
          tunnel: w2507 -> [_ w2538]
          tunnel: w2506 -> [_ w2537]
          tunnel: w2505 -> [_ w2532]
          tunnel: w2503 -> [_ w2530]
          tunnel: w2502 -> [_ w2528]
          tunnel: w2501 -> [_ _]
          tunnel: w2500 -> [_ _]
          tunnel: w2499 -> [_ _]
          frame False {
          }
          frame True {
            # "True: Last Frame of frame accum"
            # "Current Line in Frame Accum"
            # "Current Line In Frame"
            n857 = Increment(x=w2540) -> (x+1=w2533:u32)
            n858 = Dequeue Element(queue=w2543) -> (element=w2556:u64[])  [unwired: 2 in, 3 out]
            n859 = Equal?(x=w2533, y=w2537) -> (x = y?=w2542:bool)
            n860 = Greater?(x=w2533, y=w2538) -> (0:w2535:bool)
            n861 = Greater?(x=w2533, y=w2532) -> (0:w2531:bool)
            n862 = Split Number(x=w2556) -> (hi(x)=w2557:u32[], lo(x)=w2555:u32[])
            n863 = Split Number(x=w2557) -> (lo(x)=w2524:u16[])  [unwired: 1 out]
            n864 = Split Number(x=w2555) -> (lo(x)=w2523:u16[])  [unwired: 1 out]
            n865 = Select(t=u32 0, s=w2542, f=w2533) -> (s? t:f=w2539:u32)
            n866 = Increment(x=w2550) -> (x+1=w2552:i32)
            n867 = Equal?(x=w2549, y=w2550) -> (x = y?=w2551:bool)
            n868 = To Single Precision Float(number=w2524) -> (single precision float=w2527:sgl[])
            n869 = To Single Precision Float(number=w2523) -> (single precision float=w2526:sgl[])
            n870 = Select(t=0, s=w2551, f=w2552) -> (s? t:f=w2548:i32)
            n871 = Add(x=w2527, y=w2526) -> (x+y=w2525:sgl[])
            n872 = Build Array(0, w2550, w2549, w2550) -> (w2547:i32[])
            n873 = case shown="False" w2531 {
              tunnel: [w2565 w2571] -> w2546
              tunnel: w2547 -> [_ w2569]
              tunnel: w2544 -> [w2564 w2568]
              tunnel: w2530 -> [w2563 w2567]
              tunnel: [w2563 w2567] -> w2529
              tunnel: w2525 -> [w2562 w2566]
              frame False {
                n874 = Divide(x=w2562, y=w2564) -> (x/y=w2565:sgl[])
              }
              frame True {
                n875 = call "IMAQ GetPixelLine"("Line Coordinates"=w2569, "Image"=w2567) -> ("Pixels Line (Float)"=w2570:sgl[])  [unwired: 2 in, 4 out]
                n876 = Divide(x=w2566, y=w2568) -> (x/y=w2572:sgl[])
                n877 = Add(x=w2570, y=w2572) -> (x+y=w2571:sgl[])
              }
            }
            n878 = call "IMAQ SetPixelLine"("Pixels Line (Float)"=w2546, "Line Coordinates"=w2547, "Image"=w2529) -> ()  [unwired: 7 in, 2 out]
            n879 = And(x=w2535, y=w2534) -> (x .and. y?=w2536:bool)
            n880 = case shown="True" w2536 {
              tunnel: w2546 -> [_ w2561]
              tunnel: w2545 -> [_ w2559]
              tunnel: w2528 -> [_ w2558]
              frame False {
              }
              frame True {
                n881 = Write to Binary File(file (use dialog)=w2558, data=w2561, 5:FALSE ("prepend array or string size? (T)"), 9:w2559) -> ()  [unwired: 2 in, 3 out]
              }
            }
          }
        }
      }
    }
    frame 27 {
      n882 = while {
        shift-right: [w2608] -> _
        shift-left: 0 -> [w2609]
        tunnel: w2587 -> [w2610]
        tunnel: w2586 -> [w2607]
        tunnel: w2585 -> [w2606]
        tunnel: w2584 -> [w2605]
        tunnel: w2583 -> [w2601]
        shift-right: [w2598] -> _
        shift-left: u32 0 -> [w2599]
        tunnel: w2581 -> [w2597]
        tunnel: w2580 -> [w2596]
        tunnel: w2579 -> [w2595]
        tunnel: w2578 -> [w2594]
        tunnel: w2573 -> [w2593]
        tunnel: w2577 -> [w2592]
        tunnel: w2576 -> [w2591]
        tunnel: w2575 -> [w2590]
        tunnel: w2574 -> [w2589]
        stop <- w2600 stop-if-true
        n883 = Get Queue Status(queue=w2594) -> (queue out=w2602:refnum<queue>, # elements in queue=w2604:i32)  [unwired: 2 in, 6 out]
        n884 = Get Notifier Status(notifier=w2601) -> (current notification=w2600:bool)  [unwired: 1 in, 4 out]
        n885 = Greater Than 0?(x=w2604) -> (x > 0?=w2603:bool)
        n886 = case shown="True" w2603 {
          tunnel: w2610 -> [_ w2641]
          tunnel: w2609 -> [w2612 w2642]
          tunnel: [w2612 w2640] -> w2608
          tunnel: w2607 -> [_ w2637]
          tunnel: w2606 -> [_ w2636]
          tunnel: w2605 -> [_ w2626]
          tunnel: w2602 -> [_ w2635]
          tunnel: w2599 -> [w2611 w2632]
          tunnel: [w2611 w2631] -> w2598
          tunnel: w2597 -> [_ w2630]
          tunnel: w2596 -> [_ w2629]
          tunnel: w2595 -> [_ w2624]
          tunnel: w2593 -> [_ w2622]
          tunnel: w2592 -> [_ w2620]
          tunnel: w2591 -> [_ _]
          tunnel: w2590 -> [_ _]
          tunnel: w2589 -> [_ _]
          frame False {
          }
          frame True {
            # "True: Last Frame of frame accum"
            # "Current Line in Frame Accum"
            # "Current Line In Frame"
            n887 = Increment(x=w2632) -> (x+1=w2625:u32)
            n888 = Dequeue Element(queue=w2635) -> (element=w2648:u64[])  [unwired: 2 in, 3 out]
            n889 = Equal?(x=w2625, y=w2629) -> (x = y?=w2634:bool)
            n890 = Greater?(x=w2625, y=w2630) -> (0:w2627:bool)
            n891 = Greater?(x=w2625, y=w2624) -> (0:w2623:bool)
            n892 = Split Number(x=w2648) -> (hi(x)=w2649:u32[], lo(x)=w2647:u32[])
            n893 = Split Number(x=w2649) -> (hi(x)=w2619:u16[], lo(x)=w2618:u16[])
            n894 = Split Number(x=w2647) -> (lo(x)=w2613:u16[])  [unwired: 1 out]
            n895 = Select(t=u32 0, s=w2634, f=w2625) -> (s? t:f=w2631:u32)
            n896 = Increment(x=w2642) -> (x+1=w2644:i32)
            n897 = Equal?(x=w2641, y=w2642) -> (x = y?=w2643:bool)
            n898 = To Single Precision Float(number=w2619) -> (single precision float=w2617:sgl[])
            n899 = To Single Precision Float(number=w2618) -> (single precision float=w2615:sgl[])
            n900 = To Single Precision Float(number=w2613) -> (single precision float=w2616:sgl[])
            n901 = Select(t=0, s=w2643, f=w2644) -> (s? t:f=w2640:i32)
            n902 = Compound Arithmetic op=ADD(w2617, w2615, w2616) -> (w2614:sgl[])
            n903 = Build Array(0, w2642, w2641, w2642) -> (w2639:i32[])
            n904 = case shown="False" w2623 {
              tunnel: [w2657 w2663] -> w2638
              tunnel: w2639 -> [_ w2661]
              tunnel: w2636 -> [w2656 w2660]
              tunnel: w2622 -> [w2655 w2659]
              tunnel: [w2655 w2659] -> w2621
              tunnel: w2614 -> [w2654 w2658]
              frame False {
                n905 = Divide(x=w2654, y=w2656) -> (x/y=w2657:sgl[])
              }
              frame True {
                n906 = call "IMAQ GetPixelLine"("Line Coordinates"=w2661, "Image"=w2659) -> ("Pixels Line (Float)"=w2662:sgl[])  [unwired: 2 in, 4 out]
                n907 = Divide(x=w2658, y=w2660) -> (x/y=w2664:sgl[])
                n908 = Add(x=w2662, y=w2664) -> (x+y=w2663:sgl[])
              }
            }
            n909 = call "IMAQ SetPixelLine"("Pixels Line (Float)"=w2638, "Line Coordinates"=w2639, "Image"=w2621) -> ()  [unwired: 7 in, 2 out]
            n910 = And(x=w2627, y=w2626) -> (x .and. y?=w2628:bool)
            n911 = case shown="True" w2628 {
              tunnel: w2638 -> [_ w2653]
              tunnel: w2637 -> [_ w2651]
              tunnel: w2620 -> [_ w2650]
              frame False {
              }
              frame True {
                n912 = Write to Binary File(file (use dialog)=w2650, data=w2653, 5:FALSE ("prepend array or string size? (T)"), 9:w2651) -> ()  [unwired: 2 in, 3 out]
              }
            }
          }
        }
      }
    }
    frame 28 {
      n913 = while {
        shift-right: [w2700] -> _
        shift-left: 0 -> [w2701]
        tunnel: w2679 -> [w2702]
        tunnel: w2678 -> [w2699]
        tunnel: w2677 -> [w2698]
        tunnel: w2676 -> [w2697]
        tunnel: w2675 -> [w2693]
        shift-right: [w2690] -> _
        shift-left: u32 0 -> [w2691]
        tunnel: w2673 -> [w2689]
        tunnel: w2672 -> [w2688]
        tunnel: w2671 -> [w2687]
        tunnel: w2670 -> [w2686]
        tunnel: w2665 -> [w2685]
        tunnel: w2669 -> [w2684]
        tunnel: w2668 -> [w2683]
        tunnel: w2667 -> [w2682]
        tunnel: w2666 -> [w2681]
        stop <- w2692 stop-if-true
        n914 = Get Queue Status(queue=w2686) -> (queue out=w2694:refnum<queue>, # elements in queue=w2696:i32)  [unwired: 2 in, 6 out]
        n915 = Get Notifier Status(notifier=w2693) -> (current notification=w2692:bool)  [unwired: 1 in, 4 out]
        n916 = Greater Than 0?(x=w2696) -> (x > 0?=w2695:bool)
        n917 = case shown="True" w2695 {
          tunnel: w2702 -> [_ w2731]
          tunnel: w2701 -> [w2704 w2732]
          tunnel: [w2704 w2730] -> w2700
          tunnel: w2699 -> [_ w2727]
          tunnel: w2698 -> [_ w2726]
          tunnel: w2697 -> [_ w2716]
          tunnel: w2694 -> [_ w2725]
          tunnel: w2691 -> [w2703 w2722]
          tunnel: [w2703 w2721] -> w2690
          tunnel: w2689 -> [_ w2720]
          tunnel: w2688 -> [_ w2719]
          tunnel: w2687 -> [_ w2714]
          tunnel: w2685 -> [_ w2712]
          tunnel: w2684 -> [_ w2710]
          tunnel: w2683 -> [_ _]
          tunnel: w2682 -> [_ _]
          tunnel: w2681 -> [_ _]
          frame False {
          }
          frame True {
            # "True: Last Frame of frame accum"
            # "Current Line in Frame Accum"
            # "Current Line In Frame"
            n918 = Increment(x=w2722) -> (x+1=w2715:u32)
            n919 = Dequeue Element(queue=w2725) -> (element=w2738:u64[])  [unwired: 2 in, 3 out]
            n920 = Equal?(x=w2715, y=w2719) -> (x = y?=w2724:bool)
            n921 = Greater?(x=w2715, y=w2720) -> (0:w2717:bool)
            n922 = Greater?(x=w2715, y=w2714) -> (0:w2713:bool)
            n923 = Split Number(x=w2738) -> (lo(x)=w2737:u32[])  [unwired: 1 out]
            n924 = Split Number(x=w2737) -> (hi(x)=w2705:u16[], lo(x)=w2706:u16[])
            n925 = Select(t=u32 0, s=w2724, f=w2715) -> (s? t:f=w2721:u32)
            n926 = Increment(x=w2732) -> (x+1=w2734:i32)
            n927 = Equal?(x=w2731, y=w2732) -> (x = y?=w2733:bool)
            n928 = To Single Precision Float(number=w2705) -> (single precision float=w2709:sgl[])
            n929 = To Single Precision Float(number=w2706) -> (single precision float=w2708:sgl[])
            n930 = Select(t=0, s=w2733, f=w2734) -> (s? t:f=w2730:i32)
            n931 = Add(x=w2709, y=w2708) -> (x+y=w2707:sgl[])
            n932 = Build Array(0, w2732, w2731, w2732) -> (w2729:i32[])
            n933 = case shown="False" w2713 {
              tunnel: [w2746 w2752] -> w2728
              tunnel: w2729 -> [_ w2750]
              tunnel: w2726 -> [w2745 w2749]
              tunnel: w2712 -> [w2744 w2748]
              tunnel: [w2744 w2748] -> w2711
              tunnel: w2707 -> [w2743 w2747]
              frame False {
                n934 = Divide(x=w2743, y=w2745) -> (x/y=w2746:sgl[])
              }
              frame True {
                n935 = call "IMAQ GetPixelLine"("Line Coordinates"=w2750, "Image"=w2748) -> ("Pixels Line (Float)"=w2751:sgl[])  [unwired: 2 in, 4 out]
                n936 = Divide(x=w2747, y=w2749) -> (x/y=w2753:sgl[])
                n937 = Add(x=w2751, y=w2753) -> (x+y=w2752:sgl[])
              }
            }
            n938 = call "IMAQ SetPixelLine"("Pixels Line (Float)"=w2728, "Line Coordinates"=w2729, "Image"=w2711) -> ()  [unwired: 7 in, 2 out]
            n939 = And(x=w2717, y=w2716) -> (x .and. y?=w2718:bool)
            n940 = case shown="True" w2718 {
              tunnel: w2728 -> [_ w2742]
              tunnel: w2727 -> [_ w2740]
              tunnel: w2710 -> [_ w2739]
              frame False {
              }
              frame True {
                n941 = Write to Binary File(file (use dialog)=w2739, data=w2742, 5:FALSE ("prepend array or string size? (T)"), 9:w2740) -> ()  [unwired: 2 in, 3 out]
              }
            }
          }
        }
      }
    }
    frame 29 {
      n942 = while {
        shift-right: [w2789] -> _
        shift-left: 0 -> [w2790]
        tunnel: w2768 -> [w2791]
        tunnel: w2767 -> [w2788]
        tunnel: w2766 -> [w2787]
        tunnel: w2765 -> [w2786]
        tunnel: w2764 -> [w2782]
        shift-right: [w2779] -> _
        shift-left: u32 0 -> [w2780]
        tunnel: w2762 -> [w2778]
        tunnel: w2761 -> [w2777]
        tunnel: w2760 -> [w2776]
        tunnel: w2759 -> [w2775]
        tunnel: w2754 -> [w2774]
        tunnel: w2758 -> [w2773]
        tunnel: w2757 -> [w2772]
        tunnel: w2756 -> [w2771]
        tunnel: w2755 -> [w2770]
        stop <- w2781 stop-if-true
        n943 = Get Queue Status(queue=w2775) -> (queue out=w2783:refnum<queue>, # elements in queue=w2785:i32)  [unwired: 2 in, 6 out]
        n944 = Get Notifier Status(notifier=w2782) -> (current notification=w2781:bool)  [unwired: 1 in, 4 out]
        n945 = Greater Than 0?(x=w2785) -> (x > 0?=w2784:bool)
        n946 = case shown="True" w2784 {
          tunnel: w2791 -> [_ w2822]
          tunnel: w2790 -> [w2793 w2823]
          tunnel: [w2793 w2821] -> w2789
          tunnel: w2788 -> [_ w2818]
          tunnel: w2787 -> [_ w2817]
          tunnel: w2786 -> [_ w2807]
          tunnel: w2783 -> [_ w2816]
          tunnel: w2780 -> [w2792 w2813]
          tunnel: [w2792 w2812] -> w2779
          tunnel: w2778 -> [_ w2811]
          tunnel: w2777 -> [_ w2810]
          tunnel: w2776 -> [_ w2805]
          tunnel: w2774 -> [_ w2803]
          tunnel: w2773 -> [_ w2801]
          tunnel: w2772 -> [_ _]
          tunnel: w2771 -> [_ _]
          tunnel: w2770 -> [_ _]
          frame False {
          }
          frame True {
            # "True: Last Frame of frame accum"
            # "Current Line in Frame Accum"
            # "Current Line In Frame"
            n947 = Increment(x=w2813) -> (x+1=w2806:u32)
            n948 = Dequeue Element(queue=w2816) -> (element=w2829:u64[])  [unwired: 2 in, 3 out]
            n949 = Equal?(x=w2806, y=w2810) -> (x = y?=w2815:bool)
            n950 = Greater?(x=w2806, y=w2811) -> (0:w2808:bool)
            n951 = Greater?(x=w2806, y=w2805) -> (0:w2804:bool)
            n952 = Split Number(x=w2829) -> (hi(x)=w2830:u32[], lo(x)=w2828:u32[])
            n953 = Split Number(x=w2830) -> (hi(x)=w2800:u16[])  [unwired: 1 out]
            n954 = Split Number(x=w2828) -> (hi(x)=w2795:u16[], lo(x)=w2794:u16[])
            n955 = Select(t=u32 0, s=w2815, f=w2806) -> (s? t:f=w2812:u32)
            n956 = Increment(x=w2823) -> (x+1=w2825:i32)
            n957 = Equal?(x=w2822, y=w2823) -> (x = y?=w2824:bool)
            n958 = To Single Precision Float(number=w2800) -> (single precision float=w2799:sgl[])
            n959 = To Single Precision Float(number=w2795) -> (single precision float=w2797:sgl[])
            n960 = To Single Precision Float(number=w2794) -> (single precision float=w2798:sgl[])
            n961 = Select(t=0, s=w2824, f=w2825) -> (s? t:f=w2821:i32)
            n962 = Compound Arithmetic op=ADD(w2799, w2797, w2798) -> (w2796:sgl[])
            n963 = Build Array(0, w2823, w2822, w2823) -> (w2820:i32[])
            n964 = case shown="False" w2804 {
              tunnel: [w2838 w2844] -> w2819
              tunnel: w2820 -> [_ w2842]
              tunnel: w2817 -> [w2837 w2841]
              tunnel: w2803 -> [w2836 w2840]
              tunnel: [w2836 w2840] -> w2802
              tunnel: w2796 -> [w2835 w2839]
              frame False {
                n965 = Divide(x=w2835, y=w2837) -> (x/y=w2838:sgl[])
              }
              frame True {
                n966 = call "IMAQ GetPixelLine"("Line Coordinates"=w2842, "Image"=w2840) -> ("Pixels Line (Float)"=w2843:sgl[])  [unwired: 2 in, 4 out]
                n967 = Divide(x=w2839, y=w2841) -> (x/y=w2845:sgl[])
                n968 = Add(x=w2843, y=w2845) -> (x+y=w2844:sgl[])
              }
            }
            n969 = call "IMAQ SetPixelLine"("Pixels Line (Float)"=w2819, "Line Coordinates"=w2820, "Image"=w2802) -> ()  [unwired: 7 in, 2 out]
            n970 = And(x=w2808, y=w2807) -> (x .and. y?=w2809:bool)
            n971 = case shown="True" w2809 {
              tunnel: w2819 -> [_ w2834]
              tunnel: w2818 -> [_ w2832]
              tunnel: w2801 -> [_ w2831]
              frame False {
              }
              frame True {
                n972 = Write to Binary File(file (use dialog)=w2831, data=w2834, 5:FALSE ("prepend array or string size? (T)"), 9:w2832) -> ()  [unwired: 2 in, 3 out]
              }
            }
          }
        }
      }
    }
    frame 30 {
      n973 = while {
        shift-right: [w2881] -> _
        shift-left: 0 -> [w2882]
        tunnel: w2860 -> [w2883]
        tunnel: w2859 -> [w2880]
        tunnel: w2858 -> [w2879]
        tunnel: w2857 -> [w2878]
        tunnel: w2856 -> [w2874]
        shift-right: [w2871] -> _
        shift-left: u32 0 -> [w2872]
        tunnel: w2854 -> [w2870]
        tunnel: w2853 -> [w2869]
        tunnel: w2852 -> [w2868]
        tunnel: w2851 -> [w2867]
        tunnel: w2846 -> [w2866]
        tunnel: w2850 -> [w2865]
        tunnel: w2849 -> [w2864]
        tunnel: w2848 -> [w2863]
        tunnel: w2847 -> [w2862]
        stop <- w2873 stop-if-true
        n974 = Get Queue Status(queue=w2867) -> (queue out=w2875:refnum<queue>, # elements in queue=w2877:i32)  [unwired: 2 in, 6 out]
        n975 = Get Notifier Status(notifier=w2874) -> (current notification=w2873:bool)  [unwired: 1 in, 4 out]
        n976 = Greater Than 0?(x=w2877) -> (x > 0?=w2876:bool)
        n977 = case shown="True" w2876 {
          tunnel: w2883 -> [_ w2914]
          tunnel: w2882 -> [w2885 w2915]
          tunnel: [w2885 w2913] -> w2881
          tunnel: w2880 -> [_ w2910]
          tunnel: w2879 -> [_ w2909]
          tunnel: w2878 -> [_ w2899]
          tunnel: w2875 -> [_ w2908]
          tunnel: w2872 -> [w2884 w2905]
          tunnel: [w2884 w2904] -> w2871
          tunnel: w2870 -> [_ w2903]
          tunnel: w2869 -> [_ w2902]
          tunnel: w2868 -> [_ w2897]
          tunnel: w2866 -> [_ w2895]
          tunnel: w2865 -> [_ w2893]
          tunnel: w2864 -> [_ _]
          tunnel: w2863 -> [_ _]
          tunnel: w2862 -> [_ _]
          frame False {
          }
          frame True {
            # "True: Last Frame of frame accum"
            # "Current Line in Frame Accum"
            # "Current Line In Frame"
            n978 = Increment(x=w2905) -> (x+1=w2898:u32)
            n979 = Dequeue Element(queue=w2908) -> (element=w2921:u64[])  [unwired: 2 in, 3 out]
            n980 = Equal?(x=w2898, y=w2902) -> (x = y?=w2907:bool)
            n981 = Greater?(x=w2898, y=w2903) -> (0:w2900:bool)
            n982 = Greater?(x=w2898, y=w2897) -> (0:w2896:bool)
            n983 = Split Number(x=w2921) -> (hi(x)=w2922:u32[], lo(x)=w2920:u32[])
            n984 = Split Number(x=w2922) -> (lo(x)=w2886:u16[])  [unwired: 1 out]
            n985 = Split Number(x=w2920) -> (hi(x)=w2888:u16[], lo(x)=w2887:u16[])
            n986 = Select(t=u32 0, s=w2907, f=w2898) -> (s? t:f=w2904:u32)
            n987 = Increment(x=w2915) -> (x+1=w2917:i32)
            n988 = Equal?(x=w2914, y=w2915) -> (x = y?=w2916:bool)
            n989 = To Single Precision Float(number=w2886) -> (single precision float=w2892:sgl[])
            n990 = To Single Precision Float(number=w2888) -> (single precision float=w2890:sgl[])
            n991 = To Single Precision Float(number=w2887) -> (single precision float=w2891:sgl[])
            n992 = Select(t=0, s=w2916, f=w2917) -> (s? t:f=w2913:i32)
            n993 = Compound Arithmetic op=ADD(w2892, w2890, w2891) -> (w2889:sgl[])
            n994 = Build Array(0, w2915, w2914, w2915) -> (w2912:i32[])
            n995 = case shown="False" w2896 {
              tunnel: [w2930 w2936] -> w2911
              tunnel: w2912 -> [_ w2934]
              tunnel: w2909 -> [w2929 w2933]
              tunnel: w2895 -> [w2928 w2932]
              tunnel: [w2928 w2932] -> w2894
              tunnel: w2889 -> [w2927 w2931]
              frame False {
                n996 = Divide(x=w2927, y=w2929) -> (x/y=w2930:sgl[])
              }
              frame True {
                n997 = call "IMAQ GetPixelLine"("Line Coordinates"=w2934, "Image"=w2932) -> ("Pixels Line (Float)"=w2935:sgl[])  [unwired: 2 in, 4 out]
                n998 = Divide(x=w2931, y=w2933) -> (x/y=w2937:sgl[])
                n999 = Add(x=w2935, y=w2937) -> (x+y=w2936:sgl[])
              }
            }
            n1000 = call "IMAQ SetPixelLine"("Pixels Line (Float)"=w2911, "Line Coordinates"=w2912, "Image"=w2894) -> ()  [unwired: 7 in, 2 out]
            n1001 = And(x=w2900, y=w2899) -> (x .and. y?=w2901:bool)
            n1002 = case shown="True" w2901 {
              tunnel: w2911 -> [_ w2926]
              tunnel: w2910 -> [_ w2924]
              tunnel: w2893 -> [_ w2923]
              frame False {
              }
              frame True {
                n1003 = Write to Binary File(file (use dialog)=w2923, data=w2926, 5:FALSE ("prepend array or string size? (T)"), 9:w2924) -> ()  [unwired: 2 in, 3 out]
              }
            }
          }
        }
      }
    }
    frame 31 {
      n1004 = while {
        shift-right: [w2973] -> _
        shift-left: 0 -> [w2974]
        tunnel: w2952 -> [w2975]
        tunnel: w2951 -> [w2972]
        tunnel: w2950 -> [w2971]
        tunnel: w2949 -> [w2970]
        tunnel: w2948 -> [w2966]
        shift-right: [w2963] -> _
        shift-left: u32 0 -> [w2964]
        tunnel: w2946 -> [w2962]
        tunnel: w2945 -> [w2961]
        tunnel: w2944 -> [w2960]
        tunnel: w2943 -> [w2959]
        tunnel: w2938 -> [w2958]
        tunnel: w2942 -> [w2957]
        tunnel: w2941 -> [w2956]
        tunnel: w2940 -> [w2955]
        tunnel: w2939 -> [w2954]
        stop <- w2965 stop-if-true
        n1005 = Get Queue Status(queue=w2959) -> (queue out=w2967:refnum<queue>, # elements in queue=w2969:i32)  [unwired: 2 in, 6 out]
        n1006 = Get Notifier Status(notifier=w2966) -> (current notification=w2965:bool)  [unwired: 1 in, 4 out]
        n1007 = Greater Than 0?(x=w2969) -> (x > 0?=w2968:bool)
        n1008 = case shown="True" w2968 {
          tunnel: w2975 -> [_ w3008]
          tunnel: w2974 -> [w2977 w3009]
          tunnel: [w2977 w3007] -> w2973
          tunnel: w2972 -> [_ w3004]
          tunnel: w2971 -> [_ w3003]
          tunnel: w2970 -> [_ w2993]
          tunnel: w2967 -> [_ w3002]
          tunnel: w2964 -> [w2976 w2999]
          tunnel: [w2976 w2998] -> w2963
          tunnel: w2962 -> [_ w2997]
          tunnel: w2961 -> [_ w2996]
          tunnel: w2960 -> [_ w2991]
          tunnel: w2958 -> [_ w2989]
          tunnel: w2957 -> [_ w2987]
          tunnel: w2956 -> [_ _]
          tunnel: w2955 -> [_ _]
          tunnel: w2954 -> [_ _]
          frame False {
          }
          frame True {
            # "True: Last Frame of frame accum"
            # "Current Line in Frame Accum"
            # "Current Line In Frame"
            n1009 = Increment(x=w2999) -> (x+1=w2992:u32)
            n1010 = Dequeue Element(queue=w3002) -> (element=w3015:u64[])  [unwired: 2 in, 3 out]
            n1011 = Equal?(x=w2992, y=w2996) -> (x = y?=w3001:bool)
            n1012 = Greater?(x=w2992, y=w2997) -> (0:w2994:bool)
            n1013 = Greater?(x=w2992, y=w2991) -> (0:w2990:bool)
            n1014 = Split Number(x=w3015) -> (hi(x)=w3016:u32[], lo(x)=w3014:u32[])
            n1015 = Split Number(x=w3016) -> (hi(x)=w2981:u16[], lo(x)=w2980:u16[])
            n1016 = Split Number(x=w3014) -> (hi(x)=w2979:u16[], lo(x)=w2978:u16[])
            n1017 = Select(t=u32 0, s=w3001, f=w2992) -> (s? t:f=w2998:u32)
            n1018 = Increment(x=w3009) -> (x+1=w3011:i32)
            n1019 = Equal?(x=w3008, y=w3009) -> (x = y?=w3010:bool)
            n1020 = To Single Precision Float(number=w2981) -> (single precision float=w2986:sgl[])
            n1021 = To Single Precision Float(number=w2980) -> (single precision float=w2984:sgl[])
            n1022 = To Single Precision Float(number=w2979) -> (single precision float=w2985:sgl[])
            n1023 = To Single Precision Float(number=w2978) -> (single precision float=w2982:sgl[])
            n1024 = Select(t=0, s=w3010, f=w3011) -> (s? t:f=w3007:i32)
            n1025 = Compound Arithmetic op=ADD(w2986, w2984, w2985, w2982) -> (w2983:sgl[])
            n1026 = Build Array(0, w3009, w3008, w3009) -> (w3006:i32[])
            n1027 = case shown="False" w2990 {
              tunnel: [w3024 w3030] -> w3005
              tunnel: w3006 -> [_ w3028]
              tunnel: w3003 -> [w3023 w3027]
              tunnel: w2989 -> [w3022 w3026]
              tunnel: [w3022 w3026] -> w2988
              tunnel: w2983 -> [w3021 w3025]
              frame False {
                n1028 = Divide(x=w3021, y=w3023) -> (x/y=w3024:sgl[])
              }
              frame True {
                n1029 = call "IMAQ GetPixelLine"("Line Coordinates"=w3028, "Image"=w3026) -> ("Pixels Line (Float)"=w3029:sgl[])  [unwired: 2 in, 4 out]
                n1030 = Divide(x=w3025, y=w3027) -> (x/y=w3031:sgl[])
                n1031 = Add(x=w3029, y=w3031) -> (x+y=w3030:sgl[])
              }
            }
            n1032 = call "IMAQ SetPixelLine"("Pixels Line (Float)"=w3005, "Line Coordinates"=w3006, "Image"=w2988) -> ()  [unwired: 7 in, 2 out]
            n1033 = And(x=w2994, y=w2993) -> (x .and. y?=w2995:bool)
            n1034 = case shown="True" w2995 {
              tunnel: w3005 -> [_ w3020]
              tunnel: w3004 -> [_ w3018]
              tunnel: w2987 -> [_ w3017]
              frame False {
              }
              frame True {
                n1035 = Write to Binary File(file (use dialog)=w3017, data=w3020, 5:FALSE ("prepend array or string size? (T)"), 9:w3018) -> ()  [unwired: 2 in, 3 out]
              }
            }
          }
        }
      }
    }
  }
  n1036 = Flush Queue(queue=w20) -> (queue out=w64:refnum<queue>)  [unwired: 1 in, 2 out]
  n1037 = Release Queue(queue=w64) -> ()  [unwired: 2 in, 3 out]
  n1038 = while {
    tunnel: w78 -> [w3052]
    shift-right: [w3034] -> _
    shift-left: u32 0 -> [w3033]
    tunnel: w104 -> [w3032]
    shift-right: [w3048] -> _
    shift-left: FALSE -> [w3047]
    tunnel: w21 -> [w3046]
    shift-right: [w3044] -> _
    shift-left: u32 0 -> [w3045]
    tunnel: w99 -> [w3040]
    tunnel: w17 -> [w3037]
    tunnel: [w3035] -> w79
    shift-right: [w3036] -> w93
    shift-left: w39 -> [w3053]
    stop <- w3043 stop-if-true
    # "Total Lines Counter"
    n1039 = xnode "Invoke Method"("FPGA VI Reference In"=w3052, "Number of Elements"=w3033, "Timeout (ms)"=0) -> ("FPGA VI Reference Out"=w3035:refnum<k20>, "Data"=w3041:u64[], "Elements Remaining"=w3050:u32)  [unwired: 1 in, 1 out]
    n1040 = Get Notifier Status(notifier=w3053) -> (notifier out=w3036:refnum<notifier>, current notification=w3042:bool)  [unwired: 1 in, 3 out]
    n1041 = case shown="True" w3047 {
      tunnel: w3041 -> [_ w3056]
      tunnel: w3046 -> [_ w3062]
      tunnel: w3045 -> [w3055 w3059]
      tunnel: [w3055 w3060] -> w3044
      tunnel: [w3054 w3058] -> w3039
      tunnel: w3042 -> [w3054 _]
      tunnel: w3040 -> [_ w3057]
      frame False {
      }
      frame True {
        n1042 = Increment(x=w3059) -> (x+1=w3060:u32)
        n1043 = Enqueue Element(queue=w3062, element=w3056, timeout in ms (-1)=0) -> ()  [unwired: 1 in, 3 out]
        n1044 = Equal?(x=w3060, y=w3057) -> (x = y?=w3058:bool)
      }
    }
    n1045 = Greater Or Equal?(x=w3050, y=w3032) -> (x >= y?=w3048:bool)
    n1046 = Select(t=w3032, s=w3048, f=u32 0) -> (s? t:f=w3034:u32)
    n1047 = And(x=w3037, y=w3039) -> (x .and. y?=w3038:bool)
    n1048 = Or(x=w3038, y=w3042) -> (x .or. y?=w3043:bool)
  }
  n1049 = xnode "Close FPGA VI Reference"("FPGA VI Reference In"=w79) -> ()  [unwired: 1 in, 1 out]
  n1050 = Send Notification(notification=TRUE, notifier=w93) -> ()  [unwired: 1 in, 2 out]
